vi "Core_Chem_User_Interface_v2.0.vi"() -> ()   [LabVIEW 2014]
uses:
  C:/Program Files (x86)/National Instruments/LabVIEW 2014/examples/Data Communication/Network Streams/Simple Network Streams/support/Network Stream Command.ctl
  <vilib>/dex/Stream Element Allocation Mode.ctl
  <vilib>/Platform/TimedLoop/XDataNode/timing_clust.ctl
  <vilib>/Platform/TimedLoop/XDataNode/nitl_modes.ctl
  <vilib>/Platform/TimedLoop/XDataNode/wakeup.ctl
  <vilib>/Utility/tcp.llb/UDP Multicast Read-Only Open.vi
  <vilib>/platform/TimedLoop/XDataNode/XDataNode.xnode
  <vilib>/Platform/TimedLoop/XDataNode/XDNodeRunTimeDep.lvlib
  <vilib>/FTP/NI_FTP.lvlib
panel:
  out "SO2 Zeroing (Inflight)\nTime Remain (sec)":u32
  in  "eV6 User set time \n(Inflight) (sec)":i32=120
  in  "SO2 Inflight \nZeroing":bool
  out "Create folder error out 2":errorcluster
  out "Network to cRIO live status":bool
  out "Create folder error out":errorcluster
  in  "Confirm Flight Number":bool
  out "PRTAFT_UDP_In":string
  out "TWBOZO01":string
  out "CABOZO01":string
  out "TEIOZO01":string
  out "CHTSOO01":string
  out "CHFGGA01":string
  out "AL52CO01":string
  in  "Flight Number":string
  in  "Tab Control":T1(tab)
  out "FGGA preflight Des 17":string="Preflight - Start minimum 2 hours before take-off\n\n1. Ensure no bags/jackets are stowed on seat backs and behind seats in front of core chemistry rack at all times.\n\n2. Remove inlet covers if applicable.\n\n3. Connect Lilliput mini TFT/LCD VGA cable to FGGA VIDEO (back panel) and PS2 Keyboard/Mouse cables to FGGA Connectors (back panel). TFT/LCD screen kept in WAS/GAS rack Zargers Box. Keyboard/Mouse kept bottom of chemistry rack. (DO NOT disconnect PS2 cable). Connect TFT/LCD AC/DC PSU to 6026-8-98 Amphenol (SSP9) and make 230 Vac CB.\n\n4. Ensure all circuit breakers are pushed in, except 230Vac and 28Vdc, UPS switch off (down) and AL5002 CO Plasma Lamp switch off (down), WoW key to normal (horizontal).\n\n5. Wait for ALL network switches on the aircraft to be up and running before start-up. On the Flight Manager's Interface on the Flight Manager laptop, check SSP icons status (top row) should be all green.  \n\n6. Check AboutTime has synchronised laptop clock to aircraft timeservers (Filiberto/Gaston).\n\nClick the PowerUp Tab."
  out "FGGA preflight Des 16":string="PowerUp\n\n1.\tSSP9 forward face\tMake 3 CBs\n\n2.\tPWRDIST \t\tMake 230Vac CB \n                     Switch UPS On \t[UP]\n                     Make 28Vdc CB\n                     Check 28VDC OK Green Light comes on\n\n3.\tCore Chemistry e-Log\nComplete Core Chemistry e-Log in WordPad (Bnnn_CoreChemLog_v2.2), save on Flight Manager's laptop (192.168.101.180/      flt_folders/Bnnn); Fill in header with date, flight number and your name/initials.\n\n4. Wait for MFM flow rate to display non zero value.\n\n5.\tSAMPUMP\t\t\n - Switch WoW override key (vertical) to check pump starts, and MFM flowrate increase (>20 LPM) on the right hand plot. \n - Switch off WoW override\t\t\t\t [NORM, key horizontal]\n\nClick the 2B Ozone tab if operated, otherwise, click the UDP tab.\n\n\n"
  out "MFM":dbl(graph)
  in  "Ambient = OFF\nCabin = ON":bool
  out "FGGA preflight Des 15":string="2B Ozone Preflight\n\n1.\tSelect either Ambient or Cabin Air mode (default should be OFF for Ambient air mode).\n\n2. Check flowrate is greater than 2000 sccm on the right hand plot.\n\nClick the UDP tab."
  out "2B Ozone concentration":dbl(graph)
  out "2B Ozone flow rate":dbl(graph)
  out "2BOzone Event error out":errorcluster
  out "2BOzone command sender error out":errorcluster
  out "FGGA preflight Des 20":string="4. Check derived parameters in DECADES (192.168.101.110 & 192.168.101.108). 574 Ozone TEi49C; 588 CO AL5002; 611 SO2 TEi43i; 903 - 905 FGGA; 910 / 920 Ozone 2B."
  out "FGGA preflight Des 14":string="UDP Preflight\n1. Check all UDP packets are updating.  Unix time increasing by 1 sec (3rd parameter).\n2. Check flight number is correct.\n3. Confirm flight number and check it appears in the UDP packet (6th parameter). "
  in  "name":string="239.1.4.6"
  in  "Port":u16=50001
  out "FGGA":string
  out "CO":string
  out "TEi49 Ozone":string
  out "2B Cabin Ozone":string
  out "2B Ambient Ozone":string
  out "SO2":string
  out "Ozone Zeroing\nTime Remain (sec)":u32
  in  "Ozone Zeroing":bool
  out "TEI49C Sample Flow B":dbl(graph)
  out "TEi49C Concentration":dbl(graph)
  out "TEI49C Sample Flow A":dbl(graph)
  out "FGGA preflight Des 13":string="TEi49C Ozone PRE-FLIGHT - LAST ACTIONS BEFORE SEAT-BELTING DOWN (PRIOR TO ENGINES START)\n\n1. Ozone monitor zeroing\t\t[10 min minimum]\n\n\n2. Check TEi49C zero value and note down value in e-Log. \n"
  out "FGGA preflight Des 12":string="TEi49C Ozone Preflight\n\n1. Check nominal sample flowrate on both channels is ~0.7 LPM."
  out "Ozone Event error out":errorcluster
  out "Ozone command sender error out":errorcluster
  in  "Ozone UDP Time Offset":i32=1
  out "SO2 react pressure":dbl(graph)
  in  "Prepare SO2 Zero Gas":bool
  in  "Prepare SO2 Span Gas":bool
  in  "Auto Zeroing \ninterval (sec)":i32=600
  out "Next Auto Zero\nStarts in (sec)":u32
  out "Auto Zero\nIndicator":string="Auto Zero Inactive; Manual Zero Allow"
  out "SO2 Resume Zeroing\nCount down timer (sec)":u32
  in  "SO2 Pause\nAuto Zeroing":bool
  out "TEi43i Concentration scaled / raw":cluster{dbl, dbl}(graph)
  in  "SO2 Auto Zeroing":bool
  out "mean zero\ncal status":bool
  out "SO2 Sensitivity":dbl format="%.2g"
  out "SO2 Zero":dbl format="%.2g"
  in  "eV9 Flush User\nset time (sec)":i32=15
  in  "MFC_3 User Set Value":dbl=2.0
  in  "MFC_2 User Set Value":dbl=2.5
  in  "eV6 User\nset time (sec)":i32=600
  out "SO2 Flush\nTime Remain (sec)":u32
  out "TEI43i MFC3 Sample Flow":dbl(graph)
  out "TEI43C Sample Flow":dbl(graph)
  out "TEI43i MFC2 Cal Flow":dbl(graph)
  out "SO2 CAL/Zero\nTime Remain (sec)":u32
  out "SO2 Cal/Zero Flush\nTime Remain (sec)":u32
  in  "SO2 CAL/Zero":bool
  out "FGGA preflight Des 11":string="TEi43 SO2 Inflight Calibration & Zeroing"
  in  "SO2 GND Zeroing":bool
  out "SO2 Zeroing\nTime Remain (sec)":u32
  out "FGGA preflight Des 10":string="TEi43 SO2 PRE-FLIGHT - LAST ACTIONS BEFORE SEAT-BELTING DOWN (PRIOR TO ENGINES START)\n\n1. SO2 monitors zeroing\t\t[10 min minimum]\n\n2. Check TEi43i or TEi43C zero value and note down value in e-Log.\n\n3. Select required SO2 Span/Zero CAL gas at CALDECK front panel using quick connector.\n    For pre- and post-flight SO2 span calibrations select span gas. - Perform SO2 CAL\n    For in-flight SO2 (auto) zeroing, select zero air gas.\n\n4. Enable SO2 auto zeroing (if required) and check zeroing interval. "
  in  "SO2 Flush":bool
  out "FGGA preflight Des 9":string="TEi43 SO2 Preflight\n\n1. Check nominal sample flowrate is 2.0 LPM on the right hand plot.\n\nSO2 calibration gas purge - SO2 calibration cylinder locate at bottom of WAS Gas rack.\n\n2.\n\n\n3. Press SO2 flush button, MFC2 cal flow should increase to 2.5 SLPM.\nMonitor MFC2 flow rate to make sure the reading decreases from 2.5 SLPM to 0.0 SLPM.\nCheck pressure content and delivery gauges also reads zero.\nIf pressure content & delivery gauges do NOT read zero, press SO2 flush button again until they do.\n\n4. Quickly open and close cylinder valve 1.\n\n5. Repeat step 3) to 4) three times.\n\n6. Open cylinder valve 1, system is ready. Note down content pressure in elog.\n\n7."
  in  "eV9 flush User\nset time (sec)":i32=30
  in  "eV8 User\nset time (sec)":i32=60
  out "SO2 Event error out":errorcluster
  out "SO2 command sender \nerror out":errorcluster
  in  "SO2 UDP Time Offset":i32=1
  out "Lamp Temperature":dbl(graph)
  out "CO CAL Status":bool
  in  "CO CAL":bool
  out "FGGA preflight Des 8":string="CO Preflight and Inflight Calibrations\nHold down the CAL button for 2 secs then release, CAL status should then lit up.\nInflight calibration performed on 45 minutes interval or more frequently if lamp temperature > 35.5 degC."
  in  "Prepare Gases":bool
  out "FGGA preflight Des 7":string="AL5002 CO Preflight Checks\n\n1.\n\n2. Start CO Vacuum. NB: If there is problem with the software control, use manual override switch [up] on CALDECK front panel\n\n3. CO Checks - charts on the right hand side\n    Lamp Flow Controller ~ 40 ml/min\n    Monochromator Flow Controller ~ 30 ml/min\n    Fluorescence Cell Pressure ~ 7.5 Torr\n\nIf Lamp/Mono flows are low, manual valves (V1 -> V5) may still be shut, or pressure adjusting valves (ALREG1 & 2) have not been set > 2 bar\n\nIf Cell pressure is 10 Torr (max range), check that COPUMP is running and eV7 is opened (CO Vacuum eV7 is ON).\n\n4. Switch Plasma Lamp at the front panel UP\n\nDetector count rate (on 'Raw Signal' or F2 instrument touchscreen) should increase to >=10000 Hz within a minute.  Recycle plasma lamp switch (off/on) if no significant increase in count rate after 10 mins.  CO concentration should increase (100s ppb). \n     \n\n"
  in  "CO Vaccum (eV7)":bool
  out "Raw Signal":dbl(graph)
  out "CO Concentration":dbl(graph)
  out "Fluorescence Cell Pressure":dbl(graph)
  out "Monochromator Flow":dbl(graph)
  out "Lamp Flow Controller":dbl(graph)
  in  "CO UDP Time Offset":i32=1
  out "CO2 Pressure\nDelivery (PSIA)":dbl(slide) scale=0.0..100.0
  out "Std\nContent (barG)":dbl(slide) scale=0.0..220.0
  out "N2\nContent (barG)":dbl(slide) scale=0.0..220.0
  out "CO2\nContent (barG)":dbl(slide) scale=0.0..170.0
  out "CO Event error out":errorcluster
  out "CO command sender error out":errorcluster
  out "CO Zero":T2(array[cluster])
  out "CO Sensitivity":T3(array[cluster])
  out "Ring Down Time RDA & RDB":cluster{dbl, dbl}(graph)
  in  "Line Lock Setting Change":bool
  out "Cell temperature":dbl(graph)
  out "Cell pressure":dbl(graph)
  in  "Manual FGGA Pump":bool
  out "CO2":dbl(graph)
  out "CH4":dbl(graph)
  out "H2O":dbl(graph)
  out "WoW Flag":string="0"
  in  "FGGA pump\nsync to WoW":bool
  out "CH4 Dry":dbl(graph)
  out "CO2 Dry":dbl(graph)
  out "MFC1 Cal Flow":dbl(graph)
  out "Flush Target Tank\nTime Remain (sec)":u32
  out "Flush Low Tank\nTime Remain (sec)":u32
  out "Flush High Tank\nTime Remain (sec)":u32
  in  "Flush Target Tank":bool
  in  "Flush Low Tank":bool
  in  "Flush High Tank":bool
  in  "FGGA Restart":bool
  out "FGGA preflight Des 6":string="FGGA Instrument Controls"
  in  "High Cal":bool
  out "High Cal\nFlush Time Remain (sec)":u32
  out "High Cal\nCal Time Remain (sec)":u32
  in  "Low Cal":bool
  in  "Target Cal":bool
  in  "Span Cal - \nHigh Cal, CO Cal, Low Cal":bool
  out "Low Cal\nFlush Time Remain (sec)":u32
  out "Low Cal\nCal Time Remain (sec)":u32
  out "Target Cal\nFlush Time Remain (sec)":u32
  out "Target Cal\nCal Time Remain (sec)":u32
  in  "MFC_1 User Set Value":dbl=2.0
  out "FGGA preflight Des 5":string="FGGA Inflight Calibrations"
  out "FGGA preflight Des 4":string="FGGA Ground Preflight Checks\n\n1. Switch FGGA pump ON\n\n2. Check cavity pressure ~50 Torr\n\n3. Switch FGGA pump OFF\n\n4. Enable FGGA pump sync to WoW\n\n5.. Check Time Synchronisation\n\n6. Check CO2 & CH4 values\n\nIf CO2 & CH4 values are -1 ppm, follow the \nchange linelock settings procedure.\n\n\n\n\n\nLAST ACTION BEFORE SEAT-BELTING \nDOWN (PRIOR TO ENGINES START)\n\n1. Disconnect Monitor & stow away. Leave Keyboard & Mouse connected. Place keyboard at the bottom\nof the rack.\n\n"
  out "FGGA preflight Des 3":string="FGGA CAL Gas Purge\n\nFor each cylinder in gas stowage, check that,\n\n1. V1 Closed\n    V3 Closed\n    V4 Make sure arrow positioned downwards (i.e. flow points to gas line)\n\n2. V3 Open (turn anti-clockwise)\n\n3. Use the button on the right according to the operating cylinder to flush the line. Monitor the MFC flow rate to make sure the reading decreases from 3 to zero. (ie fully flushed). Pressure content & delivery gauges should also read zero.\n\n4. V3 Close (turn clockwise)\n\n5. V1 Open / Close quickly\n         Check delivery pressure gauge is ~ 40 PSI \n         (Use V2 to increase if necessary)\n\n6. Repeat steps 2) to 5) three times\n\n7. V3 Close (turn clockwise)\n\n8. V1 Open, check V2 ~ 40 PSIG\n\n9. V3 Open - System is ready"
  out "FGGA command sender error out":errorcluster
  out "FGGA Event Error out":errorcluster
  in  "FGGA UDP Time Offset":i32=1
  in  "FGGA Shutdown":bool
  in  "Postflight Procedures":bool
  in  "FTP ASCII Files to Local":bool
  in  "Transfer FGGA Files":bool
  out "FGGA preflight Des 18":string="Postflight\n\n1. Press the FTP ASCII File to Local button to transfer ASCII files to flight folder.\n\n\n2. Press the Transfer FGGA Files button to transfer FGGA files to flight folder. \n\n\n3. Shutdown FGGA.\n\n\n4. View Postflight Procedures."
  out "File List":string[](array[string])
  out "FGGA File Transfer Error out":errorcluster
  out "Move to FM Error out":errorcluster
  out "USB Disk Space Used %":dbl(slide) scale=0.0..100.0
  out "PTP Sync":bool
  out "CPU Total %":dbl(graph)
  out "PRTAFT_DLU":string
  in  "Pause Auto Zero Count \nDown set time (sec)":i32=600
  out "Calibration gas cylinder \nconcentration (ppb)":dbl format="%.4g"
  in  "Save Calibration gas\ncylinder concentration to file":bool
  in  "Calibration gas cylinder \nconcentration (ppb)":dbl=500.0 format="%.4g"
  in  "Simulate MOCCA Conc":dbl
  in  "MOCCA window \ndelay time (sec)":i32=30
  in  "MOCCA Limit":i32=800
  in  "SO2 Inflight MOCCA Alarm\n(default = OFF)":bool
  in  "Offset Mean Zero Calculation (default = ON)\nOFF = User input\nOn = Mean zero calculated with ev8":bool=TRUE
  out "FGGA preflight Des 19":string="This tab controls ONLY for advanced operators."
  in  "Inst_alm_thresh":i32=220
  in  "3hr_alm_thresh":i32=80
  in  "Simulate Inst Conc":i32
  in  "Simulate 3hr Average Conc":dbl
  in  "Simulate 2B Conc":bool
  in  "Ozone eV6":bool
  in  "Simulate Conc":bool
  in  "8hr TWA Limit":i32=490
  in  "10mins STEL Limit":i32=800
  in  "SO2 Sensitivity":dbl=1.1
  in  "SO2 Zero":dbl
  in  "Simulate TWA Conc":dbl
  in  "Simulate STEL Conc":dbl
  in  "MFC_3\nSLPM Value":dbl=2.0
  in  "MFC_2\nSLPM Value":dbl
  in  "SO2 eV6":bool
  in  "eV8":bool
  in  "eV9":bool
  in  "eV4":bool
  in  "eV3":bool
  in  "MFC_1\nSLPM Value":dbl
  in  "eV2":bool
  in  "eV1":bool
  in  "cRIO File IO Stop\n(USB Flash Drive Unmount)":bool
  # "Unix time"
  # "Flight Number"
  # "concentration (scaled)\npmt_volt\nlamp_volt\nlamp_intens\ninternal_temper\nreact_temper\nreact_press\nflow\nflags\nten_min_so2\neight_hr_so2\nten_min_so2_alm\neight_hr_so2_alm\nMFC_2absolute_pres\nMFC_2temperature\nMFC_2volumetic_flow\nMFC_2mass_flow\nMFC_2set_point\nMFC_3_absolute_pres\nMFC_3_temperature\nMFC_3volumetic_flow\nMFC_3mass_flow\nMFC_3set_point\nV6\nV8\nV9\nMFC2_Set_Value\nMFC3_Set_Value\nconcentration (raw)\nmean calculation status\noffset\nsensitivity\nev8_user_set_time\nauto_zeroing_control\nev8_zero_interval\nMOCCA_inflight_alarm\nMOCCA_time_window_delay\nMOCCA_SO2_limit\n10 min STEL limit\n8 hour TWA limit\nSO2 cal gas cylin conc\nsimulate_SO2_conc_control\nMOCCA_SO2_sim_value\nMOCCA_SO2_alarm"
  # "Unix time"
  # "Unix time"
  # "Unix time"
  # "Unix time"
  # "Flight Number"
  # "Flight Number"
  # "Flight Number"
  # "Flight Number"
  # "conc\ntemp\npress\nflow\nthreehr_oz\nInst_alarm\nthreehr_alarm"
  # "ch4\nco2\nh2o\npress_torr\ntemp_c\nfit_flag\nrda_usec\nrdb_usec\nch4_dry\nco2_dry\nMFC_1_absolute_pres\nMFC_1_temperature\nMFC_1volumetic_flow\nMFC_1mass_flow\nMFC_1set_point\nV1\nV2\nV3\nV4\nrestart_FGGA\nFGGA_Pump\nCAL_MFC_1Set_Value"
  # "conc\ntemp\npress\nflow"
  # "conc\nbenchtemp\npress\ncellAint\ncellBint\nFlowA\nFlowB\nlamptemp\nflag\nV6"
  # "conc\ncounts\nsens\nzero\nlampflow\nlamptemp\nmonoflow\nmonotemp\nmonopress\ncellpress\ncalpress\ntemppmt\ncalconc\nerr\ncal_counter\nerr_counter\nCO_vacuum_status\nIn_Cal\nALEG1_press_delivery\nALREG1_press_content\nALREG2_press_content\nALREG3_press_content"
  # "TEi43c"
  # "TEi43i"
  # "SO2 CAL / ZERO\nSETTINGS"
  # "FGGA"
  # "2B Ozone"
  # "TEi49C  - Ozone"
  # "TEi43 - SO2"
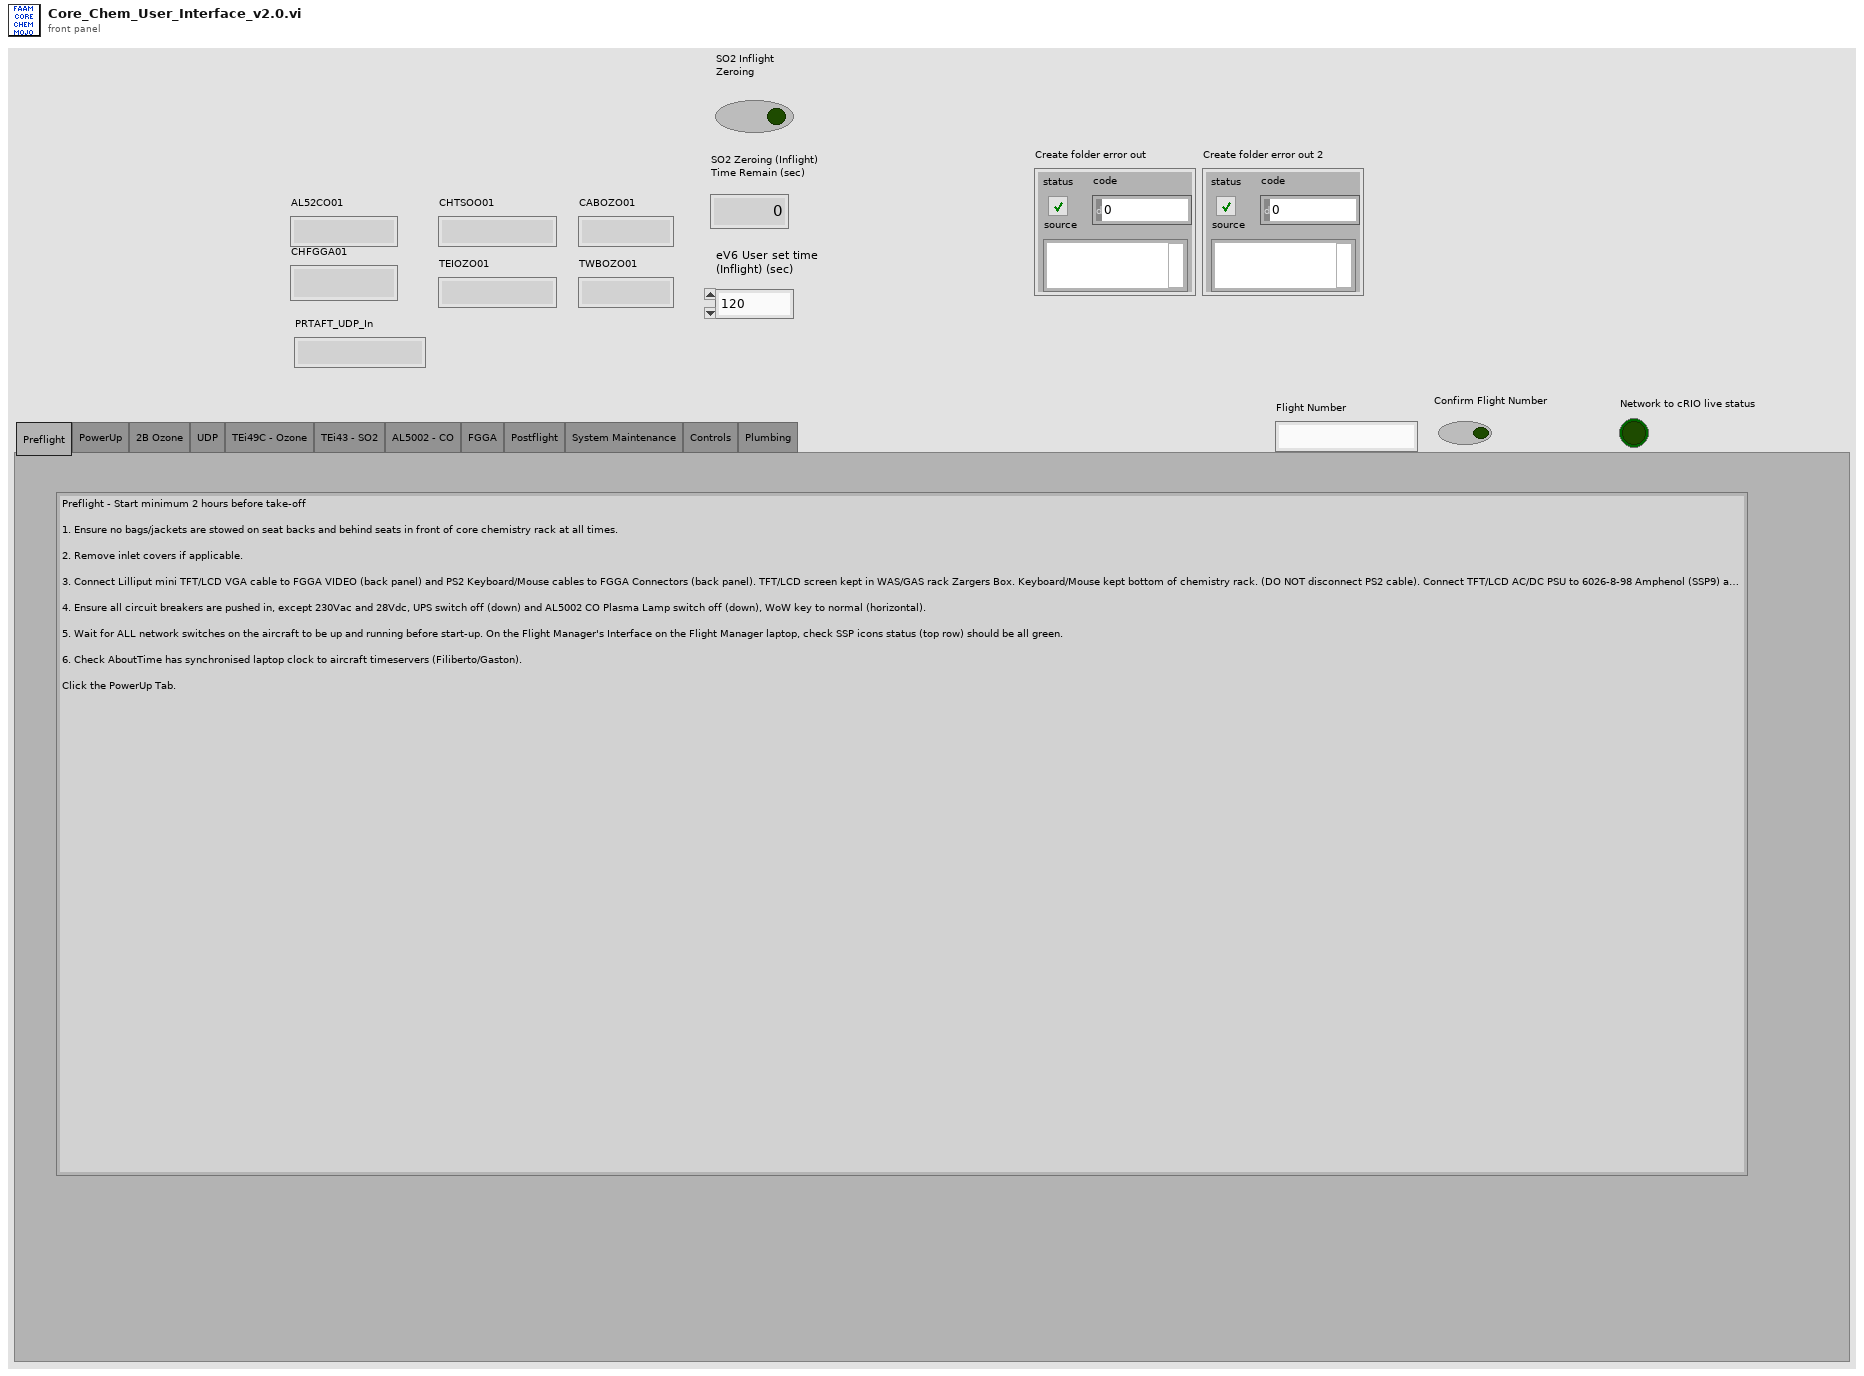
[diagram p1: front panel]
types:
  T1 = enum32{"Preflight", "PowerUp", "2B Ozone", "UDP", "TEi49C - Ozone", "TEi43 - SO2", "AL5002 - CO", "FGGA", "Postflight", "System Maintenance", "Controls", "Plumbing"}
  T2 = cluster{"time stamp":timestamp, "CO Offset":dbl}[]
  T3 = cluster{"time stamp":timestamp, "CO Sensitivity":dbl}[]
  T4 = typedef "Network Stream Command.ctl" = cluster{"Message":string, "Message Data":variant}
  T5 = typedef "Stream Element Allocation Mode.ctl" = u32
  T6 = typedef "XDNodeRunTimeDep.lvlib/timing_clust.ctl" = cluster{"Expected End [f-1]":u64, "Actual End [f-1]":u64, "Finished Late? [f-1]":bool, "Expected End [i-1]":u64, "Actual End [i-1]":u64, "Finished Late? [i-1]":bool, "Expected Start [i]":u64, "Actual Start [i]":u64, "Expected Start [f]":u64, "Actual Start [f]":u64, "Source Name":string, "Structure Name":string, "Period":i64, "Deadline":i64, "Offset":i64, "Start":i64, "Priority":i32, "Timeout":i32, "Mode":T7, "Wakeup Reason":T8, "Error":errorcluster, "Source Type":string, "Secondary Source Type":string, "Global End Time":u64, "Global Start Time":u64, "Frame Duration":u64, "Iteration Duration":u64, "Assigned CPU":i32, "I/O Scan Engine Mode":u32}
  T7 = typedef "XDNodeRunTimeDep.lvlib/nitl_modes.ctl" = enum32{"No Change", "Process missed periods, maintain original phase", "Discard missed periods, maintain original phase", "Process missed periods, ignore original phase", "Discard missed periods, ignore original phase"}
  T8 = typedef "XDNodeRunTimeDep.lvlib/wakeup.ctl" = enum32{"Normal", "Aborted", "Asynchronous wakeup", "Timing source error", "Timed loop error", "Timeout"}
  T9 = typedef "NI_FTP.lvlib/FTP Session.ctl" = refnum<k5>
  T10 = typedef "NI_FTP.lvlib/FTP File Info.ctl" = cluster{"type":enum16{"unknown", "file", "dir", "link"}, "permissions":string, "owner":string, "group":string, "size":i32, "date":string, "name":string, "link name":string}
  T11 = cluster{"Message":string, "Message 2":string, "Message 3":string}
  T12 = cluster{"Message":string, "Message 2":string, "Message 3":string, "Message 4":string}
  T13 = cluster{"Message":string, "Message 3":string, "Message 4":string}
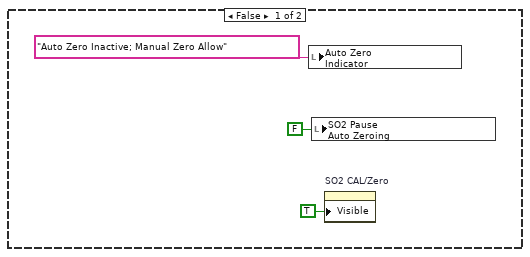
[diagram p4: hidden frame]
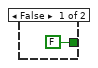
[diagram p17: hidden frame]
diagram:
  w6 = "XXXX"
  w9 = 0
  w10 = 0.0
  w16 = T4 {"Message"="", "Message Data"=variant} ("Message Cluster")
  w22 = T5 0 items=["allocate as needed", "pre-allocate"] ("element allocation mode")
  w28 = T4 {"Message"="", "Message Data"=variant} ("Message Cluster")
  w34 = T5 0 items=["allocate as needed", "pre-allocate"] ("element allocation mode")
  w39 = T4 {"Message"="", "Message Data"=variant} ("Message Cluster")
  w44 = T5 0 items=["allocate as needed", "pre-allocate"] ("element allocation mode")
  w53 = T5 0 items=["allocate as needed", "pre-allocate"] ("element allocation mode")
  w55 = T4 {"Message"="", "Message Data"=variant} ("Message Cluster")
  w62 = T5 0 items=["allocate as needed", "pre-allocate"] ("element allocation mode")
  w64 = T4 {"Message"="", "Message Data"=variant} ("Message Cluster")
  n1 = local write "cRIO File IO Stop\n(USB Flash Drive Unmount)"(FALSE ("Stop File Write")) -> ()
  n2 = local write "Flight Number"(w6) -> ()
  n3 = while {
    shift-right: [w68] -> _
    shift-left: w6 -> [w67]
    stop <- FALSE stop-if-true
    n4 = Not Equal?(x=w67, y="Flight Number") -> (x != y?=w70:bool)
    n5 = case shown="True" w70 {
      tunnel: [w73 w74] -> w68
      tunnel: "Flight Number" -> [_ w74]
      tunnel: w67 -> [w73 _]
      frame False {
      }
      frame True {
        n6 = One Button Dialog(message="Flight Number changed,\nPress flight number button to confirm") -> ()  [unwired: 1 in, 1 out]
      }
    }
    n7 = Wait (ms)(milliseconds to wait=u32 1000) -> ()  [unwired: 1 out]
  }
  n8 = while {
    stop <- FALSE stop-if-true
    # "UDP Read"
    n9 = String To IP(1:"name") -> (0:w81:u32)
    n10 = call-poly <vilib>:"UDP Multicast Open.vi"("multicast addr"=w81, "port"="Port") -> ("error out"=w79:errorcluster, "connection ID"=w78:refnum<k16>)  [unwired: 7 in, 1 out]
    n11 = Wait (ms)(milliseconds to wait=u32 1000) -> ()  [unwired: 1 out]
    n12 = case shown="No Error" w79 {
      selector: w79 -> [w85 _]
      tunnel: w78 -> [w84 _]
      frame No Error {
        w83 = ""
        n13 = while {
          tunnel: w85 -> [w131]
          tunnel: w84 -> [w130]
          shift-right: [w126] -> _
          shift-left: w83 -> [w127]
          shift-right: [w117] -> _
          shift-left: w83 -> [w119]
          shift-right: [w111] -> _
          shift-left: w83 -> [w113]
          shift-right: [w105] -> _
          shift-left: w83 -> [w106]
          shift-right: [w99] -> _
          shift-left: w83 -> [w100]
          shift-right: [w93] -> _
          shift-left: w83 -> [w94]
          shift-right: [w87] -> _
          shift-left: w83 -> [w88]
          stop <- w129 stop-if-true
          n14 = UDP Read(connection ID=w130, 8:w131) -> (data out=w86:string, error out=w129:errorcluster)  [unwired: 2 in, 3 out]
          n15 = Match Pattern(string=w86, regular expression="$TEIOZO01,") -> (match substring=w125:string, after substring=w124:string)  [unwired: 1 in, 2 out]
          n16 = Match Pattern(string=w86, regular expression="$TWBOZO01,") -> (match substring=w103:string, after substring=w102:string)  [unwired: 1 in, 2 out]
          n17 = Match Pattern(string=w86, regular expression="$CABOZO01,") -> (match substring=w109:string, after substring=w108:string)  [unwired: 1 in, 2 out]
          n18 = Match Pattern(string=w86, regular expression="$CHTSOO") -> (match substring=w97:string, after substring=w96:string)  [unwired: 1 in, 2 out]
          n19 = Match Pattern(string=w86, regular expression="$CHFGGA01,") -> (match substring=w121:string, after substring=w120:string)  [unwired: 1 in, 2 out]
          n20 = Match Pattern(string=w86, regular expression="$AL52CO01,") -> (match substring=w115:string, after substring=w114:string)  [unwired: 1 in, 2 out]
          n21 = Match Pattern(string=w86, regular expression="$PRTAFT01,") -> (match substring=w92:string, after substring=w91:string)  [unwired: 1 in, 2 out]
          n22 = Concatenate Strings(w125, w124) -> (w123:string)
          n23 = Concatenate Strings(w103, w102) -> (w101:string)
          n24 = Concatenate Strings(w109, w108) -> (w107:string)
          n25 = Concatenate Strings(w97, w96) -> (w95:string)
          n26 = Concatenate Strings(w121, w120) -> (w118:string)
          n27 = Concatenate Strings(w115, w114) -> (w112:string)
          n28 = Concatenate Strings(w92, w91) -> (w89:string)
          n29 = Replace Substring(4:w101, 5:w100) -> (1:w99:string)  [unwired: 2 in, 1 out]
          "TWBOZO01" <- w99
          n30 = Replace Substring(4:w123, 5:w127) -> (1:w126:string)  [unwired: 2 in, 1 out]
          "TEIOZO01" <- w126
          n31 = Replace Substring(4:w107, 5:w106) -> (1:w105:string)  [unwired: 2 in, 1 out]
          "CABOZO01" <- w105
          n32 = Replace Substring(4:w95, 5:w94) -> (1:w93:string)  [unwired: 2 in, 1 out]
          "CHTSOO01" <- w93
          n33 = Replace Substring(4:w112, 5:w113) -> (1:w111:string)  [unwired: 2 in, 1 out]
          "AL52CO01" <- w111
          n34 = Replace Substring(4:w118, 5:w119) -> (1:w117:string)  [unwired: 2 in, 1 out]
          "CHFGGA01" <- w117
          n35 = Replace Substring(4:w89, 5:w88) -> (1:w87:string)  [unwired: 2 in, 1 out]
          "PRTAFT_UDP_In" <- w87
        }
      }
      frame Error {
      }
    }
  }
  n36 = Obtain Queue(name (unnamed)="CO_Command", element data type=w64) -> (queue out=w15:refnum<queue>, error out=w58:errorcluster)  [unwired: 3 in, 1 out]
  n37 = Create Network Stream Writer Endpoint(6:w62, 7:10 ("writer buffer size"), 9:w64, 10:"//192.168.101.17/command/reader/CO" ("reader url"), 11:"/command/writer/CO" ("writer name")) -> (0:w61:errorcluster, 3:w60:refnum<k21>)  [unwired: 2 in]
  n38 = while {
    tunnel: w15 -> [w135]
    tunnel: w58 -> [w134]
    tunnel: [w132] -> _
    stop <- FALSE stop-if-true
    # "CO UI Event Handler Loop"
    n39 = event shown="[4] \"Confirm Flight Number\": Value Change" {
      selector: _ -> [_ _ _ _ _]
      dyn-events: _ -> [_ _ _ _ _]
      timeout: _ -> [_ _ _ _ _]
      tunnel: w135 -> [w142 w149 w153 w160 w168]
      tunnel: w134 -> [w141 w148 w152 w159 w167]
      tunnel: [w136 w143 w151 w158 w166] -> w132
      event "CO CAL": Value Change {
        n40 = event-data() -> ("NewVal"=w139:bool)  [unwired: 1 in]
        n41 = Bundle(cluster=T4 {"Message"="", "Message Data"=variant} ("Message Cluster"), "Message"="CO CAL", "Message Data"=w139) -> (w137:T4)
        n42 = Enqueue Element(queue=w142, element=w137, error in (no error)=w141) -> (error out=w136:errorcluster)  [unwired: 1 in, 2 out]
      }
      event "CO UDP Time Offset": Value Change {
        n43 = event-data() -> ("NewVal"=w146:i32)  [unwired: 1 in]
        n44 = Bundle(cluster=T4 {"Message"="", "Message Data"=variant} ("Message Cluster"), "Message"="UDP Time Offset", "Message Data"=w146) -> (w144:T4)
        n45 = Enqueue Element(queue=w149, element=w144, error in (no error)=w148) -> (error out=w143:errorcluster)  [unwired: 1 in, 2 out]
      }
      event "CO Vaccum (eV7)": Value Change {
        n46 = event-data() -> ("NewVal"=w150:bool)  [unwired: 1 in]
        n47 = Bundle(cluster=T4 {"Message"="", "Message Data"=variant} ("Message Cluster"), "Message"="CO Vacuum", "Message Data"=w150) -> (w154:T4)
        n48 = Enqueue Element(queue=w153, element=w154, error in (no error)=w152) -> (error out=w151:errorcluster)  [unwired: 1 in, 2 out]
      }
      event "cRIO File IO Stop\n(USB Flash Drive Unmount)": Value Change {
        n49 = event-data() -> ("NewVal"=w157:bool)  [unwired: 1 in]
        n50 = Bundle(cluster=T4 {"Message"="", "Message Data"=variant} ("Message Cluster"), "Message"="Stop File Write", "Message Data"=w157) -> (w161:T4)
        n51 = Enqueue Element(queue=w160, element=w161, error in (no error)=w159) -> (error out=w158:errorcluster)  [unwired: 1 in, 2 out]
      }
      event "Confirm Flight Number": Value Change {
        n52 = event-data() -> ()  [unwired: 1 in, 1 out]
        n53 = flat-sequence {
          tunnel: w167 -> [w170]
          tunnel: w168 -> [w171]
          tunnel: [w171] -> w165
          tunnel: [w170] -> w164
          tunnel: [w173] -> w166
          tunnel: w165 -> [w175]
          tunnel: w164 -> [w174]
          frame #0 {
            n54 = local write "cRIO File IO Stop\n(USB Flash Drive Unmount)"(FALSE ("cRIO File IO Stop\n(USB Flash Drive Unmount)")) -> ()
          }
          frame #1 {
            n55 = local read "Flight Number"() -> (w172:string)
            n56 = Bundle(cluster=T4 {"Message"="", "Message Data"=variant} ("Message Cluster"), "Message"="Flight Number", "Message Data"=w172) -> (w176:T4)
            n57 = Enqueue Element(queue=w175, element=w176, error in (no error)=w174) -> (error out=w173:errorcluster)  [unwired: 1 in, 2 out]
          }
        }
      }
    }
    "CO Event error out" <- w132
  }
  n58 = while {
    tunnel: w15 -> [w186]
    shift-right: [w181] -> _
    shift-left: w60 -> [w183]
    shift-right: [w179] -> w49
    shift-left: w61 -> [w185]
    tunnel: w58 -> [w180]
    stop <- w179 stop-if-true
    # "CO UI Command Sender"
    n59 = Dequeue Element(queue=w186, error in (no error)=w180) -> (element=w182:T4)  [unwired: 1 in, 3 out]
    n60 = Unbundle By Name(w182) -> ("Message"=w184:string)
    n61 = case shown="\"UDP Time Offset\"" w184 {
      tunnel: w185 -> [w187 w191 w198 w205 w212 w219]
      tunnel: w183 -> [w188 w194 w201 w208 w215 w222]
      tunnel: w182 -> [_ w193 w200 w207 w214 w221]
      tunnel: [w187 w190 w197 w204 w211 w218] -> w179
      tunnel: [w188 w189 w196 w203 w210 w217] -> w181
      frame "False", Default {
      }
      frame "CO CAL" {
        n62 = shared-variable-write(w194, w191, w193) -> (w192:refnum<k21>, w195:errorcluster)  [unwired: 1 in, 1 out]
        n63 = Flush Stream(8:w195, 11:w192) -> (0:w190:errorcluster, 3:w189:refnum<k21>)  [unwired: 2 in, 1 out]
      }
      frame "UDP Time Offset" {
        n64 = shared-variable-write(w201, w198, w200) -> (w199:refnum<k21>, w202:errorcluster)  [unwired: 1 in, 1 out]
        n65 = Flush Stream(8:w202, 11:w199) -> (0:w197:errorcluster, 3:w196:refnum<k21>)  [unwired: 2 in, 1 out]
      }
      frame "Stop File Write" {
        n66 = shared-variable-write(w208, w205, w207) -> (w206:refnum<k21>, w209:errorcluster)  [unwired: 1 in, 1 out]
        n67 = Flush Stream(8:w209, 11:w206) -> (0:w204:errorcluster, 3:w203:refnum<k21>)  [unwired: 2 in, 1 out]
      }
      frame "Flight Number" {
        n68 = shared-variable-write(w215, w212, w214) -> (w213:refnum<k21>, w216:errorcluster)  [unwired: 1 in, 1 out]
        n69 = Flush Stream(8:w216, 11:w213) -> (0:w211:errorcluster, 3:w210:refnum<k21>)  [unwired: 2 in, 1 out]
      }
      frame "CO Vacuum" {
        n70 = shared-variable-write(w222, w219, w221) -> (w220:refnum<k21>, w223:errorcluster)  [unwired: 1 in, 1 out]
        n71 = Flush Stream(8:w223, 11:w220) -> (0:w218:errorcluster, 3:w217:refnum<k21>)  [unwired: 2 in, 1 out]
      }
    }
  }
  "CO command sender error out" <- w49
  n72 = node-c288() -> (w14:T6)  [unwired: 4 in]
  n73 = Initialize Array(cluster{"time stamp":timestamp, "Y":dbl} {"time stamp"=timestamp(0 s since 1904-01-01), "Y"=0.0}, 30 ("dimension size")) -> (w11:cluster{"time stamp":timestamp, "Y":dbl}[])
  n74 = timed-loop {
    timing: w14 -> [_]
    timing-out: [_] -> w13
    stop <- _ stop-if-true
    # "PC Tasks"
    n75 = node-c288() -> ()  [unwired: 1 in, 1 out]
    n76 = event shown="[0] \"FTP ASCII Files to Local\": Value Change" {
      selector: _ -> [_ _ _ _]
      dyn-events: _ -> [_ _ _ _]
      timeout: _ -> [_ _ _ _]
      event "FTP ASCII Files to Local": Value Change {
        n77 = event-data() -> ()  [unwired: 1 in, 1 out]
        n78 = flat-sequence {
          tunnel: [w232] -> w226
          tunnel: [w244] -> w231
          tunnel: [w243] -> w229
          tunnel: [w242] -> w227
          tunnel: w226 -> [w242]
          tunnel: w231 -> [w302]
          tunnel: [w302] -> w230
          tunnel: w229 -> [w298]
          tunnel: [w297] -> w228
          tunnel: w227 -> [w297]
          tunnel: w230 -> [w308]
          tunnel: w228 -> [w303]
          frame #0 {
            n79 = local read "Flight Number"() -> (w234:string)
            n80 = Concatenate Strings("Confirm Flight Number" ("message"), "\n", w234) -> (w238:string)
            n81 = Two Button Dialog(message=w238, 1:"No" ("F button name (\"Cancel\")"), 2:"Yes" ("T button name (\"OK\")")) -> (T button?=w235:bool)
            n82 = case shown="False" w235 {
              tunnel: w234 -> [_ w241]
              tunnel: [w240 w241] -> w232
              frame False {
                n83 = call "Prompt User for Flight Number2"() -> ("Flight Number BXXX"=w240:string)  [unwired: 17 in, 2 out]
              }
              frame True {
              }
            }
          }
          frame #1 {
            n84 = Get Date/Time In Seconds() -> (seconds since 1Jan1904=w248:timestamp)
            n85 = Format Date/Time String(time format string (%c)="%Y%m%d", seconds (now)=w248) -> (date/time string=w246:string)  [unwired: 1 in]
            n86 = call <vilib>:"FTP Open Session.vi"("address"="192.168.101.17") -> ("error out"=w263:errorcluster, "ftp session"=w264:T9)  [unwired: 7 in, 2 out]
            n87 = Concatenate Strings("Use Today's Date" ("message"), "\r", w246) -> (w252:string)
            n88 = call <vilib>:"FTP Logon.vi"("error in (no error)"=w263, "password"="", "user"="anonymous", "ftp session"=w264) -> ("error out"=w260:errorcluster, "ftp session out"=w259:T9)  [unwired: 4 in, 2 out]
            n89 = Two Button Dialog(message=w252, 1:"No" ("F button name (\"Cancel\")"), 2:"Yes" ("T button name (\"OK\")")) -> (T button?=w249:bool)
            n90 = case shown="False" w249 {
              tunnel: [w267 w268] -> w243
              tunnel: w246 -> [_ w268]
              frame False {
                n91 = call "Prompt User for Date"() -> ("Date"=w267:string)  [unwired: 17 in, 2 out]
              }
              frame True {
              }
            }
            n92 = call <vilib>:"FTP Directory Listing.vi"("error in (no error)"=w260, "directory path"="/U:/data", "ftp session"=w259) -> ("dir list"=w258:T10[])  [unwired: 4 in, 4 out]
            n93 = for {
              tunnel: w258 -> [w288] mode=indexing
              tunnel: [w287] -> w255 mode=indexing
              tunnel: w243 -> [w286]
              # "Extract File Name According to the Date"
              n94 = Unbundle By Name(w288) -> ("name"=w294:string, "name"=w293:string)
              n95 = Match Pattern(string=w293, regular expression="_[0-9]+") -> (match substring=w291:string)  [unwired: 1 in, 3 out]
              n96 = String Subset(string=w291, offset (0)=1) -> (substring=w289:string)  [unwired: 1 in]
              n97 = Equal?(x=w289, y=w286) -> (x = y?=w295:bool)
              n98 = case shown="False" w295 {
                tunnel: w294 -> [_ w296]
                tunnel: [_ w296] -> w287
                frame False {
                }
                frame True {
                }
              }
            }
            n99 = Array Size(array=w255) -> (size(s)=w257:i32)
            n100 = for {
              N: w257 -> [_]
              shift-right: [w275] -> w245
              shift-left: w255 -> [w276]
              shift-right: [w273] -> _
              shift-left: 0 -> [w274]
              # "Remove Empty Array"
              n101 = Index Array(array=w276, index=w274) -> (element=w278:string)
              n102 = Equal?(x=w278, y="") -> (x = y?=w277:bool)
              n103 = case shown="True" w277 {
                tunnel: w276 -> [w282 w285]
                tunnel: w274 -> [w281 w283]
                tunnel: [w282 w284] -> w275
                tunnel: [w280 w283] -> w273
                frame False {
                  n104 = Increment(x=w281) -> (x+1=w280:i32)
                }
                frame True {
                  n105 = Delete From Array(array=w285, index=w283) -> (array with subset deleted=w284:string[])  [unwired: 1 in, 1 out]
                }
              }
            }
            "File List" <- w245
            n106 = for {
              tunnel: w245 -> [w271] mode=indexing
              tunnel: [w269] -> w244 mode=indexing
              # "Specify destination path for each file"
              n107 = Concatenate Strings("C:\\temp\\", w271) -> (w270:string)
              n108 = String To Path(string=w270) -> (path=w269:path)
            }
          }
          frame #2 {
            # "FTP a list of files"
            n109 = call <vilib>:"System Exec.vi"("wait until completion? (T)"=TRUE, "working directory"=path "C:/temp", "standard input"=w298, "command line"="C:\\temp\\transfer_ascii_files.bat") -> ()  [unwired: 4 in, 4 out]
          }
          frame #3 {
            # "Move file from local PC to Flight Folder"
            n110 = Build Path(base path=path "\\\\192.168.101.180\\flt_folders" ("path"), name or relative path=w303) -> (appended path=w310:path)
            n111 = Concatenate Strings(w303, "_" ("string"), "corechem" ("string")) -> (w309:string)
            n112 = Build Path(base path=w310, name or relative path=w309) -> (appended path=w305:path)
            n113 = Create Folder(path (use dialog)=w305) -> (created path=w304:path, error out=→"Create folder error out 2":errorcluster)  [unwired: 2 in, 1 out]
            n114 = for {
              tunnel: w304 -> [w317]
              tunnel: [w316] -> w307
              tunnel: w308 -> [w314] mode=indexing
              n115 = Copy(9:TRUE ("overwrite (F)"), 10:w317, 11:w314) -> (0:w316:errorcluster)  [unwired: 2 in, 2 out]
            }
            "Move to FM Error out" <- w307
          }
          frame #4 {
            n116 = local write "FTP ASCII Files to Local"(FALSE ("FTP Files to Local")) -> ()
          }
        }
      }
      event "Transfer FGGA Files": Value Change {
        n117 = event-data() -> ()  [unwired: 1 in, 6 out]
        n118 = flat-sequence {
          tunnel: [w323] -> w322
          tunnel: w322 -> [w335]
          tunnel: [w335] -> w321
          tunnel: [w334] -> w320
          tunnel: [w333] -> w319
          tunnel: w321 -> [w345]
          tunnel: w320 -> [w344]
          tunnel: w319 -> [w346]
          frame #0 {
            n119 = local read "Flight Number"() -> (w324:string)
            n120 = Concatenate Strings("Confirm Flight Number" ("message"), "\n", w324) -> (w326:string)
            n121 = Two Button Dialog(message=w326, 1:"No" ("F button name (\"Cancel\")"), 2:"Yes" ("T button name (\"OK\")")) -> (T button?=w330:bool)
            n122 = case shown="False" w330 {
              tunnel: w324 -> [_ w332]
              tunnel: [w331 w332] -> w323
              frame False {
                n123 = call "Prompt User for Flight Number"() -> ("Flight Number BXXX"=w331:string)  [unwired: 17 in, 2 out]
              }
              frame True {
              }
            }
          }
          frame #1 {
            n124 = Two Button Dialog(message="Get FGGA Files\nof Today's Date?", 1:"No" ("F button name (\"Cancel\")"), 2:"Yes" ("T button name (\"OK\")")) -> (T button?=w339:bool)
            n125 = case shown="False" w339 {
              selector: w339 -> [w341 w342]
              tunnel: [w341 w342] -> w333
              tunnel: [w340 _] -> w334
              frame False {
                n126 = call "Prompt User for Date"() -> ("Date"=w340:string)  [unwired: 17 in, 2 out]
              }
              frame True {
              }
            }
          }
          frame #2 {
            n127 = Build Path(base path=path "\\\\192.168.101.180\\flt_folders" ("path"), name or relative path=w345) -> (appended path=w350:path)
            n128 = Concatenate Strings(w345, "_" ("string"), "corechem" ("string")) -> (w349:string)
            n129 = Build Path(base path=w350, name or relative path=w349) -> (appended path=w343:path)
            n130 = Create Folder(path (use dialog)=w343) -> (error out=→"Create folder error out":errorcluster)  [unwired: 2 in, 2 out]
            n131 = call "labSSH_FGGA_Files_Transfer.vi"("Flight_num"=w345, "Get current?"=w346, "Date"=w344, "Flight Folder Path"=w343) -> ("error IO"=→"FGGA File Transfer Error out":errorcluster)  [unwired: 11 in]
          }
          frame #3 {
            n132 = local write "Transfer FGGA Files"(FALSE) -> ()
          }
        }
      }
      event "FGGA Restart": Value Change {
        n133 = event-data() -> ()  [unwired: 1 in, 6 out]
        n134 = flat-sequence {
          frame #0 {
            n135 = Two Button Dialog(message="FGGA will be restarted,\nARE YOU SURE?") -> (T button?=w356:bool)  [unwired: 2 in]
            n136 = case shown="True" w356 {
              frame False {
              }
              frame True {
                n137 = call "labSSH_Commands.vi"("Data"="reboot") -> ()  [unwired: 14 in, 1 out]
              }
            }
          }
          frame #1 {
            n138 = local write "FGGA Restart"(FALSE ("FGGA Restart")) -> ()
          }
        }
      }
      event "FGGA Shutdown": Value Change {
        n139 = event-data() -> ()  [unwired: 1 in, 6 out]
        n140 = flat-sequence {
          frame #0 {
            n141 = Two Button Dialog(message="FGGA will be shutdown,\nARE YOU SURE?") -> (T button?=w360:bool)  [unwired: 2 in]
            n142 = case shown="True" w360 {
              frame False {
              }
              frame True {
                n143 = call "labSSH_Commands.vi"("Data"="halt") -> ()  [unwired: 14 in, 1 out]
              }
            }
          }
          frame #1 {
            n144 = local write "FGGA Shutdown"(FALSE ("FGGA Restart")) -> ()
          }
        }
      }
    }
    n145 = node-c288() -> ()  [unwired: 1 in, 1 out]
  }
  n146 = while {
    shift-right: [w488] -> _
    shift-left: w10 -> [w486]
    shift-right: [w490] -> _
    shift-left: w9 -> [w491]
    shift-right: [w489] -> _
    shift-left: w11 -> [w493]
    shift-right: [w482] -> _
    shift-left: w11 -> [w484]
    shift-right: [w479] -> _
    shift-left: w10 -> [w478]
    shift-right: [w481] -> _
    shift-left: w9 -> [w483]
    shift-right: [w475] -> _
    shift-left: FALSE -> [w476]
    stop <- FALSE stop-if-true
    w422 = ""
    w417 = "%s" ("format string")
    w610 = "%s" ("format string")
    w615 = "%s" ("format string")
    w620 = "%s" ("format string")
    w626 = "%s" ("format string")
    w632 = "%s" ("format string")
    w636 = "%s" ("format string")
    # "UDP Data Processing"
    n147 = local read "CHFGGA01"() -> (w639:string)
    n148 = local read "TWBOZO01"() -> (w614:string)
    n149 = local read "AL52CO01"() -> (w631:string)
    n150 = local read "CABOZO01"() -> (w619:string)
    n151 = local read "TEIOZO01"() -> (w625:string)
    n152 = local read "CHTSOO01"() -> (w609:string)
    n153 = local read "Ambient = OFF\nCabin = ON"() -> (w514:bool)
    n154 = Spreadsheet String To Array(delimiter (Tab)=",", format string=w636, spreadsheet string=w639, array type (2D Dbl)=string[] []) -> (array=w586:string[])
    n155 = Spreadsheet String To Array(delimiter (Tab)=",", format string=w632, spreadsheet string=w631, array type (2D Dbl)=string[] []) -> (array=w607:string[])
    n156 = Spreadsheet String To Array(delimiter (Tab)=",", format string=w620, spreadsheet string=w619, array type (2D Dbl)=string[] []) -> (array=w511:string[])
    n157 = Spreadsheet String To Array(delimiter (Tab)=",", format string=w626, spreadsheet string=w625, array type (2D Dbl)=string[] []) -> (array=w584:string[])
    n158 = Spreadsheet String To Array(delimiter (Tab)=",", format string=w615, spreadsheet string=w614, array type (2D Dbl)=string[] []) -> (array=w510:string[])
    n159 = Spreadsheet String To Array(delimiter (Tab)=",", format string=w610, spreadsheet string=w609, array type (2D Dbl)=string[] []) -> (array=w582:string[])
    n160 = Array To Spreadsheet String(delimiter (Tab)="\r", array=w586, 3:w636) -> (spreadsheet string=→"FGGA":string)
    n161 = Array To Spreadsheet String(delimiter (Tab)="\r", array=w607, 3:w632) -> (spreadsheet string=→"CO":string)
    n162 = Array To Spreadsheet String(delimiter (Tab)="\r", array=w511, 3:w620) -> (spreadsheet string=→"2B Cabin Ozone":string)
    n163 = Array To Spreadsheet String(delimiter (Tab)="\r", array=w584, 3:w626) -> (spreadsheet string=→"TEi49 Ozone":string)
    n164 = Array To Spreadsheet String(delimiter (Tab)="\r", array=w510, 3:w615) -> (spreadsheet string=→"2B Ambient Ozone":string)
    n165 = Array To Spreadsheet String(delimiter (Tab)="\r", array=w582, 3:w610) -> (spreadsheet string=→"SO2":string)
    n166 = Select(t=w511, s=w514, f=w510) -> (s? t:f=w509:string[])
    n167 = Index Array(array=w582, index #1=6 ("index"), index #2=4 ("index"), index #3=3 ("index"), index #4=7 ("index"), index #5=8 ("index"), index #6=15 ("index"), index #7=24 ("index"), index #8=29 ("index"), index #9=36 ("index"), index #10=37 ("index"), index #11=38 ("index"), index #12=39 ("index"), index #13=48 ("index"), index #14=14 ("index")) -> (element #1=w501:string, element #2=w565:string, element #3=w560:string, element #4=w553:string, element #5=w529:string, element #6=w528:string, element #7=w440:string, element #8=w439:string, element #9=w386:string, element #10=w382:string, element #11=w378:string, element #12=w376:string, element #13=w368:string, element #14=w366:string)
    n168 = Index Array(array=w509, index #1=8 ("index"), index #2=11 ("index")) -> (element #1=w503:string, element #2=w504:string)
    n169 = Index Array(array=w584, index #1=6 ("index"), index #2=4 ("index"), index #3=3 ("index"), index #4=7 ("index"), index #5=9 ("index"), index #6=14 ("index"), index #7=15 ("index")) -> (element #1=w578:string, element #2=w566:string, element #3=w561:string, element #4=w546:string, element #5=w520:string, element #6=w519:string, element #7=w518:string)
    n170 = Scan Value(string=w503, format string="%f") -> (value=→"2B Ozone concentration":dbl)  [unwired: 1 in, 1 out]
    n171 = Scan Value(string=w504, format string="%4f") -> (value=→"2B Ozone flow rate":dbl)  [unwired: 1 in, 1 out]
    n172 = Index Array(array=w586, index #1=6 ("index"), index #2=4 ("index"), index #3=3 ("index"), index #4=7 ("index"), index #5=8 ("index"), index #6=9 ("index"), index #7=10 ("index"), index #8=17 ("index"), index #9=16 ("index"), index #10=11 ("index"), index #11=12 ("index"), index #12=21 ("index"), index #13=14 ("index"), index #14=15 ("index")) -> (element #1=w580:string, element #2=w568:string, element #3=w563:string, element #4=w548:string, element #5=w464:string, element #6=w461:string, element #7=w456:string, element #8=w454:string, element #9=w451:string, element #10=w446:string, element #11=w445:string, element #12=w432:string, element #13=w396:string, element #14=w395:string)
    n173 = Index Array(array=w607, index #1=2 ("index"), index #2=27 ("index"), index #3=28 ("index"), index #4=29 ("index"), index #5=30 ("index"), index #6=31 ("index"), index #7=6 ("index"), index #8=4 ("index"), index #9=3 ("index"), index #10=8 ("index"), index #11=14 ("index"), index #12=16 ("index"), index #13=19 ("index"), index #14=12 ("index"), index #15=13 ("index"), index #16=10 ("index"), index #17=11 ("index"), index #18=15 ("index")) -> (element #1=w474:string, element #2=w550:string, element #3=w597:string, element #4=w591:string, element #5=w589:string, element #6=w590:string, element #7=w579:string, element #8=w567:string, element #9=w562:string, element #10=w551:string, element #11=w538:string, element #12=w535:string, element #13=w534:string, element #14=w496:string, element #15=w495:string, element #16=w428:string, element #17=w409:string, element #18=w403:string)
    n174 = Scan Value(string=w368, format string="%f") -> (value=→"Calibration gas cylinder \nconcentration (ppb)":dbl)  [unwired: 1 in, 1 out]
    n175 = Scan Value(string=w440, format string="%f") -> (value=→"TEI43i MFC2 Cal Flow":dbl)  [unwired: 1 in, 1 out]
    n176 = Scan Value(string=w439, format string="%f") -> (value=→"TEI43i MFC3 Sample Flow":dbl)  [unwired: 1 in, 1 out]
    n177 = Scan Value(string=w386, format string="%f") -> (value=w372:dbl)  [unwired: 1 in, 1 out]
    n178 = Scan Value(string=w382, format string="%d", default (0 dbl)=0) -> (value=w380:i32)  [unwired: 1 out]
    n179 = Scan Value(string=w366, format string="%f") -> (value=→"SO2 react pressure":dbl)  [unwired: 1 in, 1 out]
    n180 = Scan Value(string=w376, format string="%f") -> (value=→"SO2 Sensitivity":dbl)  [unwired: 1 in, 1 out]
    n181 = Scan Value(string=w378, format string="%f") -> (value=→"SO2 Zero":dbl)  [unwired: 1 in, 1 out]
    n182 = Scan Value(string=w529, format string="%f") -> (value=w373:dbl)  [unwired: 1 in, 1 out]
    n183 = Scan Value(string=w528, format string="%f") -> (value=→"TEI43C Sample Flow":dbl)  [unwired: 1 in, 1 out]
    n184 = Not Equal To 0?(x=w380) -> (x != 0?=→"mean zero\ncal status":bool)
    n185 = Decimal String To Number(string=w474) -> (number=w472:i32)  [unwired: 2 in, 1 out]
    n186 = call "Find_Data_SubVI.vi"("FGGA"=w580, "CO"=w579, "Ozone"=w578, "SO2"=w501) -> ("Output Value"=→"CPU Total %":dbl)  [unwired: 11 in]
    n187 = call "Find_Data_SubVI.vi"("FGGA"=w568, "CO"=w567, "Ozone"=w566, "SO2"=w565) -> ("Output Value"=→"MFM":dbl)  [unwired: 11 in]
    n188 = call "Find_Data_SubVI.vi"("FGGA"=w563, "CO"=w562, "Ozone"=w561, "SO2"=w560) -> ("Output Value"=w559:dbl)  [unwired: 11 in]
    n189 = call "Find_Data_SubVI.vi"("FGGA"=w548, "CO"=w551, "Ozone"=w546, "SO2"=w553) -> ("Output Value"=→"USB Disk Space Used %":dbl)  [unwired: 11 in]
    n190 = Not Equal To 0?(x=w559) -> (x != 0?=→"PTP Sync":bool)
    n191 = Add(x=w472, y=u32 2082844800) -> (x+y=w471:u32)
    n192 = Scan Value(string=w432, format string="%f") -> (value=→"MFC1 Cal Flow":dbl)  [unwired: 1 in, 1 out]
    n193 = Scan Value(string=w396, format string="%f") -> (value=w394:dbl)  [unwired: 1 in, 1 out]
    n194 = Scan Value(string=w395, format string="%f") -> (value=w392:dbl)  [unwired: 1 in, 1 out]
    n195 = Scan Value(string=w445, format string="%f") -> (value=→"Cell temperature":dbl)  [unwired: 1 in, 1 out]
    n196 = Scan Value(string=w446, format string="%f") -> (value=→"Cell pressure":dbl)  [unwired: 1 in, 1 out]
    n197 = Scan Value(string=w451, format string="%f") -> (value=→"CH4 Dry":dbl)  [unwired: 1 in, 1 out]
    n198 = Scan Value(string=w454, format string="%f") -> (value=→"CO2 Dry":dbl)  [unwired: 1 in, 1 out]
    n199 = Scan Value(string=w456, format string="%f") -> (value=→"H2O":dbl)  [unwired: 1 in, 1 out]
    n200 = Scan Value(string=w461, format string="%f") -> (value=→"CO2":dbl)  [unwired: 1 in, 1 out]
    n201 = Scan Value(string=w464, format string="%f") -> (value=→"CH4":dbl)  [unwired: 1 in, 1 out]
    n202 = local read "PRTAFT_UDP_In"() -> (w415:string)
    n203 = Scan Value(string=w590, format string="%f") -> (value=→"Std\nContent (barG)":dbl)  [unwired: 1 in, 1 out]
    n204 = Scan Value(string=w550, format string="%d", default (0 dbl)=u32 0) -> (value=w604:u32)  [unwired: 1 out]
    n205 = Scan Value(string=w589, format string="%f") -> (value=→"N2\nContent (barG)":dbl)  [unwired: 1 in, 1 out]
    n206 = Scan Value(string=w591, format string="%f") -> (value=→"CO2\nContent (barG)":dbl)  [unwired: 1 in, 1 out]
    n207 = Scan Value(string=w597, format string="%f") -> (value=→"CO2 Pressure\nDelivery (PSIA)":dbl)  [unwired: 1 in, 1 out]
    n208 = Bundle(w373, w372) -> (→"TEi43i Concentration scaled / raw":cluster{dbl, dbl})  [unwired: 1 in]
    n209 = To Time Stamp(1:w471) -> (0:w477:timestamp)
    n210 = Scan Value(string=w538, format string="%f") -> (value=→"Lamp Flow Controller":dbl)  [unwired: 1 in, 1 out]
    n211 = Scan Value(string=w409, format string="%f") -> (value=→"Raw Signal":dbl)  [unwired: 1 in, 1 out]
    n212 = Scan Value(string=w403, format string="%f") -> (value=→"Lamp Temperature":dbl)  [unwired: 1 in, 1 out]
    n213 = Scan Value(string=w428, format string="%f") -> (value=→"CO Concentration":dbl)  [unwired: 1 in, 1 out]
    n214 = Scan Value(string=w535, format string="%f") -> (value=→"Monochromator Flow":dbl)  [unwired: 1 in, 1 out]
    n215 = Scan Value(string=w534, format string="%f") -> (value=→"Fluorescence Cell Pressure":dbl)  [unwired: 1 in, 1 out]
    n216 = Not Equal To 0?(x=w604) -> (x != 0?=→"CO CAL Status":bool)
    n217 = call "ping.vi"("host"="192.168.101.17" ("Host IP Address")) -> ("found?"=w401:bool)  [unwired: 8 in, 2 out]
    n218 = Scan Value(string=w518, format string="%f") -> (value=→"TEI49C Sample Flow B":dbl)  [unwired: 1 in, 1 out]
    n219 = Scan Value(string=w520, format string="%f") -> (value=→"TEi49C Concentration":dbl)  [unwired: 1 in, 1 out]
    n220 = Scan Value(string=w519, format string="%f") -> (value=→"TEI49C Sample Flow A":dbl)  [unwired: 1 in, 1 out]
    n221 = Scan Value(string=w496, format string="%f") -> (value=w487:dbl)  [unwired: 1 in, 1 out]
    n222 = Scan Value(string=w495, format string="%f") -> (value=w480:dbl)  [unwired: 1 in, 1 out]
    n223 = Not Equal?(x=w486, y=w487) -> (x != y?=w492:bool)
    n224 = Not Equal?(x=w478, y=w480) -> (x != y?=w485:bool)
    n225 = Spreadsheet String To Array(delimiter (Tab)=",", format string=w417, spreadsheet string=w415, array type (2D Dbl)=string[] []) -> (array=w416:string[])
    n226 = case shown="True" w492 {
      tunnel: w493 -> [w665 w674]
      tunnel: w491 -> [w666 w673]
      tunnel: [w666 w672] -> w490
      tunnel: w477 -> [_ w668]
      tunnel: w487 -> [_ w669]
      tunnel: [w665 w671] -> w489
      tunnel: [w664 w670] -> w488
      tunnel: w487 -> [_ w670]
      tunnel: w486 -> [w664 _]
      frame False {
      }
      frame True {
        n227 = Bundle(w668, w669) -> (w667:cluster{timestamp, dbl})  [unwired: 1 in]
        n228 = Replace Array Subset(array=w674, new element=w667, index=w673) -> (w671:cluster{"time stamp":timestamp, "Y":dbl}[])
        n229 = Increment(x=w673) -> (x+1=w672:i32)
      }
    }
    "CO Sensitivity" <- w489
    n230 = case shown="True" w485 {
      tunnel: w484 -> [w654 w663]
      tunnel: w483 -> [w655 w662]
      tunnel: [w655 w661] -> w481
      tunnel: w477 -> [_ w660]
      tunnel: w480 -> [_ w659]
      tunnel: [w654 w658] -> w482
      tunnel: [w653 w657] -> w479
      tunnel: w480 -> [_ w657]
      tunnel: w478 -> [w653 _]
      frame False {
      }
      frame True {
        n231 = Bundle(w660, w659) -> (w656:cluster{timestamp, dbl})  [unwired: 1 in]
        n232 = Replace Array Subset(array=w663, new element=w656, index=w662) -> (w658:cluster{"time stamp":timestamp, "Y":dbl}[])
        n233 = Increment(x=w662) -> (x+1=w661:i32)
      }
    }
    "CO Zero" <- w482
    n234 = case shown="True" w401 {
      tunnel: w476 -> [_ w652]
      tunnel: [FALSE w649] -> w475
      frame False {
      }
      frame True {
        n235 = Select(t=FALSE, s=w652, f=TRUE) -> (s? t:f=w649:bool)
      }
    }
    "Network to cRIO live status" <- w475
    n236 = Array To Spreadsheet String(delimiter (Tab)="\r", array=w416, 3:w417) -> (spreadsheet string=→"PRTAFT_DLU":string)
    n237 = Index Array(array=w416, index #1=5 ("index"), index #2=19 ("index")) -> (element #1=w420:string, element #2=w418:string)
    n238 = Not Equal?(x=w420, y=w422) -> (x != y?=w421:bool)
    n239 = Not Equal?(x=w418, y=w422) -> (x != y?=w419:bool)
    n240 = Bundle(w394, w392) -> (→"Ring Down Time RDA & RDB":cluster{dbl, dbl})  [unwired: 1 in]
    n241 = case shown="False" w419 {
      tunnel: ["1" w645] -> w412
      tunnel: w418 -> [_ w645]
      frame False {
      }
      frame True {
      }
    }
    n242 = case shown="False" w421 {
      tunnel: ["XXXX" w647] -> w413
      tunnel: w420 -> [_ w647]
      frame False {
      }
      frame True {
      }
    }
    n243 = Wait (ms)(milliseconds to wait=u32 1000) -> ()  [unwired: 1 out]
    n244 = local write "WoW Flag"(w412) -> ()
    n245 = local write "Flight Number"(w413) -> ()
  }
  n246 = while {
    stop <- FALSE stop-if-true
    # "Preflight Sub VI Descriptions"
    n247 = Wait (ms)(milliseconds to wait=u32 500) -> ()  [unwired: 1 out]
    n248 = case shown="True" "Line Lock Setting Change" {
      frame False {
      }
      frame True {
        n249 = call "FGGA Linelock Settings Procedures.vi"() -> ()  [unwired: 12 in]
      }
    }
  }
  n250 = while {
    stop <- FALSE stop-if-true
    # "Postflight Sub VI Descriptions"
    n251 = case shown="True" "Postflight Procedures" {
      frame False {
      }
      frame True {
        n252 = call "PostFlight Procedures.vi"() -> ()  [unwired: 12 in]
      }
    }
    n253 = Wait (ms)(milliseconds to wait=u32 500) -> ()  [unwired: 1 out]
  }
  n254 = while {
    stop <- FALSE stop-if-true
    # "Preflight Sub VI Descriptions"
    n255 = case shown="True" "Prepare Gases" {
      frame False {
      }
      frame True {
        n256 = call "CO Gas Preparation.vi"() -> ()  [unwired: 12 in]
      }
    }
    n257 = Wait (ms)(milliseconds to wait=u32 500) -> ()  [unwired: 1 out]
  }
  n258 = while {
    stop <- FALSE stop-if-true
    # "Preflight Sub VI Descriptions"
    n259 = case shown="True" "Prepare SO2 Span Gas" {
      frame False {
      }
      frame True {
        n260 = call "SO2 Span Gas Preparation.vi"() -> ()  [unwired: 12 in]
      }
    }
    n261 = Wait (ms)(milliseconds to wait=u32 500) -> ()  [unwired: 1 out]
  }
  n262 = while {
    stop <- FALSE stop-if-true
    # "Preflight Sub VI Descriptions"
    n263 = case shown="True" "Prepare SO2 Zero Gas" {
      frame False {
      }
      frame True {
        n264 = call "SO2 ZeroAir Gas Preparation.vi"() -> ()  [unwired: 12 in]
      }
    }
    n265 = Wait (ms)(milliseconds to wait=u32 500) -> ()  [unwired: 1 out]
  }
  n266 = Obtain Queue(name (unnamed)="FGGA_Command", element data type=w55) -> (queue out=w4:refnum<queue>, error out=w3:errorcluster)  [unwired: 3 in, 1 out]
  n267 = while {
    shift-right: [w693] -> _
    shift-left: u8 1 -> [w694]
    tunnel: w4 -> [w691]
    tunnel: w3 -> [w690]
    stop <- FALSE stop-if-true
    # "FGGA pump synchronise to WoW Wait on Wheel Flag"
    n268 = Wait (ms)(milliseconds to wait=u32 1000) -> ()  [unwired: 1 out]
    n269 = case shown="True" "FGGA pump\nsync to WoW" {
      tunnel: [w697 w702] -> w693
      tunnel: w694 -> [w697 w701]
      tunnel: w691 -> [_ w700]
      tunnel: w690 -> [_ w699]
      frame False {
      }
      frame True {
        n270 = local read "WoW Flag"() -> (w698:string)
        n271 = Scan Value(string=w698, format string="%d", default (0 dbl)=u8 0) -> (value=w702:u8)  [unwired: 1 out]
        n272 = Not Equal?(x=w702, y=w701) -> (x != y?=w705:bool)
        n273 = case shown="True" w705 {
          tunnel: w702 -> [_ w708]
          tunnel: w700 -> [_ w707]
          tunnel: w699 -> [_ w706]
          frame False {
          }
          frame True {
            n274 = Equal?(x=w708, y=u8 0) -> (x = y?=w713:bool)
            n275 = case shown="True" w713 {
              selector: w713 -> [w715 w716]
              tunnel: [w715 w716] -> w709
              frame False {
              }
              frame True {
              }
            }
            n276 = local write "Manual FGGA Pump"(w709) -> ()
            n277 = Bundle(cluster=T4 {"Message"="", "Message Data"=variant} ("Message Cluster"), "Message"="FGGA_pump", "Message Data"=w709) -> (w710:T4)
            n278 = Enqueue Element(queue=w707, element=w710, error in (no error)=w706) -> ()  [unwired: 1 in, 3 out]
          }
        }
      }
    }
  }
  n279 = while {
    tunnel: w4 -> [w718]
    tunnel: w3 -> [w717]
    tunnel: [w720] -> _
    tunnel: w15 -> [w719]
    stop <- FALSE stop-if-true
    # "FGGA UI Event Handler Loop"
    n280 = event shown="[9] \"Span Cal -  High Cal, CO Cal, Low Cal\": Value Change" {
      selector: _ -> [_ _ _ _ _ _ _ _ _ _ _ _ _ _ _ _ _]
      dyn-events: _ -> [_ _ _ _ _ _ _ _ _ _ _ _ _ _ _ _ _]
      timeout: _ -> [_ _ _ _ _ _ _ _ _ _ _ _ _ _ _ _ _]
      tunnel: w718 -> [w728 w732 w739 w746 w753 w761 w775 w782 w801 w910 w1083 w1150 w1217 w1274 w1361 w1429 w1436]
      tunnel: w717 -> [w727 w731 w738 w745 w752 w760 w774 w781 w800 w909 w1082 w1149 w1216 w1273 w1360 w1428 w1435]
      tunnel: [w722 w730 w737 w744 w751 w759 w773 w780 w787 w873 w1075 w1142 w1209 w1260 w1347 w1427 w1434] -> w720
      tunnel: w719 -> [_ _ _ _ _ _ _ _ _ w897 _ _ _ _ _ _ _]
      event "eV1": Value Change {
        n281 = event-data() -> ("NewVal"=w725:bool)  [unwired: 1 in]
        n282 = Bundle(cluster=T4 {"Message"="", "Message Data"=variant} ("Message Cluster"), "Message"="V1", "Message Data"=w725) -> (w723:T4)
        n283 = Enqueue Element(queue=w728, element=w723, error in (no error)=w727) -> (error out=w722:errorcluster)  [unwired: 1 in, 2 out]
      }
      event "eV2": Value Change {
        n284 = event-data() -> ("NewVal"=w729:bool)  [unwired: 1 in]
        n285 = Bundle(cluster=T4 {"Message"="", "Message Data"=variant} ("Message Cluster"), "Message"="V2", "Message Data"=w729) -> (w733:T4)
        n286 = Enqueue Element(queue=w732, element=w733, error in (no error)=w731) -> (error out=w730:errorcluster)  [unwired: 1 in, 2 out]
      }
      event "eV3": Value Change {
        n287 = event-data() -> ("NewVal"=w736:bool)  [unwired: 1 in]
        n288 = Bundle(cluster=T4 {"Message"="", "Message Data"=variant} ("Message Cluster"), "Message"="V3", "Message Data"=w736) -> (w740:T4)
        n289 = Enqueue Element(queue=w739, element=w740, error in (no error)=w738) -> (error out=w737:errorcluster)  [unwired: 1 in, 2 out]
      }
      event "eV4": Value Change {
        n290 = event-data() -> ("NewVal"=w743:bool)  [unwired: 1 in]
        n291 = Bundle(cluster=T4 {"Message"="", "Message Data"=variant} ("Message Cluster"), "Message"="V4", "Message Data"=w743) -> (w747:T4)
        n292 = Enqueue Element(queue=w746, element=w747, error in (no error)=w745) -> (error out=w744:errorcluster)  [unwired: 1 in, 2 out]
      }
      event "Manual FGGA Pump": Value Change {
        n293 = event-data() -> ("NewVal"=w750:bool)  [unwired: 1 in]
        n294 = Bundle(cluster=T4 {"Message"="", "Message Data"=variant} ("Message Cluster"), "Message"="FGGA_pump", "Message Data"=w750) -> (w754:T4)
        n295 = Enqueue Element(queue=w753, element=w754, error in (no error)=w752) -> (error out=w751:errorcluster)  [unwired: 1 in, 2 out]
      }
      event "Confirm Flight Number": Value Change {
        n296 = event-data() -> ()  [unwired: 1 in, 6 out]
        n297 = flat-sequence {
          tunnel: w760 -> [w763]
          tunnel: w761 -> [w764]
          tunnel: [w764] -> w758
          tunnel: [w763] -> w757
          tunnel: [w766] -> w759
          tunnel: w758 -> [w768]
          tunnel: w757 -> [w767]
          frame #0 {
            n298 = local write "cRIO File IO Stop\n(USB Flash Drive Unmount)"(FALSE ("cRIO File IO Stop\n(USB Flash Drive Unmount)")) -> ()
          }
          frame #1 {
            n299 = local read "Flight Number"() -> (w765:string)
            n300 = Bundle(cluster=T4 {"Message"="", "Message Data"=variant} ("Message Cluster"), "Message"="Flight Number", "Message Data"=w765) -> (w769:T4)
            n301 = Enqueue Element(queue=w768, element=w769, error in (no error)=w767) -> (error out=w766:errorcluster)  [unwired: 1 in, 2 out]
          }
        }
      }
      event "FGGA Restart": Value Change {
        n302 = event-data() -> ("NewVal"=w772:bool)  [unwired: 1 in]
        n303 = Bundle(cluster=T4 {"Message"="", "Message Data"=variant} ("Message Cluster"), "Message"="FGGA_restart", "Message Data"=w772) -> (w776:T4)
        n304 = Enqueue Element(queue=w775, element=w776, error in (no error)=w774) -> (error out=w773:errorcluster)  [unwired: 1 in, 2 out]
      }
      event "cRIO File IO Stop\n(USB Flash Drive Unmount)": Value Change {
        n305 = event-data() -> ("NewVal"=w779:bool)  [unwired: 1 in]
        n306 = Bundle(cluster=T4 {"Message"="", "Message Data"=variant} ("Message Cluster"), "Message"="Stop File Write", "Message Data"=w779) -> (w783:T4)
        n307 = Enqueue Element(queue=w782, element=w783, error in (no error)=w781) -> (error out=w780:errorcluster)  [unwired: 1 in, 2 out]
      }
      event "High Cal": Value Change {
        n308 = event-data() -> ()  [unwired: 1 in, 1 out]
        n309 = flat-sequence {
          tunnel: w801 -> [w806]
          tunnel: w800 -> [w805]
          tunnel: [w804] -> w799
          tunnel: [w803] -> w798
          tunnel: w799 -> [w822]
          tunnel: w798 -> [w821]
          tunnel: [w819] -> w796
          tunnel: [w818] -> w794
          tunnel: [w827] -> w797
          tunnel: w796 -> [w827]
          tunnel: [w826] -> w795
          tunnel: w794 -> [w826]
          tunnel: w797 -> [w837]
          tunnel: w795 -> [w836]
          tunnel: [w834] -> w792
          tunnel: [w833] -> w790
          tunnel: [w843] -> w793
          tunnel: w792 -> [w843]
          tunnel: [w842] -> w791
          tunnel: w790 -> [w842]
          tunnel: w793 -> [w853]
          tunnel: w791 -> [w852]
          tunnel: [w850] -> w789
          tunnel: [w849] -> w788
          tunnel: w789 -> [w867]
          tunnel: w788 -> [w866]
          tunnel: [w864] -> w786
          tunnel: [w872] -> w787
          tunnel: w786 -> [w872]
          frame #0 {
            w802 = TRUE
            n310 = Cluster To Array(cluster=T11 {"Message"="V2", "Message 2"="V3", "Message 3"="V4"}) -> (array=w807:string[])
            n311 = for {
              tunnel: w807 -> [w814] mode=indexing
              tunnel: w806 -> [w813]
              tunnel: w805 -> [w812]
              tunnel: [w811] -> w804
              tunnel: [w810] -> w803
              tunnel: w802 -> [w809]
              n312 = Bundle(cluster=T4 {"Message"="", "Message Data"=variant} ("Message Cluster"), "Message"=w814, "Message Data"=w809) -> (w816:T4)
              n313 = Enqueue Element(queue=w813, element=w816, error in (no error)=w812) -> (queue out=w811:refnum<queue>, error out=w810:errorcluster)  [unwired: 1 in, 1 out]
            }
            n314 = local write "eV2"(w802) -> ()
            n315 = local write "eV4"(w802) -> ()
            n316 = local write "eV3"(w802) -> ()
          }
          frame #1 {
            n317 = local read "MFC_1 User Set Value"() -> (w817:dbl)
            n318 = local write "MFC_1\nSLPM Value"(w817) -> ()
            n319 = Bundle(cluster=T4 {"Message"="", "Message Data"=variant} ("Message Cluster"), "Message"="MFC_1", "Message Data"=w817) -> (w820:T4)
            n320 = Enqueue Element(queue=w822, element=w820, error in (no error)=w821) -> (queue out=w819:refnum<queue>, error out=w818:errorcluster)  [unwired: 1 in, 1 out]
          }
          frame #2 {
            n321 = for {
              N: 45 -> [w831]
              i -> [w830]
              n322 = Subtract(x=w831, y=w830) -> (x-y=w829:i32)
              n323 = Decrement(x=w829) -> (x-1=→"High Cal\nFlush Time Remain (sec)":i32)
              n324 = Wait (ms)(milliseconds to wait=u32 1000) -> ()  [unwired: 1 out]
            }
          }
          frame #3 {
            w835 = TRUE
            n325 = Bundle(cluster=T4 {"Message"="", "Message Data"=variant} ("Message Cluster"), "Message"="V1", "Message Data"=w835) -> (w838:T4)
            n326 = local write "eV1"(w835) -> ()
            n327 = Enqueue Element(queue=w837, element=w838, error in (no error)=w836) -> (queue out=w834:refnum<queue>, error out=w833:errorcluster)  [unwired: 1 in, 1 out]
          }
          frame #4 {
            n328 = for {
              N: 60 -> [w847]
              i -> [w846]
              n329 = Subtract(x=w847, y=w846) -> (x-y=w845:i32)
              n330 = Decrement(x=w845) -> (x-1=→"High Cal\nCal Time Remain (sec)":i32)
              n331 = Wait (ms)(milliseconds to wait=u32 1000) -> ()  [unwired: 1 out]
            }
          }
          frame #5 {
            w851 = FALSE
            n332 = Cluster To Array(cluster=T12 {"Message"="V2", "Message 2"="V3", "Message 3"="V4", "Message 4"="V1"}) -> (array=w854:string[])
            n333 = for {
              tunnel: w854 -> [w861] mode=indexing
              tunnel: [w860] -> w850
              tunnel: [w859] -> w849
              tunnel: w851 -> [w858]
              tunnel: w853 -> [w857]
              tunnel: w852 -> [w856]
              n334 = Bundle(cluster=T4 {"Message"="", "Message Data"=variant} ("Message Cluster"), "Message"=w861, "Message Data"=w858) -> (w863:T4)
              n335 = Enqueue Element(queue=w857, element=w863, error in (no error)=w856) -> (queue out=w860:refnum<queue>, error out=w859:errorcluster)  [unwired: 1 in, 1 out]
            }
            n336 = local write "eV2"(w851) -> ()
            n337 = local write "eV4"(w851) -> ()
            n338 = local write "eV3"(w851) -> ()
            n339 = local write "eV1"(w851) -> ()
          }
          frame #6 {
            w865 = 0.0 ("MFC_1\nSLPM Value")
            n340 = local write "MFC_1\nSLPM Value"(w865) -> ()
            n341 = Bundle(cluster=T4 {"Message"="", "Message Data"=variant} ("Message Cluster"), "Message"="MFC_1", "Message Data"=w865) -> (w869:T4)
            n342 = Enqueue Element(queue=w867, element=w869, error in (no error)=w866) -> (error out=w864:errorcluster)  [unwired: 1 in, 2 out]
          }
          frame #7 {
            n343 = local write "High Cal"(FALSE ("High Cal")) -> ()
          }
        }
      }
      event "Span Cal - \nHigh Cal, CO Cal, Low Cal": Value Change {
        n344 = event-data() -> ()  [unwired: 1 in, 1 out]
        n345 = flat-sequence {
          tunnel: w910 -> [w916]
          tunnel: w909 -> [w915]
          tunnel: [w914] -> w908
          tunnel: [w913] -> w907
          tunnel: w908 -> [w932]
          tunnel: w907 -> [w931]
          tunnel: [w929] -> w905
          tunnel: [w928] -> w903
          tunnel: [w937] -> w906
          tunnel: w905 -> [w937]
          tunnel: [w936] -> w904
          tunnel: w903 -> [w936]
          tunnel: w906 -> [w943]
          tunnel: w904 -> [w944]
          tunnel: [w944] -> w879
          tunnel: w897 -> [w945]
          tunnel: [w945] -> w877
          tunnel: [w943] -> w875
          tunnel: w879 -> [w953]
          tunnel: [w953] -> w878
          tunnel: w877 -> [w952]
          tunnel: [w952] -> w876
          tunnel: w875 -> [w950]
          tunnel: [w950] -> w874
          tunnel: [w954] -> w896
          tunnel: w878 -> [w957]
          tunnel: [w956] -> w895
          tunnel: w876 -> [w966]
          tunnel: w874 -> [w955]
          tunnel: [w969] -> w902
          tunnel: w896 -> [w969]
          tunnel: [w968] -> w901
          tunnel: w895 -> [w968]
          tunnel: w902 -> [w979]
          tunnel: w901 -> [w978]
          tunnel: [w976] -> w900
          tunnel: [w975] -> w899
          tunnel: w900 -> [w994]
          tunnel: w899 -> [w993]
          tunnel: [w991] -> w898
          tunnel: [w990] -> w892
          tunnel: w898 -> [w1000]
          tunnel: [w1000] -> w894
          tunnel: [w998] -> w893
          tunnel: w892 -> [w998]
          tunnel: w894 -> [w1005]
          tunnel: w893 -> [w1007]
          tunnel: [w1004] -> w891
          tunnel: [w1001] -> w890
          tunnel: w891 -> [w1021]
          tunnel: w890 -> [w1019]
          tunnel: [w1018] -> w889
          tunnel: [w1017] -> w886
          tunnel: w889 -> [w1026]
          tunnel: [w1026] -> w888
          tunnel: [w1025] -> w887
          tunnel: w886 -> [w1025]
          tunnel: w888 -> [w1038]
          tunnel: w887 -> [w1036]
          tunnel: [w1034] -> w884
          tunnel: [w1033] -> w882
          tunnel: [w1042] -> w885
          tunnel: w884 -> [w1042]
          tunnel: [w1041] -> w883
          tunnel: w882 -> [w1041]
          tunnel: w885 -> [w1053]
          tunnel: w883 -> [w1052]
          tunnel: [w1050] -> w881
          tunnel: [w1049] -> w880
          tunnel: w881 -> [w1068]
          tunnel: w880 -> [w1067]
          tunnel: [w1064] -> w873
          frame #0 {
            w912 = TRUE
            n346 = Cluster To Array(cluster=T11 {"Message"="V2", "Message 2"="V3", "Message 3"="V4"}) -> (array=w917:string[])
            n347 = for {
              tunnel: w917 -> [w924] mode=indexing
              tunnel: w916 -> [w923]
              tunnel: w915 -> [w922]
              tunnel: [w921] -> w914
              tunnel: [w920] -> w913
              tunnel: w912 -> [w919]
              n348 = Bundle(cluster=T4 {"Message"="", "Message Data"=variant} ("Message Cluster"), "Message"=w924, "Message Data"=w919) -> (w926:T4)
              n349 = Enqueue Element(queue=w923, element=w926, error in (no error)=w922) -> (queue out=w921:refnum<queue>, error out=w920:errorcluster)  [unwired: 1 in, 1 out]
            }
            n350 = local write "High Cal"(TRUE ("High Cal")) -> ()
            n351 = local write "eV2"(w912) -> ()
            n352 = local write "eV4"(w912) -> ()
            n353 = local write "eV3"(w912) -> ()
          }
          frame #1 {
            n354 = local read "MFC_1 User Set Value"() -> (w927:dbl)
            n355 = local write "MFC_1\nSLPM Value"(w927) -> ()
            n356 = Bundle(cluster=T4 {"Message"="", "Message Data"=variant} ("Message Cluster"), "Message"="MFC_1", "Message Data"=w927) -> (w930:T4)
            n357 = Enqueue Element(queue=w932, element=w930, error in (no error)=w931) -> (queue out=w929:refnum<queue>, error out=w928:errorcluster)  [unwired: 1 in, 1 out]
          }
          frame #2 {
            n358 = for {
              N: 45 -> [w941]
              i -> [w940]
              n359 = Subtract(x=w941, y=w940) -> (x-y=w939:i32)
              n360 = Decrement(x=w939) -> (x-1=w938:i32)
              n361 = local write "High Cal\nFlush Time Remain (sec)"(w938) -> ()
              n362 = Wait (ms)(milliseconds to wait=u32 1000) -> ()  [unwired: 1 out]
            }
          }
          frame #3 {
            n363 = Bundle(cluster=T4 {"Message"="", "Message Data"=variant} ("Message Cluster"), "Message"="CO CAL", "Message Data"=TRUE) -> (w947:T4)
            n364 = Enqueue Element(queue=w945, element=w947) -> ()  [unwired: 2 in, 3 out]
          }
          frame #4 {
            # "To Ensure\nCO CAL\nis certain"
            n365 = Wait (ms)(milliseconds to wait=u32 1000) -> ()  [unwired: 1 out]
          }
          frame #5 {
            w961 = TRUE
            n366 = Bundle(cluster=T4 {"Message"="", "Message Data"=variant} ("Message Cluster"), "Message"="CO CAL", "Message Data"=FALSE) -> (w962:T4)
            n367 = Bundle(cluster=T4 {"Message"="", "Message Data"=variant} ("Message Cluster"), "Message"="V1", "Message Data"=w961) -> (w960:T4)
            n368 = local write "eV1"(w961) -> ()
            n369 = Enqueue Element(queue=w966, element=w962) -> ()  [unwired: 2 in, 3 out]
            n370 = Enqueue Element(queue=w955, element=w960, error in (no error)=w957) -> (queue out=w954:refnum<queue>, error out=w956:errorcluster)  [unwired: 1 in, 1 out]
          }
          frame #6 {
            n371 = for {
              N: 60 -> [w973]
              i -> [w972]
              n372 = Subtract(x=w973, y=w972) -> (x-y=w971:i32)
              n373 = Decrement(x=w971) -> (x-1=w970:i32)
              n374 = local write "High Cal\nCal Time Remain (sec)"(w970) -> ()
              n375 = Wait (ms)(milliseconds to wait=u32 1000) -> ()  [unwired: 1 out]
            }
          }
          frame #7 {
            w977 = FALSE
            n376 = Cluster To Array(cluster=T12 {"Message"="V2", "Message 2"="V3", "Message 3"="V4", "Message 4"="V1"}) -> (array=w980:string[])
            n377 = for {
              tunnel: w980 -> [w987] mode=indexing
              tunnel: [w986] -> w976
              tunnel: [w985] -> w975
              tunnel: w977 -> [w984]
              tunnel: w979 -> [w983]
              tunnel: w978 -> [w982]
              n378 = Bundle(cluster=T4 {"Message"="", "Message Data"=variant} ("Message Cluster"), "Message"=w987, "Message Data"=w984) -> (w989:T4)
              n379 = Enqueue Element(queue=w983, element=w989, error in (no error)=w982) -> (queue out=w986:refnum<queue>, error out=w985:errorcluster)  [unwired: 1 in, 1 out]
            }
            n380 = local write "eV2"(w977) -> ()
            n381 = local write "eV4"(w977) -> ()
            n382 = local write "eV3"(w977) -> ()
            n383 = local write "eV1"(w977) -> ()
          }
          frame #8 {
            w992 = 0.0 ("MFC_1\nSLPM Value")
            n384 = local write "MFC_1\nSLPM Value"(w992) -> ()
            n385 = Bundle(cluster=T4 {"Message"="", "Message Data"=variant} ("Message Cluster"), "Message"="MFC_1", "Message Data"=w992) -> (w996:T4)
            n386 = Enqueue Element(queue=w994, element=w996, error in (no error)=w993) -> (queue out=w990:refnum<queue>, error out=w991:errorcluster)  [unwired: 1 in, 1 out]
          }
          frame #9 {
            n387 = local write "High Cal"(FALSE ("High Cal")) -> ()
          }
          frame #10 {
            w1002 = TRUE
            n388 = Cluster To Array(cluster=cluster{"Message":string, "Message 3":string} {"Message"="V2", "Message 3"="V4"}) -> (array=w1008:string[])
            n389 = for {
              tunnel: w1008 -> [w1014] mode=indexing
              tunnel: w1007 -> [w1013]
              tunnel: [w1012] -> w1001
              tunnel: [w1011] -> w1004
              tunnel: w1002 -> [w1010]
              tunnel: w1005 -> [w1009]
              n390 = Bundle(cluster=T4 {"Message"="", "Message Data"=variant} ("Message Cluster"), "Message"=w1014, "Message Data"=w1010) -> (w1016:T4)
              n391 = Enqueue Element(queue=w1013, element=w1016, error in (no error)=w1009) -> (queue out=w1012:refnum<queue>, error out=w1011:errorcluster)  [unwired: 1 in, 1 out]
            }
            n392 = local write "eV4"(w1002) -> ()
            n393 = local write "eV2"(w1002) -> ()
            n394 = local write "Low Cal"(TRUE ("Low Cal")) -> ()
          }
          frame #11 {
            n395 = local read "MFC_1 User Set Value"() -> (w1022:dbl)
            n396 = local write "MFC_1\nSLPM Value"(w1022) -> ()
            n397 = Bundle(cluster=T4 {"Message"="", "Message Data"=variant} ("Message Cluster"), "Message"="MFC_1", "Message Data"=w1022) -> (w1023:T4)
            n398 = Enqueue Element(queue=w1019, element=w1023, error in (no error)=w1021) -> (queue out=w1018:refnum<queue>, error out=w1017:errorcluster)  [unwired: 1 in, 1 out]
          }
          frame #12 {
            n399 = for {
              N: 45 -> [w1031]
              i -> [w1030]
              n400 = Subtract(x=w1031, y=w1030) -> (x-y=w1029:i32)
              n401 = Decrement(x=w1029) -> (x-1=w1028:i32)
              n402 = local write "Low Cal\nFlush Time Remain (sec)"(w1028) -> ()
              n403 = Wait (ms)(milliseconds to wait=u32 1000) -> ()  [unwired: 1 out]
            }
          }
          frame #13 {
            w1035 = TRUE
            n404 = local write "eV1"(w1035) -> ()
            n405 = Bundle(cluster=T4 {"Message"="", "Message Data"=variant} ("Message Cluster"), "Message"="V1", "Message Data"=w1035) -> (w1039:T4)
            n406 = Enqueue Element(queue=w1038, element=w1039, error in (no error)=w1036) -> (queue out=w1034:refnum<queue>, error out=w1033:errorcluster)  [unwired: 1 in, 1 out]
          }
          frame #14 {
            n407 = for {
              N: 60 -> [w1047]
              i -> [w1046]
              n408 = Subtract(x=w1047, y=w1046) -> (x-y=w1045:i32)
              n409 = Decrement(x=w1045) -> (x-1=w1044:i32)
              n410 = local write "Low Cal\nCal Time Remain (sec)"(w1044) -> ()
              n411 = Wait (ms)(milliseconds to wait=u32 1000) -> ()  [unwired: 1 out]
            }
          }
          frame #15 {
            w1051 = FALSE
            n412 = Cluster To Array(cluster=T13 {"Message"="V2", "Message 3"="V4", "Message 4"="V1"}) -> (array=w1054:string[])
            n413 = local write "eV1"(w1051) -> ()
            n414 = local write "eV2"(w1051) -> ()
            n415 = local write "eV4"(w1051) -> ()
            n416 = for {
              tunnel: w1054 -> [w1061] mode=indexing
              tunnel: [w1060] -> w1050
              tunnel: [w1059] -> w1049
              tunnel: w1051 -> [w1058]
              tunnel: w1053 -> [w1057]
              tunnel: w1052 -> [w1056]
              n417 = Bundle(cluster=T4 {"Message"="", "Message Data"=variant} ("Message Cluster"), "Message"=w1061, "Message Data"=w1058) -> (w1063:T4)
              n418 = Enqueue Element(queue=w1057, element=w1063, error in (no error)=w1056) -> (queue out=w1060:refnum<queue>, error out=w1059:errorcluster)  [unwired: 1 in, 1 out]
            }
          }
          frame #16 {
            w1065 = FALSE
            w1066 = 0.0 ("MFC_1\nSLPM Value")
            n419 = local write "Span Cal - \nHigh Cal, CO Cal, Low Cal"(w1065) -> ()
            n420 = local write "MFC_1\nSLPM Value"(w1066) -> ()
            n421 = local write "Low Cal"(w1065) -> ()
            n422 = Bundle(cluster=T4 {"Message"="", "Message Data"=variant} ("Message Cluster"), "Message"="MFC_1", "Message Data"=w1066) -> (w1070:T4)
            n423 = Enqueue Element(queue=w1068, element=w1070, error in (no error)=w1067) -> (error out=w1064:errorcluster)  [unwired: 1 in, 2 out]
          }
        }
      }
      event "Flush High Tank": Value Change {
        n424 = event-data() -> ()  [unwired: 1 in, 1 out]
        n425 = flat-sequence {
          tunnel: w1083 -> [w1088]
          tunnel: w1082 -> [w1087]
          tunnel: [w1086] -> w1081
          tunnel: [w1085] -> w1080
          tunnel: w1081 -> [w1104]
          tunnel: w1080 -> [w1103]
          tunnel: [w1101] -> w1079
          tunnel: [w1100] -> w1078
          tunnel: w1079 -> [w1107]
          tunnel: w1078 -> [w1108]
          tunnel: [w1108] -> w1073
          tunnel: [w1107] -> w1072
          tunnel: [w1118] -> w1077
          tunnel: [w1117] -> w1076
          tunnel: w1073 -> [w1116]
          tunnel: w1072 -> [w1115]
          tunnel: w1077 -> [w1133]
          tunnel: w1076 -> [w1132]
          tunnel: [w1130] -> w1074
          tunnel: [w1138] -> w1075
          tunnel: w1074 -> [w1138]
          frame #0 {
            w1084 = TRUE
            n426 = Cluster To Array(cluster=T11 {"Message"="V2", "Message 2"="V3", "Message 3"="V4"}) -> (array=w1089:string[])
            n427 = for {
              tunnel: w1089 -> [w1096] mode=indexing
              tunnel: w1088 -> [w1095]
              tunnel: w1087 -> [w1094]
              tunnel: [w1093] -> w1086
              tunnel: [w1092] -> w1085
              tunnel: w1084 -> [w1091]
              n428 = Bundle(cluster=T4 {"Message"="", "Message Data"=variant} ("Message Cluster"), "Message"=w1096, "Message Data"=w1091) -> (w1098:T4)
              n429 = Enqueue Element(queue=w1095, element=w1098, error in (no error)=w1094) -> (queue out=w1093:refnum<queue>, error out=w1092:errorcluster)  [unwired: 1 in, 1 out]
            }
            n430 = local write "eV2"(w1084) -> ()
            n431 = local write "eV4"(w1084) -> ()
            n432 = local write "eV3"(w1084) -> ()
          }
          frame #1 {
            n433 = local read "MFC_1 User Set Value"() -> (w1099:dbl)
            n434 = local write "MFC_1\nSLPM Value"(w1099) -> ()
            n435 = Bundle(cluster=T4 {"Message"="", "Message Data"=variant} ("Message Cluster"), "Message"="MFC_1", "Message Data"=w1099) -> (w1102:T4)
            n436 = Enqueue Element(queue=w1104, element=w1102, error in (no error)=w1103) -> (queue out=w1101:refnum<queue>, error out=w1100:errorcluster)  [unwired: 1 in, 1 out]
          }
          frame #2 {
            n437 = for {
              N: 15 -> [w1113]
              i -> [w1112]
              n438 = Subtract(x=w1113, y=w1112) -> (x-y=w1111:i32)
              n439 = Decrement(x=w1111) -> (x-1=→"Flush High Tank\nTime Remain (sec)":i32)
              n440 = Wait (ms)(milliseconds to wait=u32 1000) -> ()  [unwired: 1 out]
            }
          }
          frame #3 {
            w1119 = FALSE
            n441 = Cluster To Array(cluster=T11 {"Message"="V2", "Message 2"="V3", "Message 3"="V4"}) -> (array=w1120:string[])
            n442 = for {
              tunnel: w1120 -> [w1127] mode=indexing
              tunnel: [w1126] -> w1118
              tunnel: [w1125] -> w1117
              tunnel: w1119 -> [w1124]
              tunnel: w1115 -> [w1123]
              tunnel: w1116 -> [w1122]
              n443 = Bundle(cluster=T4 {"Message"="", "Message Data"=variant} ("Message Cluster"), "Message"=w1127, "Message Data"=w1124) -> (w1129:T4)
              n444 = Enqueue Element(queue=w1123, element=w1129, error in (no error)=w1122) -> (queue out=w1126:refnum<queue>, error out=w1125:errorcluster)  [unwired: 1 in, 1 out]
            }
            n445 = local write "eV2"(w1119) -> ()
            n446 = local write "eV4"(w1119) -> ()
            n447 = local write "eV3"(w1119) -> ()
          }
          frame #4 {
            w1131 = 0.0 ("MFC_1\nSLPM Value")
            n448 = local write "MFC_1\nSLPM Value"(w1131) -> ()
            n449 = Bundle(cluster=T4 {"Message"="", "Message Data"=variant} ("Message Cluster"), "Message"="MFC_1", "Message Data"=w1131) -> (w1135:T4)
            n450 = Enqueue Element(queue=w1133, element=w1135, error in (no error)=w1132) -> (error out=w1130:errorcluster)  [unwired: 1 in, 2 out]
          }
          frame #5 {
            n451 = local write "Flush High Tank"(FALSE ("High Cal")) -> ()
          }
        }
      }
      event "Flush Low Tank": Value Change {
        n452 = event-data() -> ()  [unwired: 1 in, 1 out]
        n453 = flat-sequence {
          tunnel: w1150 -> [w1155]
          tunnel: w1149 -> [w1154]
          tunnel: [w1153] -> w1148
          tunnel: [w1152] -> w1147
          tunnel: w1148 -> [w1171]
          tunnel: w1147 -> [w1170]
          tunnel: [w1168] -> w1146
          tunnel: [w1167] -> w1145
          tunnel: w1146 -> [w1174]
          tunnel: w1145 -> [w1175]
          tunnel: [w1175] -> w1140
          tunnel: [w1174] -> w1139
          tunnel: [w1185] -> w1144
          tunnel: [w1184] -> w1143
          tunnel: w1140 -> [w1183]
          tunnel: w1139 -> [w1182]
          tunnel: w1144 -> [w1200]
          tunnel: w1143 -> [w1199]
          tunnel: [w1197] -> w1141
          tunnel: [w1205] -> w1142
          tunnel: w1141 -> [w1205]
          frame #0 {
            w1151 = TRUE
            n454 = Cluster To Array(cluster=cluster{"Message":string, "Message 3":string} {"Message"="V2", "Message 3"="V4"}) -> (array=w1156:string[])
            n455 = for {
              tunnel: w1156 -> [w1163] mode=indexing
              tunnel: w1155 -> [w1162]
              tunnel: w1154 -> [w1161]
              tunnel: [w1160] -> w1153
              tunnel: [w1159] -> w1152
              tunnel: w1151 -> [w1158]
              n456 = Bundle(cluster=T4 {"Message"="", "Message Data"=variant} ("Message Cluster"), "Message"=w1163, "Message Data"=w1158) -> (w1165:T4)
              n457 = Enqueue Element(queue=w1162, element=w1165, error in (no error)=w1161) -> (queue out=w1160:refnum<queue>, error out=w1159:errorcluster)  [unwired: 1 in, 1 out]
            }
            n458 = local write "eV2"(w1151) -> ()
            n459 = local write "eV4"(w1151) -> ()
          }
          frame #1 {
            n460 = local read "MFC_1 User Set Value"() -> (w1166:dbl)
            n461 = local write "MFC_1\nSLPM Value"(w1166) -> ()
            n462 = Bundle(cluster=T4 {"Message"="", "Message Data"=variant} ("Message Cluster"), "Message"="MFC_1", "Message Data"=w1166) -> (w1169:T4)
            n463 = Enqueue Element(queue=w1171, element=w1169, error in (no error)=w1170) -> (queue out=w1168:refnum<queue>, error out=w1167:errorcluster)  [unwired: 1 in, 1 out]
          }
          frame #2 {
            n464 = for {
              N: 15 -> [w1180]
              i -> [w1179]
              n465 = Subtract(x=w1180, y=w1179) -> (x-y=w1178:i32)
              n466 = Decrement(x=w1178) -> (x-1=→"Flush Low Tank\nTime Remain (sec)":i32)
              n467 = Wait (ms)(milliseconds to wait=u32 1000) -> ()  [unwired: 1 out]
            }
          }
          frame #3 {
            w1186 = FALSE
            n468 = Cluster To Array(cluster=cluster{"Message":string, "Message 3":string} {"Message"="V2", "Message 3"="V4"}) -> (array=w1187:string[])
            n469 = for {
              tunnel: w1187 -> [w1194] mode=indexing
              tunnel: [w1193] -> w1185
              tunnel: [w1192] -> w1184
              tunnel: w1186 -> [w1191]
              tunnel: w1182 -> [w1190]
              tunnel: w1183 -> [w1189]
              n470 = Bundle(cluster=T4 {"Message"="", "Message Data"=variant} ("Message Cluster"), "Message"=w1194, "Message Data"=w1191) -> (w1196:T4)
              n471 = Enqueue Element(queue=w1190, element=w1196, error in (no error)=w1189) -> (queue out=w1193:refnum<queue>, error out=w1192:errorcluster)  [unwired: 1 in, 1 out]
            }
            n472 = local write "eV2"(w1186) -> ()
            n473 = local write "eV4"(w1186) -> ()
          }
          frame #4 {
            w1198 = 0.0 ("MFC_1\nSLPM Value")
            n474 = local write "MFC_1\nSLPM Value"(w1198) -> ()
            n475 = Bundle(cluster=T4 {"Message"="", "Message Data"=variant} ("Message Cluster"), "Message"="MFC_1", "Message Data"=w1198) -> (w1202:T4)
            n476 = Enqueue Element(queue=w1200, element=w1202, error in (no error)=w1199) -> (error out=w1197:errorcluster)  [unwired: 1 in, 2 out]
          }
          frame #5 {
            n477 = local write "Flush Low Tank"(FALSE ("High Cal")) -> ()
          }
        }
      }
      event "Flush Target Tank": Value Change {
        n478 = event-data() -> ()  [unwired: 1 in, 1 out]
        n479 = flat-sequence {
          tunnel: w1217 -> [w1225]
          tunnel: w1216 -> [w1224]
          tunnel: [w1223] -> w1215
          tunnel: [w1222] -> w1214
          tunnel: w1215 -> [w1231]
          tunnel: w1214 -> [w1230]
          tunnel: [w1228] -> w1213
          tunnel: [w1227] -> w1212
          tunnel: w1213 -> [w1234]
          tunnel: w1212 -> [w1235]
          tunnel: [w1235] -> w1207
          tunnel: [w1234] -> w1206
          tunnel: [w1248] -> w1211
          tunnel: [w1247] -> w1210
          tunnel: w1207 -> [w1246]
          tunnel: w1206 -> [w1245]
          tunnel: w1211 -> [w1253]
          tunnel: w1210 -> [w1252]
          tunnel: [w1250] -> w1208
          tunnel: [w1258] -> w1209
          tunnel: w1208 -> [w1258]
          frame #0 {
            w1221 = TRUE
            n480 = local write "eV4"(w1221) -> ()
            n481 = Bundle(cluster=T4 {"Message"="", "Message Data"=variant} ("Message Cluster"), "Message"="V4" ("Message 3"), "Message Data"=w1221) -> (w1220:T4)
            n482 = Enqueue Element(queue=w1225, element=w1220, error in (no error)=w1224) -> (queue out=w1223:refnum<queue>, error out=w1222:errorcluster)  [unwired: 1 in, 1 out]
          }
          frame #1 {
            n483 = local read "MFC_1 User Set Value"() -> (w1226:dbl)
            n484 = local write "MFC_1\nSLPM Value"(w1226) -> ()
            n485 = Bundle(cluster=T4 {"Message"="", "Message Data"=variant} ("Message Cluster"), "Message"="MFC_1", "Message Data"=w1226) -> (w1229:T4)
            n486 = Enqueue Element(queue=w1231, element=w1229, error in (no error)=w1230) -> (queue out=w1228:refnum<queue>, error out=w1227:errorcluster)  [unwired: 1 in, 1 out]
          }
          frame #2 {
            n487 = for {
              N: 15 -> [w1240]
              i -> [w1239]
              n488 = Subtract(x=w1240, y=w1239) -> (x-y=w1238:i32)
              n489 = Decrement(x=w1238) -> (x-1=→"Flush Target Tank\nTime Remain (sec)":i32)
              n490 = Wait (ms)(milliseconds to wait=u32 1000) -> ()  [unwired: 1 out]
            }
          }
          frame #3 {
            w1249 = FALSE
            n491 = Bundle(cluster=T4 {"Message"="", "Message Data"=variant} ("Message Cluster"), "Message"="V4" ("Message 3"), "Message Data"=w1249) -> (w1244:T4)
            n492 = local write "eV4"(w1249) -> ()
            n493 = Enqueue Element(queue=w1245, element=w1244, error in (no error)=w1246) -> (queue out=w1248:refnum<queue>, error out=w1247:errorcluster)  [unwired: 1 in, 1 out]
          }
          frame #4 {
            w1251 = 0.0 ("MFC_1\nSLPM Value")
            n494 = local write "MFC_1\nSLPM Value"(w1251) -> ()
            n495 = Bundle(cluster=T4 {"Message"="", "Message Data"=variant} ("Message Cluster"), "Message"="MFC_1", "Message Data"=w1251) -> (w1255:T4)
            n496 = Enqueue Element(queue=w1253, element=w1255, error in (no error)=w1252) -> (error out=w1250:errorcluster)  [unwired: 1 in, 2 out]
          }
          frame #5 {
            n497 = local write "Flush Target Tank"(FALSE ("High Cal")) -> ()
          }
        }
      }
      event "Low Cal": Value Change {
        n498 = event-data() -> ()  [unwired: 1 in, 1 out]
        n499 = flat-sequence {
          tunnel: w1274 -> [w1279]
          tunnel: w1273 -> [w1278]
          tunnel: [w1277] -> w1272
          tunnel: [w1276] -> w1271
          tunnel: w1272 -> [w1295]
          tunnel: w1271 -> [w1294]
          tunnel: [w1292] -> w1269
          tunnel: [w1291] -> w1267
          tunnel: [w1300] -> w1270
          tunnel: w1269 -> [w1300]
          tunnel: [w1299] -> w1268
          tunnel: w1267 -> [w1299]
          tunnel: w1270 -> [w1310]
          tunnel: w1268 -> [w1309]
          tunnel: [w1307] -> w1265
          tunnel: [w1306] -> w1263
          tunnel: [w1316] -> w1266
          tunnel: w1265 -> [w1316]
          tunnel: [w1315] -> w1264
          tunnel: w1263 -> [w1315]
          tunnel: w1266 -> [w1326]
          tunnel: w1264 -> [w1325]
          tunnel: [w1323] -> w1262
          tunnel: [w1322] -> w1261
          tunnel: w1262 -> [w1340]
          tunnel: w1261 -> [w1339]
          tunnel: [w1337] -> w1259
          tunnel: [w1345] -> w1260
          tunnel: w1259 -> [w1345]
          frame #0 {
            w1275 = TRUE
            n500 = Cluster To Array(cluster=cluster{"Message":string, "Message 3":string} {"Message"="V2", "Message 3"="V4"}) -> (array=w1280:string[])
            n501 = for {
              tunnel: w1280 -> [w1287] mode=indexing
              tunnel: w1279 -> [w1286]
              tunnel: w1278 -> [w1285]
              tunnel: [w1284] -> w1277
              tunnel: [w1283] -> w1276
              tunnel: w1275 -> [w1282]
              n502 = Bundle(cluster=T4 {"Message"="", "Message Data"=variant} ("Message Cluster"), "Message"=w1287, "Message Data"=w1282) -> (w1289:T4)
              n503 = Enqueue Element(queue=w1286, element=w1289, error in (no error)=w1285) -> (queue out=w1284:refnum<queue>, error out=w1283:errorcluster)  [unwired: 1 in, 1 out]
            }
            n504 = local write "eV2"(w1275) -> ()
            n505 = local write "eV4"(w1275) -> ()
          }
          frame #1 {
            n506 = local read "MFC_1 User Set Value"() -> (w1290:dbl)
            n507 = local write "MFC_1\nSLPM Value"(w1290) -> ()
            n508 = Bundle(cluster=T4 {"Message"="", "Message Data"=variant} ("Message Cluster"), "Message"="MFC_1", "Message Data"=w1290) -> (w1293:T4)
            n509 = Enqueue Element(queue=w1295, element=w1293, error in (no error)=w1294) -> (queue out=w1292:refnum<queue>, error out=w1291:errorcluster)  [unwired: 1 in, 1 out]
          }
          frame #2 {
            n510 = for {
              N: 45 -> [w1304]
              i -> [w1303]
              n511 = Subtract(x=w1304, y=w1303) -> (x-y=w1302:i32)
              n512 = Decrement(x=w1302) -> (x-1=→"Low Cal\nFlush Time Remain (sec)":i32)
              n513 = Wait (ms)(milliseconds to wait=u32 1000) -> ()  [unwired: 1 out]
            }
          }
          frame #3 {
            w1308 = TRUE
            n514 = Bundle(cluster=T4 {"Message"="", "Message Data"=variant} ("Message Cluster"), "Message"="V1", "Message Data"=w1308) -> (w1311:T4)
            n515 = local write "eV1"(w1308) -> ()
            n516 = Enqueue Element(queue=w1310, element=w1311, error in (no error)=w1309) -> (queue out=w1307:refnum<queue>, error out=w1306:errorcluster)  [unwired: 1 in, 1 out]
          }
          frame #4 {
            n517 = for {
              N: 60 -> [w1320]
              i -> [w1319]
              n518 = Subtract(x=w1320, y=w1319) -> (x-y=w1318:i32)
              n519 = Decrement(x=w1318) -> (x-1=→"Low Cal\nCal Time Remain (sec)":i32)
              n520 = Wait (ms)(milliseconds to wait=u32 1000) -> ()  [unwired: 1 out]
            }
          }
          frame #5 {
            w1324 = FALSE
            n521 = Cluster To Array(cluster=T13 {"Message"="V2", "Message 3"="V4", "Message 4"="V1"}) -> (array=w1327:string[])
            n522 = for {
              tunnel: w1327 -> [w1334] mode=indexing
              tunnel: [w1333] -> w1323
              tunnel: [w1332] -> w1322
              tunnel: w1324 -> [w1331]
              tunnel: w1326 -> [w1330]
              tunnel: w1325 -> [w1329]
              n523 = Bundle(cluster=T4 {"Message"="", "Message Data"=variant} ("Message Cluster"), "Message"=w1334, "Message Data"=w1331) -> (w1336:T4)
              n524 = Enqueue Element(queue=w1330, element=w1336, error in (no error)=w1329) -> (queue out=w1333:refnum<queue>, error out=w1332:errorcluster)  [unwired: 1 in, 1 out]
            }
            n525 = local write "eV2"(w1324) -> ()
            n526 = local write "eV4"(w1324) -> ()
            n527 = local write "eV1"(w1324) -> ()
          }
          frame #6 {
            w1338 = 0.0 ("MFC_1\nSLPM Value")
            n528 = local write "MFC_1\nSLPM Value"(w1338) -> ()
            n529 = Bundle(cluster=T4 {"Message"="", "Message Data"=variant} ("Message Cluster"), "Message"="MFC_1", "Message Data"=w1338) -> (w1342:T4)
            n530 = Enqueue Element(queue=w1340, element=w1342, error in (no error)=w1339) -> (error out=w1337:errorcluster)  [unwired: 1 in, 2 out]
          }
          frame #7 {
            n531 = local write "Low Cal"(FALSE ("High Cal")) -> ()
          }
        }
      }
      event "Target Cal": Value Change {
        n532 = event-data() -> ()  [unwired: 1 in, 1 out]
        n533 = flat-sequence {
          tunnel: w1361 -> [w1369]
          tunnel: w1360 -> [w1368]
          tunnel: [w1367] -> w1359
          tunnel: [w1366] -> w1358
          tunnel: w1359 -> [w1375]
          tunnel: w1358 -> [w1374]
          tunnel: [w1372] -> w1356
          tunnel: [w1371] -> w1354
          tunnel: [w1380] -> w1357
          tunnel: w1356 -> [w1380]
          tunnel: [w1379] -> w1355
          tunnel: w1354 -> [w1379]
          tunnel: w1357 -> [w1390]
          tunnel: w1355 -> [w1389]
          tunnel: [w1387] -> w1352
          tunnel: [w1386] -> w1350
          tunnel: [w1396] -> w1353
          tunnel: w1352 -> [w1396]
          tunnel: [w1395] -> w1351
          tunnel: w1350 -> [w1395]
          tunnel: w1353 -> [w1405]
          tunnel: w1351 -> [w1404]
          tunnel: [w1402] -> w1349
          tunnel: [w1403] -> w1348
          tunnel: w1349 -> [w1420]
          tunnel: w1348 -> [w1419]
          tunnel: [w1417] -> w1346
          tunnel: [w1425] -> w1347
          tunnel: w1346 -> [w1425]
          frame #0 {
            w1365 = TRUE
            n534 = local write "eV4"(w1365) -> ()
            n535 = Bundle(cluster=T4 {"Message"="", "Message Data"=variant} ("Message Cluster"), "Message"="V4" ("Message 3"), "Message Data"=w1365) -> (w1364:T4)
            n536 = Enqueue Element(queue=w1369, element=w1364, error in (no error)=w1368) -> (queue out=w1367:refnum<queue>, error out=w1366:errorcluster)  [unwired: 1 in, 1 out]
          }
          frame #1 {
            n537 = local read "MFC_1 User Set Value"() -> (w1370:dbl)
            n538 = local write "MFC_1\nSLPM Value"(w1370) -> ()
            n539 = Bundle(cluster=T4 {"Message"="", "Message Data"=variant} ("Message Cluster"), "Message"="MFC_1", "Message Data"=w1370) -> (w1373:T4)
            n540 = Enqueue Element(queue=w1375, element=w1373, error in (no error)=w1374) -> (queue out=w1372:refnum<queue>, error out=w1371:errorcluster)  [unwired: 1 in, 1 out]
          }
          frame #2 {
            n541 = for {
              N: 45 -> [w1384]
              i -> [w1383]
              n542 = Subtract(x=w1384, y=w1383) -> (x-y=w1382:i32)
              n543 = Decrement(x=w1382) -> (x-1=→"Target Cal\nFlush Time Remain (sec)":i32)
              n544 = Wait (ms)(milliseconds to wait=u32 1000) -> ()  [unwired: 1 out]
            }
          }
          frame #3 {
            w1388 = TRUE
            n545 = Bundle(cluster=T4 {"Message"="", "Message Data"=variant} ("Message Cluster"), "Message"="V1", "Message Data"=w1388) -> (w1391:T4)
            n546 = local write "eV1"(w1388) -> ()
            n547 = Enqueue Element(queue=w1390, element=w1391, error in (no error)=w1389) -> (queue out=w1387:refnum<queue>, error out=w1386:errorcluster)  [unwired: 1 in, 1 out]
          }
          frame #4 {
            n548 = for {
              N: 60 -> [w1400]
              i -> [w1399]
              n549 = Subtract(x=w1400, y=w1399) -> (x-y=w1398:i32)
              n550 = Decrement(x=w1398) -> (x-1=→"Target Cal\nCal Time Remain (sec)":i32)
              n551 = Wait (ms)(milliseconds to wait=u32 1000) -> ()  [unwired: 1 out]
            }
          }
          frame #5 {
            w1408 = FALSE
            n552 = Cluster To Array(cluster=cluster{"Message 3":string, "Message":string} {"Message 3"="V4", "Message"="V1"}) -> (array=w1406:string[])
            n553 = for {
              tunnel: w1406 -> [w1414] mode=indexing
              tunnel: [w1413] -> w1402
              tunnel: [w1412] -> w1403
              tunnel: w1408 -> [w1411]
              tunnel: w1405 -> [w1410]
              tunnel: w1404 -> [w1409]
              n554 = Bundle(cluster=T4 {"Message"="", "Message Data"=variant} ("Message Cluster"), "Message"=w1414, "Message Data"=w1411) -> (w1416:T4)
              n555 = Enqueue Element(queue=w1410, element=w1416, error in (no error)=w1409) -> (queue out=w1413:refnum<queue>, error out=w1412:errorcluster)  [unwired: 1 in, 1 out]
            }
            n556 = local write "eV4"(w1408) -> ()
            n557 = local write "eV1"(w1408) -> ()
          }
          frame #6 {
            w1418 = 0.0 ("MFC_1\nSLPM Value")
            n558 = local write "MFC_1\nSLPM Value"(w1418) -> ()
            n559 = Bundle(cluster=T4 {"Message"="", "Message Data"=variant} ("Message Cluster"), "Message"="MFC_1", "Message Data"=w1418) -> (w1422:T4)
            n560 = Enqueue Element(queue=w1420, element=w1422, error in (no error)=w1419) -> (error out=w1417:errorcluster)  [unwired: 1 in, 2 out]
          }
          frame #7 {
            n561 = local write "Target Cal"(FALSE ("High Cal")) -> ()
          }
        }
      }
      event "MFC_1\nSLPM Value": Value Change {
        n562 = event-data() -> ()  [unwired: 1 in, 1 out]
        n563 = local read "MFC_1\nSLPM Value"() -> (w1426:dbl)
        n564 = Bundle(cluster=T4 {"Message"="", "Message Data"=variant} ("Message Cluster"), "Message"="MFC_1", "Message Data"=w1426) -> (w1430:T4)
        n565 = Enqueue Element(queue=w1429, element=w1430, error in (no error)=w1428) -> (error out=w1427:errorcluster)  [unwired: 1 in, 2 out]
      }
      event "FGGA UDP Time Offset": Value Change {
        n566 = event-data() -> ("NewVal"=w1433:i32)  [unwired: 1 in, 5 out]
        n567 = Bundle(cluster=T4 {"Message"="", "Message Data"=variant} ("Message Cluster"), "Message"="UDP Time Offset", "Message Data"=w1433) -> (w1437:T4)
        n568 = Enqueue Element(queue=w1436, element=w1437, error in (no error)=w1435) -> (error out=w1434:errorcluster)  [unwired: 1 in, 2 out]
      }
    }
    "FGGA Event Error out" <- w720
  }
  n569 = Create Network Stream Writer Endpoint(6:w53, 7:10 ("writer buffer size"), 9:w55, 10:"//192.168.101.17/command/reader/FGGA" ("reader url"), 11:"/command/writer/FGGA" ("writer name")) -> (0:w52:errorcluster, 3:w51:refnum<k21>)  [unwired: 2 in]
  n570 = node-c288(w13) -> ()  [unwired: 1 out]
  n571 = while {
    tunnel: w4 -> [w1447]
    shift-right: [w1442] -> _
    shift-left: w51 -> [w1444]
    shift-right: [w1440] -> w48
    shift-left: w52 -> [w1446]
    tunnel: w3 -> [w1441]
    stop <- w1440 stop-if-true
    # "FGGA UI Command Sender"
    n572 = Dequeue Element(queue=w1447, error in (no error)=w1441) -> (element=w1443:T4)  [unwired: 1 in, 3 out]
    n573 = Unbundle By Name(w1443) -> ("Message"=w1445:string)
    n574 = case shown="\"UDP Time Offset\"" w1445 {
      tunnel: w1446 -> [w1448 w1452 w1459 w1466 w1473 w1480 w1487 w1494 w1501 w1508 w1515]
      tunnel: w1444 -> [w1449 w1455 w1462 w1469 w1476 w1483 w1490 w1497 w1504 w1511 w1518]
      tunnel: w1443 -> [_ w1454 w1461 w1468 w1475 w1482 w1489 w1496 w1503 w1510 w1517]
      tunnel: [w1448 w1451 w1458 w1465 w1472 w1479 w1486 w1493 w1500 w1507 w1514] -> w1440
      tunnel: [w1449 w1450 w1457 w1464 w1471 w1478 w1485 w1492 w1499 w1506 w1513] -> w1442
      frame "False", Default {
      }
      frame "V1" {
        n575 = shared-variable-write(w1455, w1452, w1454) -> (w1453:refnum<k21>, w1456:errorcluster)  [unwired: 1 in, 1 out]
        n576 = Flush Stream(8:w1456, 11:w1453) -> (0:w1451:errorcluster, 3:w1450:refnum<k21>)  [unwired: 2 in, 1 out]
      }
      frame "MFC_1" {
        n577 = shared-variable-write(w1462, w1459, w1461) -> (w1460:refnum<k21>, w1463:errorcluster)  [unwired: 1 in, 1 out]
        n578 = Flush Stream(8:w1463, 11:w1460) -> (0:w1458:errorcluster, 3:w1457:refnum<k21>)  [unwired: 2 in, 1 out]
      }
      frame "UDP Time Offset" {
        n579 = shared-variable-write(w1469, w1466, w1468) -> (w1467:refnum<k21>, w1470:errorcluster)  [unwired: 1 in, 1 out]
        n580 = Flush Stream(8:w1470, 11:w1467) -> (0:w1465:errorcluster, 3:w1464:refnum<k21>)  [unwired: 2 in, 1 out]
      }
      frame "V2" {
        n581 = shared-variable-write(w1476, w1473, w1475) -> (w1474:refnum<k21>, w1477:errorcluster)  [unwired: 1 in, 1 out]
        n582 = Flush Stream(8:w1477, 11:w1474) -> (0:w1472:errorcluster, 3:w1471:refnum<k21>)  [unwired: 2 in, 1 out]
      }
      frame "V3" {
        n583 = shared-variable-write(w1483, w1480, w1482) -> (w1481:refnum<k21>, w1484:errorcluster)  [unwired: 1 in, 1 out]
        n584 = Flush Stream(8:w1484, 11:w1481) -> (0:w1479:errorcluster, 3:w1478:refnum<k21>)  [unwired: 2 in, 1 out]
      }
      frame "V4" {
        n585 = shared-variable-write(w1490, w1487, w1489) -> (w1488:refnum<k21>, w1491:errorcluster)  [unwired: 1 in, 1 out]
        n586 = Flush Stream(8:w1491, 11:w1488) -> (0:w1486:errorcluster, 3:w1485:refnum<k21>)  [unwired: 2 in, 1 out]
      }
      frame "FGGA_pump" {
        n587 = shared-variable-write(w1497, w1494, w1496) -> (w1495:refnum<k21>, w1498:errorcluster)  [unwired: 1 in, 1 out]
        n588 = Flush Stream(8:w1498, 11:w1495) -> (0:w1493:errorcluster, 3:w1492:refnum<k21>)  [unwired: 2 in, 1 out]
      }
      frame "Flight Number" {
        n589 = shared-variable-write(w1504, w1501, w1503) -> (w1502:refnum<k21>, w1505:errorcluster)  [unwired: 1 in, 1 out]
        n590 = Flush Stream(8:w1505, 11:w1502) -> (0:w1500:errorcluster, 3:w1499:refnum<k21>)  [unwired: 2 in, 1 out]
      }
      frame "FGGA_restart" {
        n591 = shared-variable-write(w1511, w1508, w1510) -> (w1509:refnum<k21>, w1512:errorcluster)  [unwired: 1 in, 1 out]
        n592 = Flush Stream(8:w1512, 11:w1509) -> (0:w1507:errorcluster, 3:w1506:refnum<k21>)  [unwired: 2 in, 1 out]
      }
      frame "Stop File Write" {
        n593 = shared-variable-write(w1518, w1515, w1517) -> (w1516:refnum<k21>, w1519:errorcluster)  [unwired: 1 in, 1 out]
        n594 = Flush Stream(8:w1519, 11:w1516) -> (0:w1514:errorcluster, 3:w1513:refnum<k21>)  [unwired: 2 in, 1 out]
      }
    }
  }
  "FGGA command sender error out" <- w48
  n595 = Obtain Queue(name (unnamed)="SO2_Command", element data type=w39) -> (queue out=w2:refnum<queue>, error out=w1:errorcluster)  [unwired: 3 in, 1 out]
  n596 = while {
    tunnel: w2 -> [w1521]
    tunnel: w1 -> [w1520]
    stop <- FALSE stop-if-true
    # "SO2 Auto Zero Handler Loop"
    n597 = local read "SO2 CAL/Zero"() -> (w1525:bool)
    n598 = Equal?(x=w1525, y=FALSE) -> (x = y?=w1523:bool)
    n599 = And(x="SO2 Auto Zeroing", y=w1523) -> (x .and. y?=w1526:bool)
    n600 = case shown="True" w1526 {
      tunnel: w1521 -> [_ w1543]
      tunnel: w1520 -> [_ w1542]
      frame False {
        n601 = local write "Auto Zero\nIndicator"("Auto Zero Inactive; Manual Zero Allow" ("Auto Zero Indicator")) -> ()
        n602 = local write "SO2 Pause\nAuto Zeroing"(FALSE ("SO2 Pause\nAuto Zeroing")) -> ()
        n603 = property on="SO2 CAL/Zero" class="Bool (strict)"("Visible"=TRUE) -> ()  [unwired: 2 in, 2 out]
      }
      frame True {
        n604 = flat-sequence {
          tunnel: w1542 -> [w1558]
          tunnel: w1543 -> [w1559]
          tunnel: [w1559] -> w1541
          tunnel: [w1558] -> w1540
          tunnel: w1541 -> [w1568]
          tunnel: w1540 -> [w1567]
          tunnel: [w1566] -> w1539
          tunnel: [w1565] -> w1538
          tunnel: [w1574] -> w1555
          tunnel: [w1573] -> w1554
          tunnel: w1539 -> [w1578]
          tunnel: w1538 -> [w1579]
          tunnel: w1555 -> [w1583]
          tunnel: [w1582] -> w1553
          tunnel: w1554 -> [w1584]
          tunnel: [w1581] -> w1552
          tunnel: w1553 -> [w1590]
          tunnel: [w1590] -> w1551
          tunnel: w1552 -> [w1589]
          tunnel: [w1589] -> w1550
          tunnel: w1551 -> [w1599]
          tunnel: w1550 -> [w1600]
          tunnel: [w1598] -> w1549
          tunnel: [w1597] -> w1548
          tunnel: [w1606] -> w1547
          tunnel: w1549 -> [w1606]
          tunnel: [w1605] -> w1546
          tunnel: w1548 -> [w1605]
          tunnel: w1547 -> [w1615]
          tunnel: w1546 -> [w1614]
          tunnel: [w1613] -> w1545
          tunnel: [w1612] -> w1544
          tunnel: w1545 -> [w1631]
          tunnel: w1544 -> [w1630]
          tunnel: [w1628] -> w1536
          tunnel: [w1627] -> w1535
          tunnel: [w1636] -> w1537
          tunnel: w1536 -> [w1636]
          tunnel: w1535 -> [w1635]
          tunnel: [w1635] -> w1534
          tunnel: [w1639] -> w1533
          tunnel: w1534 -> [w1638]
          tunnel: w1537 -> [w1639]
          tunnel: [w1638] -> w1532
          tunnel: w1533 -> [w1674]
          tunnel: w1532 -> [w1673]
          frame #0 {
            n605 = local write "Auto Zero\nIndicator"("Auto Zero In Progress" ("Auto Zero\nIndicator")) -> ()
            n606 = while {
              stop <- w1560 stop-if-true
              n607 = local read "eV9"() -> (w1562:bool)
              n608 = Equal?(x=w1562, y=FALSE) -> (x = y?=w1560:bool)
              n609 = Wait (ms)(milliseconds to wait=u32 1000) -> ()  [unwired: 1 out]
            }
            n610 = property on="SO2 CAL/Zero" class="Bool (strict)"("Visible"=FALSE) -> ()  [unwired: 2 in, 2 out]
          }
          frame #1 {
            n611 = Bundle(cluster=T4 {"Message"="", "Message Data"=variant} ("Message Cluster"), "Message"="Auto_zero", "Message Data"=TRUE) -> (w1569:T4)
            n612 = Enqueue Element(queue=w1568, element=w1569, error in (no error)=w1567) -> (queue out=w1565:refnum<queue>, error out=w1566:errorcluster)  [unwired: 1 in, 1 out]
          }
          frame #2 {
            w1572 = TRUE ("SO2 Flush")
            n613 = Bundle(cluster=T4 {"Message"="", "Message Data"=variant} ("Message Cluster"), "Message"="V9", "Message Data"=w1572) -> (w1575:T4)
            n614 = local write "eV9"(w1572) -> ()
            n615 = Enqueue Element(queue=w1579, element=w1575, error in (no error)=w1578) -> (queue out=w1573:refnum<queue>, error out=w1574:errorcluster)  [unwired: 1 in, 1 out]
          }
          frame #3 {
            n616 = local read "MFC_2 User Set Value"() -> (w1580:dbl)
            n617 = local write "MFC_2 User Set Value"(w1580) -> ()
            n618 = Bundle(cluster=T4 {"Message"="", "Message Data"=variant} ("Message Cluster"), "Message"="MFC_2", "Message Data"=w1580) -> (w1585:T4)
            n619 = Enqueue Element(queue=w1584, element=w1585, error in (no error)=w1583) -> (queue out=w1581:refnum<queue>, error out=w1582:errorcluster)  [unwired: 1 in, 1 out]
          }
          frame #4 {
            n620 = local read "eV9 flush User\nset time (sec)"() -> (w1588:i32)
            n621 = for {
              N: w1588 -> [w1594]
              i -> [w1593]
              n622 = Subtract(x=w1594, y=w1593) -> (x-y=w1592:i32)
              n623 = Decrement(x=w1592) -> (x-1=w1591:i32)
              n624 = local write "SO2 Cal/Zero Flush\nTime Remain (sec)"(w1591) -> ()
              n625 = Wait (ms)(milliseconds to wait=u32 1000) -> ()  [unwired: 1 out]
            }
          }
          frame #5 {
            w1596 = TRUE ("SO2 Flush")
            n626 = Bundle(cluster=T4 {"Message"="", "Message Data"=variant} ("Message Cluster"), "Message"="V8", "Message Data"=w1596) -> (w1601:T4)
            n627 = local write "eV8"(w1596) -> ()
            n628 = Enqueue Element(queue=w1600, element=w1601, error in (no error)=w1599) -> (queue out=w1598:refnum<queue>, error out=w1597:errorcluster)  [unwired: 1 in, 1 out]
          }
          frame #6 {
            n629 = local read "eV8 User\nset time (sec)"() -> (w1604:i32)
            n630 = for {
              N: w1604 -> [w1610]
              i -> [w1609]
              n631 = Subtract(x=w1610, y=w1609) -> (x-y=w1608:i32)
              n632 = Decrement(x=w1608) -> (x-1=w1607:i32)
              n633 = local write "SO2 CAL/Zero\nTime Remain (sec)"(w1607) -> ()
              n634 = Wait (ms)(milliseconds to wait=u32 1000) -> ()  [unwired: 1 out]
            }
          }
          frame #7 {
            n635 = Cluster To Array(cluster=cluster{"Message":string, "Message 2":string} {"Message"="V8", "Message 2"="V9"}) -> (array=w1617:string[])
            n636 = for {
              tunnel: w1617 -> [w1624] mode=indexing
              tunnel: FALSE ("SO2 Flush") -> [w1623]
              tunnel: w1615 -> [w1622]
              tunnel: w1614 -> [w1621]
              tunnel: [w1620] -> w1613
              tunnel: [w1619] -> w1612
              n637 = Bundle(cluster=T4 {"Message"="", "Message Data"=variant} ("Message Cluster"), "Message"=w1624, "Message Data"=w1623) -> (w1625:T4)
              n638 = Enqueue Element(queue=w1622, element=w1625, error in (no error)=w1621) -> (queue out=w1620:refnum<queue>, error out=w1619:errorcluster)  [unwired: 1 in, 1 out]
            }
          }
          frame #8 {
            w1629 = 0.0 ("MFC_2\nSLPM Value")
            n639 = local write "MFC_2\nSLPM Value"(w1629) -> ()
            n640 = Bundle(cluster=T4 {"Message"="", "Message Data"=variant} ("Message Cluster"), "Message"="MFC_2", "Message Data"=w1629) -> (w1632:T4)
            n641 = Enqueue Element(queue=w1631, element=w1632, error in (no error)=w1630) -> (queue out=w1628:refnum<queue>, error out=w1627:errorcluster)  [unwired: 1 in, 1 out]
          }
          frame #9 {
            w1637 = FALSE ("SO2 Flush")
            n642 = local write "eV8"(w1637) -> ()
            n643 = local write "eV9"(w1637) -> ()
          }
          frame #10 {
            n644 = for {
              N: "Auto Zeroing \ninterval (sec)" -> [w1653]
              tunnel: [w1648] -> w1640
              i -> [w1652]
              stop <- w1648 stop-if-true
              n645 = local read "SO2 Pause\nAuto Zeroing"() -> (w1646:bool)
              n646 = Subtract(x=w1653, y=w1652) -> (x-y=w1654:i32)
              n647 = Equal?(x=w1646, y=TRUE) -> (x = y?=w1644:bool)
              n648 = Decrement(x=w1654) -> (x-1=→"Next Auto Zero\nStarts in (sec)":i32)
              n649 = Wait (ms)(milliseconds to wait=u32 1000) -> ()  [unwired: 1 out]
              n650 = case shown="True" w1644 {
                selector: w1644 -> [w1656 _]
                tunnel: [w1656 FALSE] -> w1643
                frame False {
                }
                frame True {
                  n651 = for {
                    N: "Pause Auto Zero Count \nDown set time (sec)" -> [w1670]
                    tunnel: [w1662] -> w1658
                    i -> [w1669]
                    stop <- w1662 stop-if-true
                    w1663 = FALSE
                    n652 = local read "SO2 Pause\nAuto Zeroing"() -> (w1665:bool)
                    n653 = local read "SO2 Auto Zeroing"() -> (w1666:bool)
                    n654 = Subtract(x=w1670, y=w1669) -> (x-y=w1671:i32)
                    n655 = Decrement(x=w1671) -> (x-1=→"SO2 Resume Zeroing\nCount down timer (sec)":i32)
                    n656 = Wait (ms)(milliseconds to wait=u32 1000) -> ()  [unwired: 1 out]
                    n657 = Equal?(x=w1666, y=w1663) -> (x = y?=w1667:bool)
                    n658 = Equal?(x=w1665, y=w1663) -> (x = y?=w1664:bool)
                    n659 = Or(x=w1667, y=w1664) -> (x .or. y?=w1662:bool)
                  }
                  n660 = case shown="True" w1658 {
                    frame False {
                    }
                    frame True {
                      n661 = local write "SO2 Resume Zeroing\nCount down timer (sec)"(u32 0 ("SO2 Resume Zeroing\nCount down timer (sec)")) -> ()
                    }
                  }
                  n662 = local write "Auto Zero\nIndicator"("Auto Zero Paused" ("Auto Zero\nIndicator")) -> ()
                }
              }
              n663 = local write "Auto Zero\nIndicator"("Waiting For The Next Zeroing\nInterrupt Waiting by Pressing Pause Auto Zeroing button " ("Auto Zero\nIndicator")) -> ()
              n664 = local read "SO2 Auto Zeroing"() -> (w1649:bool)
              n665 = local write "SO2 Pause\nAuto Zeroing"(w1643) -> ()
              n666 = Equal?(x=w1649, y=FALSE) -> (x = y?=w1648:bool)
            }
            n667 = case shown="True" w1640 {
              frame False {
              }
              frame True {
                n668 = local write "Next Auto Zero\nStarts in (sec)"(u32 0 ("Next Auto Zero\nStarts in (sec)")) -> ()
              }
            }
          }
          frame #11 {
            n669 = Bundle(cluster=T4 {"Message"="", "Message Data"=variant} ("Message Cluster"), "Message"="Auto_zero", "Message Data"=FALSE) -> (w1677:T4)
            n670 = Enqueue Element(queue=w1674, element=w1677, error in (no error)=w1673) -> ()  [unwired: 1 in, 3 out]
          }
        }
      }
    }
    n671 = Wait (ms)(milliseconds to wait=u32 100) -> ()  [unwired: 1 out]
  }
  n672 = while {
    tunnel: w2 -> [w1682]
    tunnel: w1 -> [w1681]
    tunnel: [w1679] -> _
    stop <- FALSE stop-if-true
    # "SO2 UI Event Handler Loop"
    n673 = event shown="[3] \"SO2 GND Zeroing\": Value Change" {
      selector: _ -> [_ _ _ _ _ _ _ _ _ _ _ _ _ _ _ _ _ _ _ _ _ _ _ _ _ _ _ _]
      dyn-events: _ -> [_ _ _ _ _ _ _ _ _ _ _ _ _ _ _ _ _ _ _ _ _ _ _ _ _ _ _ _]
      timeout: _ -> [_ _ _ _ _ _ _ _ _ _ _ _ _ _ _ _ _ _ _ _ _ _ _ _ _ _ _ _]
      tunnel: w1682 -> [w1689 w1701 w1745 w1756 w1789 w1828 w1892 w1898 w1909 w1912 w1920 w1926 w1933 w1939 w1945 w1955 w1959 w1966 w1973 w1980 w1987 w1994 w2001 w2008 w2015 w2022 w2030 w2044]
      tunnel: w1681 -> [w1688 w1700 w1744 w1755 w1788 w1827 w1891 w1897 w1908 w1911 w1918 w1925 w1932 w1938 w1944 w1954 w1958 w1965 w1972 w1979 w1986 w1993 w2000 w2007 w2014 w2021 w2029 w2043]
      tunnel: [w1683 w1699 _ w1754 w1787 _ _ _ w1903 w1910 w1917 _ w1931 _ _ w1949 w1957 w1964 w1971 w1978 w1985 w1992 w1999 w2006 w2013 w2020 w2028 w2042] -> w1679
      event "eV9": Value Change {
        n674 = event-data() -> ("NewVal"=w1686:bool)  [unwired: 1 in]
        n675 = Bundle(cluster=T4 {"Message"="", "Message Data"=variant} ("Message Cluster"), "Message"="V9", "Message Data"=w1686) -> (w1684:T4)
        n676 = Enqueue Element(queue=w1689, element=w1684, error in (no error)=w1688) -> (error out=w1683:errorcluster)  [unwired: 1 in, 2 out]
      }
      event "SO2 Flush": Value Change {
        n677 = event-data() -> ()  [unwired: 1 in, 1 out]
        n678 = flat-sequence {
          tunnel: w1701 -> [w1709]
          tunnel: w1700 -> [w1708]
          tunnel: [w1704] -> w1696
          tunnel: [w1702] -> w1694
          tunnel: w1696 -> [w1711]
          tunnel: [w1713] -> w1695
          tunnel: w1694 -> [w1712]
          tunnel: [w1714] -> w1693
          tunnel: w1695 -> [w1720]
          tunnel: [w1720] -> w1698
          tunnel: [w1718] -> w1697
          tunnel: w1693 -> [w1718]
          tunnel: w1698 -> [w1729]
          tunnel: [w1728] -> w1692
          tunnel: w1697 -> [w1730]
          tunnel: [w1726] -> w1690
          tunnel: w1692 -> [w1736]
          tunnel: [w1737] -> w1691
          tunnel: w1690 -> [w1735]
          tunnel: [w1742] -> w1699
          tunnel: w1691 -> [w1742]
          frame #0 {
            w1703 = TRUE ("SO2 Flush")
            n679 = Bundle(cluster=T4 {"Message"="", "Message Data"=variant} ("Message Cluster"), "Message"="V9", "Message Data"=w1703) -> (w1705:T4)
            n680 = local write "eV9"(w1703) -> ()
            n681 = Enqueue Element(queue=w1709, element=w1705, error in (no error)=w1708) -> (queue out=w1702:refnum<queue>, error out=w1704:errorcluster)  [unwired: 1 in, 1 out]
          }
          frame #1 {
            n682 = local read "MFC_2 User Set Value"() -> (w1710:dbl)
            n683 = local write "MFC_2\nSLPM Value"(w1710) -> ()
            n684 = Bundle(cluster=T4 {"Message"="", "Message Data"=variant} ("Message Cluster"), "Message"="MFC_2", "Message Data"=w1710) -> (w1715:T4)
            n685 = Enqueue Element(queue=w1712, element=w1715, error in (no error)=w1711) -> (queue out=w1714:refnum<queue>, error out=w1713:errorcluster)  [unwired: 1 in, 1 out]
          }
          frame #2 {
            n686 = for {
              N: "eV9 Flush User\nset time (sec)" -> [w1724]
              i -> [w1723]
              n687 = Subtract(x=w1724, y=w1723) -> (x-y=w1722:i32)
              n688 = Decrement(x=w1722) -> (x-1=w1721:i32)
              n689 = local write "SO2 Flush\nTime Remain (sec)"(w1721) -> ()
              n690 = Wait (ms)(milliseconds to wait=u32 1000) -> ()  [unwired: 1 out]
            }
          }
          frame #3 {
            w1727 = FALSE
            n691 = Bundle(cluster=T4 {"Message"="", "Message Data"=variant} ("Message Cluster"), "Message"="V9", "Message Data"=w1727) -> (w1731:T4)
            n692 = local write "eV9"(w1727) -> ()
            n693 = Enqueue Element(queue=w1730, element=w1731, error in (no error)=w1729) -> (queue out=w1726:refnum<queue>, error out=w1728:errorcluster)  [unwired: 1 in, 1 out]
          }
          frame #4 {
            w1734 = 0.0 ("MFC_2\nSLPM Value")
            n694 = local write "MFC_2\nSLPM Value"(w1734) -> ()
            n695 = Bundle(cluster=T4 {"Message"="", "Message Data"=variant} ("Message Cluster"), "Message"="MFC_2", "Message Data"=w1734) -> (w1738:T4)
            n696 = Enqueue Element(queue=w1735, element=w1738, error in (no error)=w1736) -> (error out=w1737:errorcluster)  [unwired: 1 in, 2 out]
          }
          frame #5 {
            n697 = local write "SO2 Flush"(FALSE ("SO2 Flush")) -> ()
          }
        }
      }
      event "Auto Zeroing \ninterval (sec)": Value Change {
        n698 = event-data() -> ("NewVal"=w1743:i32)  [unwired: 1 in]
        n699 = Bundle(cluster=T4 {"Message"="", "Message Data"=variant} ("Message Cluster"), "Message"="zeroing_interval", "Message Data"=w1743) -> (w1746:T4)
        n700 = Enqueue Element(queue=w1745, element=w1746, error in (no error)=w1744) -> ()  [unwired: 1 in, 3 out]
      }
      event "SO2 GND Zeroing": Value Change {
        n701 = event-data() -> ()  [unwired: 1 in, 1 out]
        n702 = flat-sequence {
          tunnel: w1756 -> [w1764]
          tunnel: w1755 -> [w1763]
          tunnel: [w1759] -> w1753
          tunnel: [w1757] -> w1749
          tunnel: w1753 -> [w1767]
          tunnel: [w1767] -> w1752
          tunnel: [w1766] -> w1750
          tunnel: w1749 -> [w1766]
          tunnel: w1752 -> [w1775]
          tunnel: [w1774] -> w1751
          tunnel: w1750 -> [w1776]
          tunnel: [w1781] -> w1754
          tunnel: w1751 -> [w1781]
          frame #0 {
            w1758 = TRUE ("SO2 Flush")
            n703 = local write "SO2 eV6"(w1758) -> ()
            n704 = Bundle(cluster=T4 {"Message"="", "Message Data"=variant} ("Message Cluster"), "Message"="V6", "Message Data"=w1758) -> (w1760:T4)
            n705 = Enqueue Element(queue=w1764, element=w1760, error in (no error)=w1763) -> (queue out=w1757:refnum<queue>, error out=w1759:errorcluster)  [unwired: 1 in, 1 out]
          }
          frame #1 {
            # "10 Mins Count down"
            n706 = for {
              N: "eV6 User\nset time (sec)" -> [w1771]
              i -> [w1770]
              n707 = Subtract(x=w1771, y=w1770) -> (x-y=w1769:i32)
              n708 = Decrement(x=w1769) -> (x-1=w1768:i32)
              n709 = local write "SO2 Zeroing\nTime Remain (sec)"(w1768) -> ()
              n710 = Wait (ms)(milliseconds to wait=u32 1000) -> ()  [unwired: 1 out]
            }
          }
          frame #2 {
            w1773 = FALSE
            n711 = Bundle(cluster=T4 {"Message"="", "Message Data"=variant} ("Message Cluster"), "Message"="V6", "Message Data"=w1773) -> (w1777:T4)
            n712 = local write "SO2 eV6"(w1773) -> ()
            n713 = Enqueue Element(queue=w1776, element=w1777, error in (no error)=w1775) -> (error out=w1774:errorcluster)  [unwired: 1 in, 2 out]
          }
          frame #3 {
            n714 = local write "SO2 GND Zeroing"(FALSE ("SO2 Flush")) -> ()
          }
        }
      }
      event "SO2 Inflight \nZeroing": Value Change {
        n715 = event-data() -> ()  [unwired: 1 in, 1 out]
        n716 = flat-sequence {
          tunnel: w1789 -> [w1797]
          tunnel: w1788 -> [w1796]
          tunnel: [w1792] -> w1786
          tunnel: [w1790] -> w1782
          tunnel: w1786 -> [w1800]
          tunnel: [w1800] -> w1785
          tunnel: [w1799] -> w1783
          tunnel: w1782 -> [w1799]
          tunnel: w1785 -> [w1808]
          tunnel: [w1807] -> w1784
          tunnel: w1783 -> [w1809]
          tunnel: [w1814] -> w1787
          tunnel: w1784 -> [w1814]
          frame #0 {
            w1791 = TRUE ("SO2 Flush")
            n717 = local write "SO2 eV6"(w1791) -> ()
            n718 = Bundle(cluster=T4 {"Message"="", "Message Data"=variant} ("Message Cluster"), "Message"="V6", "Message Data"=w1791) -> (w1793:T4)
            n719 = Enqueue Element(queue=w1797, element=w1793, error in (no error)=w1796) -> (queue out=w1790:refnum<queue>, error out=w1792:errorcluster)  [unwired: 1 in, 1 out]
          }
          frame #1 {
            n720 = for {
              N: "eV6 User set time \n(Inflight) (sec)" -> [w1804]
              i -> [w1803]
              n721 = Subtract(x=w1804, y=w1803) -> (x-y=w1802:i32)
              n722 = Decrement(x=w1802) -> (x-1=w1801:i32)
              n723 = local write "SO2 Zeroing (Inflight)\nTime Remain (sec)"(w1801) -> ()
              n724 = Wait (ms)(milliseconds to wait=u32 1000) -> ()  [unwired: 1 out]
            }
          }
          frame #2 {
            w1806 = FALSE
            n725 = Bundle(cluster=T4 {"Message"="", "Message Data"=variant} ("Message Cluster"), "Message"="V6", "Message Data"=w1806) -> (w1810:T4)
            n726 = local write "SO2 eV6"(w1806) -> ()
            n727 = Enqueue Element(queue=w1809, element=w1810, error in (no error)=w1808) -> (error out=w1807:errorcluster)  [unwired: 1 in, 2 out]
          }
          frame #3 {
            n728 = local write "SO2 Inflight \nZeroing"(FALSE ("SO2 Flush")) -> ()
          }
        }
      }
      event "SO2 CAL/Zero": Value Change {
        n729 = event-data() -> ()  [unwired: 1 in, 1 out]
        n730 = flat-sequence {
          tunnel: w1828 -> [w1836]
          tunnel: w1827 -> [w1835]
          tunnel: [w1831] -> w1826
          tunnel: [w1830] -> w1824
          tunnel: w1826 -> [w1840]
          tunnel: [w1839] -> w1825
          tunnel: w1824 -> [w1841]
          tunnel: [w1837] -> w1822
          tunnel: w1825 -> [w1847]
          tunnel: [w1847] -> w1823
          tunnel: w1822 -> [w1845]
          tunnel: [w1845] -> w1821
          tunnel: w1823 -> [w1856]
          tunnel: w1821 -> [w1857]
          tunnel: [w1854] -> w1819
          tunnel: [w1853] -> w1817
          tunnel: [w1862] -> w1820
          tunnel: w1819 -> [w1862]
          tunnel: [w1861] -> w1818
          tunnel: w1817 -> [w1861]
          tunnel: w1820 -> [w1872]
          tunnel: w1818 -> [w1871]
          tunnel: [w1870] -> w1816
          tunnel: [w1869] -> w1815
          tunnel: w1816 -> [w1886]
          tunnel: w1815 -> [w1885]
          frame #0 {
            w1829 = TRUE ("SO2 Flush")
            n731 = Bundle(cluster=T4 {"Message"="", "Message Data"=variant} ("Message Cluster"), "Message"="V9", "Message Data"=w1829) -> (w1832:T4)
            n732 = local write "eV9"(w1829) -> ()
            n733 = Enqueue Element(queue=w1836, element=w1832, error in (no error)=w1835) -> (queue out=w1830:refnum<queue>, error out=w1831:errorcluster)  [unwired: 1 in, 1 out]
          }
          frame #1 {
            n734 = local read "MFC_2 User Set Value"() -> (w1838:dbl)
            n735 = local write "MFC_2\nSLPM Value"(w1838) -> ()
            n736 = Bundle(cluster=T4 {"Message"="", "Message Data"=variant} ("Message Cluster"), "Message"="MFC_2", "Message Data"=w1838) -> (w1842:T4)
            n737 = Enqueue Element(queue=w1841, element=w1842, error in (no error)=w1840) -> (queue out=w1837:refnum<queue>, error out=w1839:errorcluster)  [unwired: 1 in, 1 out]
          }
          frame #2 {
            n738 = for {
              N: "eV9 flush User\nset time (sec)" -> [w1851]
              i -> [w1850]
              n739 = Subtract(x=w1851, y=w1850) -> (x-y=w1849:i32)
              n740 = Decrement(x=w1849) -> (x-1=w1848:i32)
              n741 = local write "SO2 Cal/Zero Flush\nTime Remain (sec)"(w1848) -> ()
              n742 = Wait (ms)(milliseconds to wait=u32 1000) -> ()  [unwired: 1 out]
            }
          }
          frame #3 {
            w1855 = TRUE ("SO2 Flush")
            n743 = Bundle(cluster=T4 {"Message"="", "Message Data"=variant} ("Message Cluster"), "Message"="V8", "Message Data"=w1855) -> (w1858:T4)
            n744 = local write "eV8"(w1855) -> ()
            n745 = Enqueue Element(queue=w1857, element=w1858, error in (no error)=w1856) -> (queue out=w1854:refnum<queue>, error out=w1853:errorcluster)  [unwired: 1 in, 1 out]
          }
          frame #4 {
            n746 = for {
              N: "eV8 User\nset time (sec)" -> [w1867]
              i -> [w1866]
              n747 = Subtract(x=w1867, y=w1866) -> (x-y=w1865:i32)
              n748 = Decrement(x=w1865) -> (x-1=w1864:i32)
              n749 = local write "SO2 CAL/Zero\nTime Remain (sec)"(w1864) -> ()
              n750 = Wait (ms)(milliseconds to wait=u32 1000) -> ()  [unwired: 1 out]
            }
          }
          frame #5 {
            n751 = Cluster To Array(cluster=cluster{"Message":string, "Message 2":string} {"Message"="V8", "Message 2"="V9"}) -> (array=w1874:string[])
            n752 = for {
              tunnel: w1874 -> [w1881] mode=indexing
              tunnel: FALSE ("SO2 Flush") -> [w1880]
              tunnel: w1872 -> [w1879]
              tunnel: w1871 -> [w1878]
              tunnel: [w1877] -> w1870
              tunnel: [w1876] -> w1869
              n753 = Bundle(cluster=T4 {"Message"="", "Message Data"=variant} ("Message Cluster"), "Message"=w1881, "Message Data"=w1880) -> (w1882:T4)
              n754 = Enqueue Element(queue=w1879, element=w1882, error in (no error)=w1878) -> (queue out=w1877:refnum<queue>, error out=w1876:errorcluster)  [unwired: 1 in, 1 out]
            }
          }
          frame #6 {
            w1884 = 0.0 ("MFC_2\nSLPM Value")
            n755 = local write "MFC_2\nSLPM Value"(w1884) -> ()
            n756 = Bundle(cluster=T4 {"Message"="", "Message Data"=variant} ("Message Cluster"), "Message"="MFC_2", "Message Data"=w1884) -> (w1887:T4)
            n757 = Enqueue Element(queue=w1886, element=w1887, error in (no error)=w1885) -> ()  [unwired: 1 in, 3 out]
          }
          frame #7 {
            w1890 = FALSE ("SO2 Flush")
            n758 = local write "SO2 CAL/Zero"(w1890) -> ()
            n759 = local write "eV9"(w1890) -> ()
            n760 = local write "eV8"(w1890) -> ()
          }
        }
      }
      event "eV8 User\nset time (sec)": Value Change {
        n761 = event-data() -> ("NewVal"=w1893:i32)  [unwired: 1 in]
        n762 = Bundle(cluster=T4 {"Message"="", "Message Data"=variant} ("Message Cluster"), "Message"="eV8_user_set_time", "Message Data"=w1893) -> (w1894:T4)
        n763 = Enqueue Element(queue=w1892, element=w1894, error in (no error)=w1891) -> ()  [unwired: 1 in, 3 out]
      }
      event "Offset Mean Zero Calculation (default = ON)\nOFF = User input\nOn = Mean zero calculated with ev8": Value Change {
        n764 = event-data() -> ("NewVal"=w1899:bool)  [unwired: 1 in]
        n765 = Bundle(cluster=T4 {"Message"="", "Message Data"=variant} ("Message Cluster"), "Message"="mean_cal_status", "Message Data"=w1899) -> (w1900:T4)
        n766 = Enqueue Element(queue=w1898, element=w1900, error in (no error)=w1897) -> ()  [unwired: 1 in, 3 out]
      }
      event "MFC_2\nSLPM Value": Value Change {
        n767 = event-data() -> ("NewVal"=w1906:dbl)  [unwired: 1 in]
        n768 = Bundle(cluster=T4 {"Message"="", "Message Data"=variant} ("Message Cluster"), "Message"="MFC_2", "Message Data"=w1906) -> (w1904:T4)
        n769 = Enqueue Element(queue=w1909, element=w1904, error in (no error)=w1908) -> (error out=w1903:errorcluster)  [unwired: 1 in, 2 out]
      }
      event "SO2 Inflight MOCCA Alarm\n(default = OFF)": Value Change {
        n770 = event-data() -> ("NewVal"=w1913:bool)  [unwired: 1 in]
        n771 = Bundle(cluster=T4 {"Message"="", "Message Data"=variant} ("Message Cluster"), "Message"="SO2_MOCCA_Alarm", "Message Data"=w1913) -> (w1914:T4)
        n772 = Enqueue Element(queue=w1912, element=w1914, error in (no error)=w1911) -> (error out=w1910:errorcluster)  [unwired: 1 in, 2 out]
      }
      event "MOCCA window \ndelay time (sec)": Value Change {
        n773 = event-data() -> ("NewVal"=w1919:i32)  [unwired: 1 in]
        n774 = Bundle(cluster=T4 {"Message"="", "Message Data"=variant} ("Message Cluster"), "Message"="MOCCA_window_delay_time", "Message Data"=w1919) -> (w1921:T4)
        n775 = Enqueue Element(queue=w1920, element=w1921, error in (no error)=w1918) -> (error out=w1917:errorcluster)  [unwired: 1 in, 2 out]
      }
      event "MOCCA Limit": Value Change {
        n776 = event-data() -> ("NewVal"=w1924:i32)  [unwired: 1 in]
        n777 = Bundle(cluster=T4 {"Message"="", "Message Data"=variant} ("Message Cluster"), "Message"="MOCCA_limit", "Message Data"=w1924) -> (w1927:T4)
        n778 = Enqueue Element(queue=w1926, element=w1927, error in (no error)=w1925) -> ()  [unwired: 1 in, 3 out]
      }
      event "Save Calibration gas\ncylinder concentration to file": Value Change {
        n779 = event-data() -> ("NewVal"=w1930:bool)  [unwired: 1 in]
        n780 = Bundle(cluster=T4 {"Message"="", "Message Data"=variant} ("Message Cluster"), "Message"="calcon_save", "Message Data"=w1930) -> (w1934:T4)
        n781 = Enqueue Element(queue=w1933, element=w1934, error in (no error)=w1932) -> (error out=w1931:errorcluster)  [unwired: 1 in, 2 out]
      }
      event "Calibration gas cylinder \nconcentration (ppb)": Value Change {
        n782 = event-data() -> ("NewVal"=w1937:dbl)  [unwired: 1 in]
        n783 = Bundle(cluster=T4 {"Message"="", "Message Data"=variant} ("Message Cluster"), "Message"="cal_gas_cylin_conc", "Message Data"=w1937) -> (w1940:T4)
        n784 = Enqueue Element(queue=w1939, element=w1940, error in (no error)=w1938) -> ()  [unwired: 1 in, 3 out]
      }
      event "Simulate MOCCA Conc": Value Change {
        n785 = event-data() -> ("NewVal"=w1943:dbl)  [unwired: 1 in]
        n786 = Bundle(cluster=T4 {"Message"="", "Message Data"=variant} ("Message Cluster"), "Message"="sim_MOCCA_conc", "Message Data"=w1943) -> (w1946:T4)
        n787 = Enqueue Element(queue=w1945, element=w1946, error in (no error)=w1944) -> ()  [unwired: 1 in, 3 out]
      }
      event "MFC_3\nSLPM Value": Value Change {
        n788 = event-data() -> ("NewVal"=w1952:dbl)  [unwired: 1 in]
        n789 = Bundle(cluster=T4 {"Message"="", "Message Data"=variant} ("Message Cluster"), "Message"="MFC_3", "Message Data"=w1952) -> (w1950:T4)
        n790 = Enqueue Element(queue=w1955, element=w1950, error in (no error)=w1954) -> (error out=w1949:errorcluster)  [unwired: 1 in, 2 out]
      }
      event "eV8": Value Change {
        n791 = event-data() -> ("NewVal"=w1956:bool)  [unwired: 1 in]
        n792 = Bundle(cluster=T4 {"Message"="", "Message Data"=variant} ("Message Cluster"), "Message"="V8", "Message Data"=w1956) -> (w1960:T4)
        n793 = Enqueue Element(queue=w1959, element=w1960, error in (no error)=w1958) -> (error out=w1957:errorcluster)  [unwired: 1 in, 2 out]
      }
      event "SO2 eV6": Value Change {
        n794 = event-data() -> ("NewVal"=w1963:bool)  [unwired: 1 in]
        n795 = Bundle(cluster=T4 {"Message"="", "Message Data"=variant} ("Message Cluster"), "Message"="V6", "Message Data"=w1963) -> (w1967:T4)
        n796 = Enqueue Element(queue=w1966, element=w1967, error in (no error)=w1965) -> (error out=w1964:errorcluster)  [unwired: 1 in, 2 out]
      }
      event "Simulate Conc": Value Change {
        n797 = event-data() -> ("NewVal"=w1970:bool)  [unwired: 1 in]
        n798 = Bundle(cluster=T4 {"Message"="", "Message Data"=variant} ("Message Cluster"), "Message"="Simulate Conc", "Message Data"=w1970) -> (w1974:T4)
        n799 = Enqueue Element(queue=w1973, element=w1974, error in (no error)=w1972) -> (error out=w1971:errorcluster)  [unwired: 1 in, 2 out]
      }
      event "SO2 UDP Time Offset": Value Change {
        n800 = event-data() -> ("NewVal"=w1977:i32)  [unwired: 1 in]
        n801 = Bundle(cluster=T4 {"Message"="", "Message Data"=variant} ("Message Cluster"), "Message"="UDP Time Offset", "Message Data"=w1977) -> (w1981:T4)
        n802 = Enqueue Element(queue=w1980, element=w1981, error in (no error)=w1979) -> (error out=w1978:errorcluster)  [unwired: 1 in, 2 out]
      }
      event "Simulate STEL Conc": Value Change {
        n803 = event-data() -> ("NewVal"=w1984:dbl)  [unwired: 1 in]
        n804 = Bundle(cluster=T4 {"Message"="", "Message Data"=variant} ("Message Cluster"), "Message"="Simulate STEL Conc", "Message Data"=w1984) -> (w1988:T4)
        n805 = Enqueue Element(queue=w1987, element=w1988, error in (no error)=w1986) -> (error out=w1985:errorcluster)  [unwired: 1 in, 2 out]
      }
      event "Simulate TWA Conc": Value Change {
        n806 = event-data() -> ("NewVal"=w1991:dbl)  [unwired: 1 in]
        n807 = Bundle(cluster=T4 {"Message"="", "Message Data"=variant} ("Message Cluster"), "Message"="Simulate TWA Conc", "Message Data"=w1991) -> (w1995:T4)
        n808 = Enqueue Element(queue=w1994, element=w1995, error in (no error)=w1993) -> (error out=w1992:errorcluster)  [unwired: 1 in, 2 out]
      }
      event "10mins STEL Limit": Value Change {
        n809 = event-data() -> ("NewVal"=w1998:i32)  [unwired: 1 in]
        n810 = Bundle(cluster=T4 {"Message"="", "Message Data"=variant} ("Message Cluster"), "Message"="10mins STEL Limit", "Message Data"=w1998) -> (w2002:T4)
        n811 = Enqueue Element(queue=w2001, element=w2002, error in (no error)=w2000) -> (error out=w1999:errorcluster)  [unwired: 1 in, 2 out]
      }
      event "8hr TWA Limit": Value Change {
        n812 = event-data() -> ("NewVal"=w2005:i32)  [unwired: 1 in]
        n813 = Bundle(cluster=T4 {"Message"="", "Message Data"=variant} ("Message Cluster"), "Message"="8hr TWA Limit", "Message Data"=w2005) -> (w2009:T4)
        n814 = Enqueue Element(queue=w2008, element=w2009, error in (no error)=w2007) -> (error out=w2006:errorcluster)  [unwired: 1 in, 2 out]
      }
      event "SO2 Zero": Value Change {
        n815 = event-data() -> ("NewVal"=w2012:dbl)  [unwired: 1 in]
        n816 = Bundle(cluster=T4 {"Message"="", "Message Data"=variant} ("Message Cluster"), "Message"="Offset", "Message Data"=w2012) -> (w2016:T4)
        n817 = Enqueue Element(queue=w2015, element=w2016, error in (no error)=w2014) -> (error out=w2013:errorcluster)  [unwired: 1 in, 2 out]
      }
      event "SO2 Sensitivity": Value Change {
        n818 = event-data() -> ("NewVal"=w2019:dbl)  [unwired: 1 in]
        n819 = Bundle(cluster=T4 {"Message"="", "Message Data"=variant} ("Message Cluster"), "Message"="Slope", "Message Data"=w2019) -> (w2023:T4)
        n820 = Enqueue Element(queue=w2022, element=w2023, error in (no error)=w2021) -> (error out=w2020:errorcluster)  [unwired: 1 in, 2 out]
      }
      event "Confirm Flight Number": Value Change {
        n821 = event-data() -> ()  [unwired: 1 in, 6 out]
        n822 = flat-sequence {
          tunnel: w2029 -> [w2032]
          tunnel: w2030 -> [w2033]
          tunnel: [w2033] -> w2027
          tunnel: [w2032] -> w2026
          tunnel: [w2035] -> w2028
          tunnel: w2027 -> [w2037]
          tunnel: w2026 -> [w2036]
          frame #0 {
            n823 = local write "cRIO File IO Stop\n(USB Flash Drive Unmount)"(FALSE ("cRIO File IO Stop\n(USB Flash Drive Unmount)")) -> ()
          }
          frame #1 {
            n824 = local read "Flight Number"() -> (w2034:string)
            n825 = Bundle(cluster=T4 {"Message"="", "Message Data"=variant} ("Message Cluster"), "Message"="Flight Number", "Message Data"=w2034) -> (w2038:T4)
            n826 = Enqueue Element(queue=w2037, element=w2038, error in (no error)=w2036) -> (error out=w2035:errorcluster)  [unwired: 1 in, 2 out]
          }
        }
      }
      event "cRIO File IO Stop\n(USB Flash Drive Unmount)": Value Change {
        n827 = event-data() -> ("NewVal"=w2041:bool)  [unwired: 1 in]
        n828 = Bundle(cluster=T4 {"Message"="", "Message Data"=variant} ("Message Cluster"), "Message"="Stop File Write", "Message Data"=w2041) -> (w2045:T4)
        n829 = Enqueue Element(queue=w2044, element=w2045, error in (no error)=w2043) -> (error out=w2042:errorcluster)  [unwired: 1 in, 2 out]
      }
    }
    "SO2 Event error out" <- w1679
  }
  n830 = Create Network Stream Writer Endpoint(6:w44, 7:10 ("writer buffer size"), 9:w39, 10:"//192.168.101.17/command/reader/SO2" ("reader url"), 11:"/command/writer/SO2" ("writer name")) -> (0:w43:errorcluster, 3:w42:refnum<k21>)  [unwired: 2 in]
  n831 = while {
    tunnel: w2 -> [w2055]
    shift-right: [w2050] -> _
    shift-left: w42 -> [w2052]
    shift-right: [w2048] -> w40
    shift-left: w43 -> [w2054]
    tunnel: w1 -> [w2049]
    stop <- w2048 stop-if-true
    # "SO2 UI Command Sender"
    n832 = Dequeue Element(queue=w2055, error in (no error)=w2049) -> (element=w2051:T4)  [unwired: 1 in, 3 out]
    n833 = Unbundle By Name(w2051) -> ("Message"=w2053:string)
    n834 = case shown="\"zeroing_interval\"" w2053 {
      tunnel: w2054 -> [w2056 w2060 w2067 w2074 w2081 w2088 w2095 w2102 w2109 w2116 w2123 w2130 w2137 w2144 w2151 w2158 w2165 w2172 w2179 w2186 w2193 w2200 w2207 w2214 w2221 w2228]
      tunnel: w2052 -> [w2057 w2063 w2070 w2077 w2084 w2091 w2098 w2105 w2112 w2119 w2126 w2133 w2140 w2147 w2154 w2161 w2168 w2175 w2182 w2189 w2196 w2203 w2210 w2217 w2224 w2231]
      tunnel: w2051 -> [_ w2062 w2069 w2076 w2083 w2090 w2097 w2104 w2111 w2118 w2125 w2132 w2139 w2146 w2153 w2160 w2167 w2174 w2181 w2188 w2195 w2202 w2209 w2216 w2223 w2230]
      tunnel: [w2056 w2059 w2066 w2073 w2080 w2087 w2094 w2101 w2108 w2115 w2122 w2129 w2136 w2143 w2150 w2157 w2164 w2171 w2178 w2185 w2192 w2199 w2206 w2213 w2220 w2227] -> w2048
      tunnel: [w2057 w2058 w2065 w2072 w2079 w2086 w2093 w2100 w2107 w2114 w2121 w2128 w2135 w2142 w2149 w2156 w2163 w2170 w2177 w2184 w2191 w2198 w2205 w2212 w2219 w2226] -> w2050
      frame "False", Default {
      }
      frame "V9" {
        n835 = shared-variable-write(w2063, w2060, w2062) -> (w2061:refnum<k21>, w2064:errorcluster)  [unwired: 1 in, 1 out]
        n836 = Flush Stream(8:w2064, 11:w2061) -> (0:w2059:errorcluster, 3:w2058:refnum<k21>)  [unwired: 2 in, 1 out]
      }
      frame "MFC_2" {
        n837 = shared-variable-write(w2070, w2067, w2069) -> (w2068:refnum<k21>, w2071:errorcluster)  [unwired: 1 in, 1 out]
        n838 = Flush Stream(8:w2071, 11:w2068) -> (0:w2066:errorcluster, 3:w2065:refnum<k21>)  [unwired: 2 in, 1 out]
      }
      frame "MFC_3" {
        n839 = shared-variable-write(w2077, w2074, w2076) -> (w2075:refnum<k21>, w2078:errorcluster)  [unwired: 1 in, 1 out]
        n840 = Flush Stream(8:w2078, 11:w2075) -> (0:w2073:errorcluster, 3:w2072:refnum<k21>)  [unwired: 2 in, 1 out]
      }
      frame "V6" {
        n841 = shared-variable-write(w2084, w2081, w2083) -> (w2082:refnum<k21>, w2085:errorcluster)  [unwired: 1 in, 1 out]
        n842 = Flush Stream(8:w2085, 11:w2082) -> (0:w2080:errorcluster, 3:w2079:refnum<k21>)  [unwired: 2 in, 1 out]
      }
      frame "Simulate Conc" {
        n843 = shared-variable-write(w2091, w2088, w2090) -> (w2089:refnum<k21>, w2092:errorcluster)  [unwired: 1 in, 1 out]
        n844 = Flush Stream(8:w2092, 11:w2089) -> (0:w2087:errorcluster, 3:w2086:refnum<k21>)  [unwired: 2 in, 1 out]
      }
      frame "Simulate STEL Conc" {
        n845 = shared-variable-write(w2098, w2095, w2097) -> (w2096:refnum<k21>, w2099:errorcluster)  [unwired: 1 in, 1 out]
        n846 = Flush Stream(8:w2099, 11:w2096) -> (0:w2094:errorcluster, 3:w2093:refnum<k21>)  [unwired: 2 in, 1 out]
      }
      frame "Simulate TWA Conc" {
        n847 = shared-variable-write(w2105, w2102, w2104) -> (w2103:refnum<k21>, w2106:errorcluster)  [unwired: 1 in, 1 out]
        n848 = Flush Stream(8:w2106, 11:w2103) -> (0:w2101:errorcluster, 3:w2100:refnum<k21>)  [unwired: 2 in, 1 out]
      }
      frame "10mins STEL Limit" {
        n849 = shared-variable-write(w2112, w2109, w2111) -> (w2110:refnum<k21>, w2113:errorcluster)  [unwired: 1 in, 1 out]
        n850 = Flush Stream(8:w2113, 11:w2110) -> (0:w2108:errorcluster, 3:w2107:refnum<k21>)  [unwired: 2 in, 1 out]
      }
      frame "8hr TWA Limit" {
        n851 = shared-variable-write(w2119, w2116, w2118) -> (w2117:refnum<k21>, w2120:errorcluster)  [unwired: 1 in, 1 out]
        n852 = Flush Stream(8:w2120, 11:w2117) -> (0:w2115:errorcluster, 3:w2114:refnum<k21>)  [unwired: 2 in, 1 out]
      }
      frame "Offset" {
        n853 = shared-variable-write(w2126, w2123, w2125) -> (w2124:refnum<k21>, w2127:errorcluster)  [unwired: 1 in, 1 out]
        n854 = Flush Stream(8:w2127, 11:w2124) -> (0:w2122:errorcluster, 3:w2121:refnum<k21>)  [unwired: 2 in, 1 out]
      }
      frame "eV8_user_set_time" {
        n855 = shared-variable-write(w2133, w2130, w2132) -> (w2131:refnum<k21>, w2134:errorcluster)  [unwired: 1 in, 1 out]
        n856 = Flush Stream(8:w2134, 11:w2131) -> (0:w2129:errorcluster, 3:w2128:refnum<k21>)  [unwired: 2 in, 1 out]
      }
      frame "mean_cal_status" {
        n857 = shared-variable-write(w2140, w2137, w2139) -> (w2138:refnum<k21>, w2141:errorcluster)  [unwired: 1 in, 1 out]
        n858 = Flush Stream(8:w2141, 11:w2138) -> (0:w2136:errorcluster, 3:w2135:refnum<k21>)  [unwired: 2 in, 1 out]
      }
      frame "SO2_MOCCA_Alarm" {
        n859 = shared-variable-write(w2147, w2144, w2146) -> (w2145:refnum<k21>, w2148:errorcluster)  [unwired: 1 in, 1 out]
        n860 = Flush Stream(8:w2148, 11:w2145) -> (0:w2143:errorcluster, 3:w2142:refnum<k21>)  [unwired: 2 in, 1 out]
      }
      frame "MOCCA_window_delay_time" {
        n861 = shared-variable-write(w2154, w2151, w2153) -> (w2152:refnum<k21>, w2155:errorcluster)  [unwired: 1 in, 1 out]
        n862 = Flush Stream(8:w2155, 11:w2152) -> (0:w2150:errorcluster, 3:w2149:refnum<k21>)  [unwired: 2 in, 1 out]
      }
      frame "MOCCA_limit" {
        n863 = shared-variable-write(w2161, w2158, w2160) -> (w2159:refnum<k21>, w2162:errorcluster)  [unwired: 1 in, 1 out]
        n864 = Flush Stream(8:w2162, 11:w2159) -> (0:w2157:errorcluster, 3:w2156:refnum<k21>)  [unwired: 2 in, 1 out]
      }
      frame "calcon_save" {
        n865 = shared-variable-write(w2168, w2165, w2167) -> (w2166:refnum<k21>, w2169:errorcluster)  [unwired: 1 in, 1 out]
        n866 = Flush Stream(8:w2169, 11:w2166) -> (0:w2164:errorcluster, 3:w2163:refnum<k21>)  [unwired: 2 in, 1 out]
      }
      frame "Auto_zero" {
        n867 = shared-variable-write(w2175, w2172, w2174) -> (w2173:refnum<k21>, w2176:errorcluster)  [unwired: 1 in, 1 out]
        n868 = Flush Stream(8:w2176, 11:w2173) -> (0:w2171:errorcluster, 3:w2170:refnum<k21>)  [unwired: 2 in, 1 out]
      }
      frame "zeroing_interval" {
        n869 = shared-variable-write(w2182, w2179, w2181) -> (w2180:refnum<k21>, w2183:errorcluster)  [unwired: 1 in, 1 out]
        n870 = Flush Stream(8:w2183, 11:w2180) -> (0:w2178:errorcluster, 3:w2177:refnum<k21>)  [unwired: 2 in, 1 out]
      }
      frame "cal_gas_cylin_conc" {
        n871 = shared-variable-write(w2189, w2186, w2188) -> (w2187:refnum<k21>, w2190:errorcluster)  [unwired: 1 in, 1 out]
        n872 = Flush Stream(8:w2190, 11:w2187) -> (0:w2185:errorcluster, 3:w2184:refnum<k21>)  [unwired: 2 in, 1 out]
      }
      frame "sim_MOCCA_conc" {
        n873 = shared-variable-write(w2196, w2193, w2195) -> (w2194:refnum<k21>, w2197:errorcluster)  [unwired: 1 in, 1 out]
        n874 = Flush Stream(8:w2197, 11:w2194) -> (0:w2192:errorcluster, 3:w2191:refnum<k21>)  [unwired: 2 in, 1 out]
      }
      frame "Slope" {
        n875 = shared-variable-write(w2203, w2200, w2202) -> (w2201:refnum<k21>, w2204:errorcluster)  [unwired: 1 in, 1 out]
        n876 = Flush Stream(8:w2204, 11:w2201) -> (0:w2199:errorcluster, 3:w2198:refnum<k21>)  [unwired: 2 in, 1 out]
      }
      frame "Flight Number" {
        n877 = shared-variable-write(w2210, w2207, w2209) -> (w2208:refnum<k21>, w2211:errorcluster)  [unwired: 1 in, 1 out]
        n878 = Flush Stream(8:w2211, 11:w2208) -> (0:w2206:errorcluster, 3:w2205:refnum<k21>)  [unwired: 2 in, 1 out]
      }
      frame "Stop File Write" {
        n879 = shared-variable-write(w2217, w2214, w2216) -> (w2215:refnum<k21>, w2218:errorcluster)  [unwired: 1 in, 1 out]
        n880 = Flush Stream(8:w2218, 11:w2215) -> (0:w2213:errorcluster, 3:w2212:refnum<k21>)  [unwired: 2 in, 1 out]
      }
      frame "UDP Time Offset" {
        n881 = shared-variable-write(w2224, w2221, w2223) -> (w2222:refnum<k21>, w2225:errorcluster)  [unwired: 1 in, 1 out]
        n882 = Flush Stream(8:w2225, 11:w2222) -> (0:w2220:errorcluster, 3:w2219:refnum<k21>)  [unwired: 2 in, 1 out]
      }
      frame "V8" {
        n883 = shared-variable-write(w2231, w2228, w2230) -> (w2229:refnum<k21>, w2232:errorcluster)  [unwired: 1 in, 1 out]
        n884 = Flush Stream(8:w2232, 11:w2229) -> (0:w2227:errorcluster, 3:w2226:refnum<k21>)  [unwired: 2 in, 1 out]
      }
    }
  }
  "SO2 command sender \nerror out" <- w40
  n885 = Obtain Queue(name (unnamed)="TEi43c_Command", element data type=w28) -> (queue out=w37:refnum<queue>, error out=w30:errorcluster)  [unwired: 3 in, 1 out]
  n886 = Create Network Stream Writer Endpoint(6:w34, 7:10 ("writer buffer size"), 9:w28, 10:"//192.168.101.17/command/reader/TEi43c" ("reader url"), 11:"/command/writer/TEi43c" ("writer name")) -> (0:w33:errorcluster, 3:w32:refnum<k21>)  [unwired: 2 in]
  n887 = while {
    tunnel: w37 -> [w2236]
    tunnel: w30 -> [w2235]
    tunnel: [w2233] -> _
    stop <- FALSE stop-if-true
    # "TEi43c Ozone UI Event Handler Loop"
    n888 = event shown="[0] \"Ozone Zeroing\": Value Change" {
      selector: _ -> [_ _ _ _ _]
      dyn-events: _ -> [_ _ _ _ _]
      timeout: _ -> [_ _ _ _ _]
      tunnel: w2236 -> [w2244 w2272 w2280 w2287 w2295]
      tunnel: w2235 -> [w2243 w2271 w2279 w2286 w2294]
      tunnel: [w2242 w2270 w2278 w2285 w2293] -> w2233
      event "Ozone Zeroing": Value Change {
        n889 = event-data() -> ()  [unwired: 1 in, 6 out]
        n890 = flat-sequence {
          tunnel: w2244 -> [w2249]
          tunnel: w2243 -> [w2248]
          tunnel: [w2247] -> w2241
          tunnel: [w2245] -> w2237
          tunnel: w2241 -> [w2255]
          tunnel: [w2255] -> w2240
          tunnel: [w2253] -> w2238
          tunnel: w2237 -> [w2253]
          tunnel: w2240 -> [w2263]
          tunnel: [w2262] -> w2239
          tunnel: w2238 -> [w2264]
          tunnel: [w2269] -> w2242
          tunnel: w2239 -> [w2269]
          frame #0 {
            w2246 = TRUE
            n891 = local write "Ozone eV6"(w2246) -> ()
            n892 = Bundle(cluster=T4 {"Message"="", "Message Data"=variant} ("Message Cluster"), "Message"="V6", "Message Data"=w2246) -> (w2250:T4)
            n893 = Enqueue Element(queue=w2249, element=w2250, error in (no error)=w2248) -> (queue out=w2245:refnum<queue>, error out=w2247:errorcluster)  [unwired: 1 in, 1 out]
          }
          frame #1 {
            # "10 Mins Count down"
            n894 = for {
              N: 600 -> [w2259]
              i -> [w2258]
              n895 = Subtract(x=w2259, y=w2258) -> (x-y=w2257:i32)
              n896 = Decrement(x=w2257) -> (x-1=→"Ozone Zeroing\nTime Remain (sec)":i32)
              n897 = Wait (ms)(milliseconds to wait=u32 1000) -> ()  [unwired: 1 out]
            }
          }
          frame #2 {
            w2261 = FALSE
            n898 = local write "Ozone eV6"(w2261) -> ()
            n899 = Bundle(cluster=T4 {"Message"="", "Message Data"=variant} ("Message Cluster"), "Message"="V6", "Message Data"=w2261) -> (w2265:T4)
            n900 = Enqueue Element(queue=w2264, element=w2265, error in (no error)=w2263) -> (error out=w2262:errorcluster)  [unwired: 1 in, 2 out]
          }
          frame #3 {
            n901 = local write "Ozone Zeroing"(FALSE ("Ozone Zeroing")) -> ()
          }
        }
      }
      event "Ozone eV6": Value Change {
        n902 = event-data() -> ("NewVal"=w2273:bool)  [unwired: 1 in]
        n903 = Bundle(cluster=T4 {"Message"="", "Message Data"=variant} ("Message Cluster"), "Message"="V6", "Message Data"=w2273) -> (w2274:T4)
        n904 = Enqueue Element(queue=w2272, element=w2274, error in (no error)=w2271) -> (error out=w2270:errorcluster)  [unwired: 1 in, 2 out]
      }
      event "cRIO File IO Stop\n(USB Flash Drive Unmount)": Value Change {
        n905 = event-data() -> ("NewVal"=w2277:bool)  [unwired: 1 in]
        n906 = Bundle(cluster=T4 {"Message"="", "Message Data"=variant} ("Message Cluster"), "Message"="Stop File Write", "Message Data"=w2277) -> (w2281:T4)
        n907 = Enqueue Element(queue=w2280, element=w2281, error in (no error)=w2279) -> (error out=w2278:errorcluster)  [unwired: 1 in, 2 out]
      }
      event "Ozone UDP Time Offset": Value Change {
        n908 = event-data() -> ("NewVal"=w2284:i32)  [unwired: 1 in]
        n909 = Bundle(cluster=T4 {"Message"="", "Message Data"=variant} ("Message Cluster"), "Message"="UDP Time Offset", "Message Data"=w2284) -> (w2288:T4)
        n910 = Enqueue Element(queue=w2287, element=w2288, error in (no error)=w2286) -> (error out=w2285:errorcluster)  [unwired: 1 in, 2 out]
      }
      event "Confirm Flight Number": Value Change {
        n911 = event-data() -> ()  [unwired: 1 in, 5 out]
        n912 = flat-sequence {
          tunnel: w2294 -> [w2297]
          tunnel: w2295 -> [w2298]
          tunnel: [w2298] -> w2292
          tunnel: [w2297] -> w2291
          tunnel: [w2300] -> w2293
          tunnel: w2292 -> [w2302]
          tunnel: w2291 -> [w2301]
          frame #0 {
            n913 = local write "cRIO File IO Stop\n(USB Flash Drive Unmount)"(FALSE ("cRIO File IO Stop\n(USB Flash Drive Unmount)")) -> ()
          }
          frame #1 {
            n914 = local read "Flight Number"() -> (w2299:string)
            n915 = Bundle(cluster=T4 {"Message"="", "Message Data"=variant} ("Message Cluster"), "Message"="Flight Number", "Message Data"=w2299) -> (w2303:T4)
            n916 = Enqueue Element(queue=w2302, element=w2303, error in (no error)=w2301) -> (error out=w2300:errorcluster)  [unwired: 1 in, 2 out]
          }
        }
      }
    }
    "Ozone Event error out" <- w2233
  }
  n917 = while {
    tunnel: w37 -> [w2313]
    shift-right: [w2308] -> _
    shift-left: w32 -> [w2310]
    shift-right: [w2306] -> w29
    shift-left: w33 -> [w2312]
    tunnel: w30 -> [w2307]
    stop <- w2306 stop-if-true
    # "TEi43c Ozone UI Command Sender"
    n918 = Dequeue Element(queue=w2313, error in (no error)=w2307) -> (element=w2309:T4)  [unwired: 1 in, 3 out]
    n919 = Unbundle By Name(w2309) -> ("Message"=w2311:string)
    n920 = case shown="\"UDP Time Offset\"" w2311 {
      tunnel: w2312 -> [w2314 w2318 w2325 w2332 w2339]
      tunnel: w2310 -> [w2315 w2321 w2328 w2335 w2342]
      tunnel: w2309 -> [_ w2320 w2327 w2334 w2341]
      tunnel: [w2314 w2317 w2324 w2331 w2338] -> w2306
      tunnel: [w2315 w2316 w2323 w2330 w2337] -> w2308
      frame "False", Default {
      }
      frame "V6" {
        n921 = shared-variable-write(w2321, w2318, w2320) -> (w2319:refnum<k21>, w2322:errorcluster)  [unwired: 1 in, 1 out]
        n922 = Flush Stream(8:w2322, 11:w2319) -> (0:w2317:errorcluster, 3:w2316:refnum<k21>)  [unwired: 2 in, 1 out]
      }
      frame "Stop File Write" {
        n923 = shared-variable-write(w2328, w2325, w2327) -> (w2326:refnum<k21>, w2329:errorcluster)  [unwired: 1 in, 1 out]
        n924 = Flush Stream(8:w2329, 11:w2326) -> (0:w2324:errorcluster, 3:w2323:refnum<k21>)  [unwired: 2 in, 1 out]
      }
      frame "Flight Number" {
        n925 = shared-variable-write(w2335, w2332, w2334) -> (w2333:refnum<k21>, w2336:errorcluster)  [unwired: 1 in, 1 out]
        n926 = Flush Stream(8:w2336, 11:w2333) -> (0:w2331:errorcluster, 3:w2330:refnum<k21>)  [unwired: 2 in, 1 out]
      }
      frame "UDP Time Offset" {
        n927 = shared-variable-write(w2342, w2339, w2341) -> (w2340:refnum<k21>, w2343:errorcluster)  [unwired: 1 in, 1 out]
        n928 = Flush Stream(8:w2343, 11:w2340) -> (0:w2338:errorcluster, 3:w2337:refnum<k21>)  [unwired: 2 in, 1 out]
      }
    }
  }
  "Ozone command sender error out" <- w29
  n929 = Obtain Queue(name (unnamed)="2BOzone_Command", element data type=w16) -> (queue out=w25:refnum<queue>, error out=w18:errorcluster)  [unwired: 3 in, 1 out]
  n930 = Create Network Stream Writer Endpoint(6:w22, 7:10 ("writer buffer size"), 9:w16, 10:"//192.168.101.17/command/reader/2BOzone" ("reader url"), 11:"/command/writer/2BOzone" ("writer name")) -> (0:w21:errorcluster, 3:w20:refnum<k21>)  [unwired: 2 in]
  n931 = while {
    tunnel: w25 -> [w2347]
    tunnel: w18 -> [w2346]
    tunnel: [w2344] -> _
    stop <- FALSE stop-if-true
    # "2BOzone UI Event Handler Loop"
    n932 = event shown="[7] \"Confirm Flight Number\": Value Change" {
      selector: _ -> [_ _ _ _ _ _ _ _]
      dyn-events: _ -> [_ _ _ _ _ _ _ _]
      timeout: _ -> [_ _ _ _ _ _ _ _]
      tunnel: w2347 -> [w2351 w2358 w2365 w2372 w2379 w2386 w2393 w2401]
      tunnel: w2346 -> [w2350 w2357 w2364 w2371 w2378 w2385 w2392 w2400]
      tunnel: [w2349 w2356 w2363 w2370 w2377 w2384 w2391 w2399] -> w2344
      event "Ambient = OFF\nCabin = ON": Value Change {
        n933 = event-data() -> ("NewVal"=w2348:bool)  [unwired: 1 in]
        n934 = Bundle(cluster=T4 {"Message"="", "Message Data"=variant} ("Message Cluster"), "Message"="Ambient/Cabin", "Message Data"=w2348) -> (w2352:T4)
        n935 = Enqueue Element(queue=w2351, element=w2352, error in (no error)=w2350) -> (error out=w2349:errorcluster)  [unwired: 1 in, 2 out]
      }
      event "Simulate 2B Conc": Value Change {
        n936 = event-data() -> ("NewVal"=w2355:bool)  [unwired: 1 in]
        n937 = Bundle(cluster=T4 {"Message"="", "Message Data"=variant} ("Message Cluster"), "Message"="Simulate_conc", "Message Data"=w2355) -> (w2359:T4)
        n938 = Enqueue Element(queue=w2358, element=w2359, error in (no error)=w2357) -> (error out=w2356:errorcluster)  [unwired: 1 in, 2 out]
      }
      event "Simulate Inst Conc": Value Change {
        n939 = event-data() -> ("NewVal"=w2362:i32)  [unwired: 1 in]
        n940 = Bundle(cluster=T4 {"Message"="", "Message Data"=variant} ("Message Cluster"), "Message"="Simulate_inst_conc", "Message Data"=w2362) -> (w2366:T4)
        n941 = Enqueue Element(queue=w2365, element=w2366, error in (no error)=w2364) -> (error out=w2363:errorcluster)  [unwired: 1 in, 2 out]
      }
      event "Inst_alm_thresh": Value Change {
        n942 = event-data() -> ("NewVal"=w2369:i32)  [unwired: 1 in]
        n943 = Bundle(cluster=T4 {"Message"="", "Message Data"=variant} ("Message Cluster"), "Message"="Inst_alm_thresh", "Message Data"=w2369) -> (w2373:T4)
        n944 = Enqueue Element(queue=w2372, element=w2373, error in (no error)=w2371) -> (error out=w2370:errorcluster)  [unwired: 1 in, 2 out]
      }
      event "3hr_alm_thresh": Value Change {
        n945 = event-data() -> ("NewVal"=w2376:i32)  [unwired: 1 in]
        n946 = Bundle(cluster=T4 {"Message"="", "Message Data"=variant} ("Message Cluster"), "Message"="3hr_alm_thresh", "Message Data"=w2376) -> (w2380:T4)
        n947 = Enqueue Element(queue=w2379, element=w2380, error in (no error)=w2378) -> (error out=w2377:errorcluster)  [unwired: 1 in, 2 out]
      }
      event "Simulate 3hr Average Conc": Value Change {
        n948 = event-data() -> ("NewVal"=w2383:dbl)  [unwired: 1 in]
        n949 = Bundle(cluster=T4 {"Message"="", "Message Data"=variant} ("Message Cluster"), "Message"="Simulate_3hr_av_conc", "Message Data"=w2383) -> (w2387:T4)
        n950 = Enqueue Element(queue=w2386, element=w2387, error in (no error)=w2385) -> (error out=w2384:errorcluster)  [unwired: 1 in, 2 out]
      }
      event "cRIO File IO Stop\n(USB Flash Drive Unmount)": Value Change {
        n951 = event-data() -> ("NewVal"=w2390:bool)  [unwired: 1 in]
        n952 = Bundle(cluster=T4 {"Message"="", "Message Data"=variant} ("Message Cluster"), "Message"="Stop File Write", "Message Data"=w2390) -> (w2394:T4)
        n953 = Enqueue Element(queue=w2393, element=w2394, error in (no error)=w2392) -> (error out=w2391:errorcluster)  [unwired: 1 in, 2 out]
      }
      event "Confirm Flight Number": Value Change {
        n954 = event-data() -> ()  [unwired: 1 in, 5 out]
        n955 = flat-sequence {
          tunnel: w2400 -> [w2403]
          tunnel: w2401 -> [w2404]
          tunnel: [w2404] -> w2398
          tunnel: [w2403] -> w2397
          tunnel: [w2406] -> w2399
          tunnel: w2398 -> [w2408]
          tunnel: w2397 -> [w2407]
          frame #0 {
            n956 = local write "cRIO File IO Stop\n(USB Flash Drive Unmount)"(FALSE ("cRIO File IO Stop\n(USB Flash Drive Unmount)")) -> ()
          }
          frame #1 {
            n957 = local read "Flight Number"() -> (w2405:string)
            n958 = Bundle(cluster=T4 {"Message"="", "Message Data"=variant} ("Message Cluster"), "Message"="Flight Number", "Message Data"=w2405) -> (w2409:T4)
            n959 = Enqueue Element(queue=w2408, element=w2409, error in (no error)=w2407) -> (error out=w2406:errorcluster)  [unwired: 1 in, 2 out]
          }
        }
      }
    }
    "2BOzone Event error out" <- w2344
  }
  n960 = while {
    tunnel: w25 -> [w2419]
    shift-right: [w2414] -> _
    shift-left: w20 -> [w2416]
    shift-right: [w2412] -> w17
    shift-left: w21 -> [w2418]
    tunnel: w18 -> [w2413]
    stop <- w2412 stop-if-true
    # "2BOzone UI Command Sender"
    n961 = Dequeue Element(queue=w2419, error in (no error)=w2413) -> (element=w2415:T4)  [unwired: 1 in, 3 out]
    n962 = Unbundle By Name(w2415) -> ("Message"=w2417:string)
    n963 = case shown="\"3hr_alm_thresh\"" w2417 {
      tunnel: w2418 -> [w2420 w2424 w2431 w2438 w2445 w2452 w2459 w2466 w2473]
      tunnel: w2416 -> [w2421 w2427 w2434 w2441 w2448 w2455 w2462 w2469 w2476]
      tunnel: w2415 -> [_ w2426 w2433 w2440 w2447 w2454 w2461 w2468 w2475]
      tunnel: [w2420 w2423 w2430 w2437 w2444 w2451 w2458 w2465 w2472] -> w2412
      tunnel: [w2421 w2422 w2429 w2436 w2443 w2450 w2457 w2464 w2471] -> w2414
      frame "False", Default {
      }
      frame "Ambient/Cabin" {
        n964 = shared-variable-write(w2427, w2424, w2426) -> (w2425:refnum<k21>, w2428:errorcluster)  [unwired: 1 in, 1 out]
        n965 = Flush Stream(8:w2428, 11:w2425) -> (0:w2423:errorcluster, 3:w2422:refnum<k21>)  [unwired: 2 in, 1 out]
      }
      frame "Simulate_conc" {
        n966 = shared-variable-write(w2434, w2431, w2433) -> (w2432:refnum<k21>, w2435:errorcluster)  [unwired: 1 in, 1 out]
        n967 = Flush Stream(8:w2435, 11:w2432) -> (0:w2430:errorcluster, 3:w2429:refnum<k21>)  [unwired: 2 in, 1 out]
      }
      frame "Simulate_inst_conc" {
        n968 = shared-variable-write(w2441, w2438, w2440) -> (w2439:refnum<k21>, w2442:errorcluster)  [unwired: 1 in, 1 out]
        n969 = Flush Stream(8:w2442, 11:w2439) -> (0:w2437:errorcluster, 3:w2436:refnum<k21>)  [unwired: 2 in, 1 out]
      }
      frame "Inst_alm_thresh" {
        n970 = shared-variable-write(w2448, w2445, w2447) -> (w2446:refnum<k21>, w2449:errorcluster)  [unwired: 1 in, 1 out]
        n971 = Flush Stream(8:w2449, 11:w2446) -> (0:w2444:errorcluster, 3:w2443:refnum<k21>)  [unwired: 2 in, 1 out]
      }
      frame "3hr_alm_thresh" {
        n972 = shared-variable-write(w2455, w2452, w2454) -> (w2453:refnum<k21>, w2456:errorcluster)  [unwired: 1 in, 1 out]
        n973 = Flush Stream(8:w2456, 11:w2453) -> (0:w2451:errorcluster, 3:w2450:refnum<k21>)  [unwired: 2 in, 1 out]
      }
      frame "Simulate_3hr_av_conc" {
        n974 = shared-variable-write(w2462, w2459, w2461) -> (w2460:refnum<k21>, w2463:errorcluster)  [unwired: 1 in, 1 out]
        n975 = Flush Stream(8:w2463, 11:w2460) -> (0:w2458:errorcluster, 3:w2457:refnum<k21>)  [unwired: 2 in, 1 out]
      }
      frame "Stop File Write" {
        n976 = shared-variable-write(w2469, w2466, w2468) -> (w2467:refnum<k21>, w2470:errorcluster)  [unwired: 1 in, 1 out]
        n977 = Flush Stream(8:w2470, 11:w2467) -> (0:w2465:errorcluster, 3:w2464:refnum<k21>)  [unwired: 2 in, 1 out]
      }
      frame "Flight Number" {
        n978 = shared-variable-write(w2476, w2473, w2475) -> (w2474:refnum<k21>, w2477:errorcluster)  [unwired: 1 in, 1 out]
        n979 = Flush Stream(8:w2477, 11:w2474) -> (0:w2472:errorcluster, 3:w2471:refnum<k21>)  [unwired: 2 in, 1 out]
      }
    }
  }
  "2BOzone command sender error out" <- w17
